vi "FIB MAIN (DESKTOP-J3Q0JMJ's conflicted copy 2019-02-19).vi"() -> ()   [LabVIEW 2018]
uses:
  <vilib>/userdefined/High Color/IMAQdx.ctl
  STAGE POSITION.ctl
  Original FIB Source/CENTER STIGMATOR.ctl
  FIB EVENTS.ctl
  FIB CAMERA EVENTS.ctl
  <vilib>/vision/driver/IMAQdx.llb/IMAQdx Buffer Number Mode.ctl
  <vilib>/vision/driver/IMAQdx.llb/IMAQdx Camera Control Mode.ctl
  <vilib>/Instr/_visa.llb/VISA Flush IO Buffer Mask.ctl
  <vilib>/Utility/error.llb/whitespace.ctl
  Mikrodaq/HYMOD MAIA/ddd.ctl
  FIB STAGE EVENTS.ctl
  <vilib>/Instr/_visa.llb/VISA Configure Serial Port (Instr).vi
  <vilib>/vision/driver/NI_Vision_Acquisition_Software.lvlib
  <resource>/objmgr/imaqdx.rc
  <vilib>/vision/NI_Vision_Development_Module.lvlib
  <vilib>/Utility/Variable/NI_VariableUtilities.lvlib
panel:
  out "size(s) 5":i32
  in  "ENABLE APERTURES":bool
  in  "ENABLE ORSAY":bool=TRUE
  in  "ENABLE CAMERA":bool
  out "size(s) 4":i32
  in  "Tab Control 4":enum32{"COMMANDS", "HV RAMPS"}(tab)
  in  "1V ENERGY RAMP":bool
  out "TEST OUTPUT":string
  in  "TEST COMMAND":bool
  in  "TEST COMMAND":string
  out "SERIAL \nRESPONSE":string[](array[string])
  out "WARNING":string
  out "PROCESS":string
  out "PROCESSES":string[](array[string])
  out "BEAM RAMP":dbl[unit][](graph)
  out "EXTRACTOR RAMP":dbl[unit][](graph)
  out "SUPPRESSOR RAMP":dbl[unit][](graph)
  in  "Tab Control 3":T1(tab)
  out "CURRENT":dbl[unit] format="%_4g"
  out "VOLTAGE":dbl[unit] format="%_4g"
  out "BEAM VOLTAGE":dbl[unit](graph)
  out "BEAM CURRENT":dbl[unit](graph)
  out "VOLTAGE":dbl[unit] format="%_4g"
  out "CURRENT":dbl[unit] format="%_4g"
  out "EXTRACTOR":dbl[unit](graph)
  out "EXTRACTOR  CURRENT":dbl[unit](graph)
  out "VOLTAGE":dbl[unit] format="%_4g"
  out "CURRENT":dbl[unit] format="%_4g"
  out "SUPPRESSOR VOLTAGE":dbl[unit](graph)
  out "SUPPRESSOR CURRENT":dbl[unit](graph)
  out "CONDENSOR VOLTAGE":dbl[unit](graph)
  out "CONDENSOR CURRENT":dbl[unit](graph)
  out "OBJECTIVE VOLTAGE":dbl[unit](graph)
  out "OBJECTIVE CURRENT":dbl[unit](graph)
  out "HV SUPPLY FEEDBACK 13":dbl[unit](graph)
  out "HV SUPPLY FEEDBACK 12":dbl[unit](graph)
  in  "IGAIN":dbl=0.00039 format="%_3p"
  in  "IOFFSET":dbl format="%_4g"
  in  "VOFFSET":dbl format="%_4g"
  out "HEATING CURRENT":dbl
  out "HEATING VOLTAGE":dbl
  in  "VGAIN":dbl=0.00071 format="%_3p"
  in  "OFFSET":dbl
  in  "RPONT":dbl[unit]
  in  "RMES":dbl[unit]
  out "TIMER":u32
  out "size(s)":i32
  out "SUPPRESSOR RAMP":dbl[unit][](array[numeric])
  out "EXTRACTOR RAMP":dbl[unit][](array[numeric])
  out "BEAM RAMP":dbl[unit][](array[numeric])
  in  "MEASURE HV":bool
  out "SERIAL \nRESPONSE 2":string[](array[string])
  out "VISA ERROR":errorcluster
  out "BEAM CURRENT (FC2)":dbl[unit] format="%_4g"
  out "BEAM CURRENT (FC1)":dbl[unit] format="%_4g"
  in  "APERTURE (MASS)":u16(ring)=3 items=["10 um", "20 um", "50 um", "50 um", "100 um", "200 um", "400 um"]
  in  "BRIGHT,CONT,GAMMA":cluster{"B":dbl, "C":dbl, "G":dbl}={"B"=250.0, "C"=67.0, "G"=1.6000000000000005} {"G" format="%_4g"; "C" format="%_4g"; "B" format="%_4g"}
  in  "REFLECTIVITY":bool
  in  "ROTATE VIEW":bool
  in  "ANGLE":sgl format="%.2f"
  in  "IMAGE SYMMETRY":u32(ring)=2 items=["Horizontal", "Vertical", "CENTRAL", "1st Diagonal", "2nd Diagonal"]
  in  "SYMMETRY":bool
  out "FIB CAMERA ERROR":errorcluster
  out "FIB SAMPLE CAMERA":T2="CSIRO-SAMPLE" caption="Session Out"
  out "IMAGE YCENTRE":dbl
  out "IMAGE XCENTRE":dbl
  out "ActualPeakBandwidth":dbl=1000.0
  out "IMAGE YPIXELS":u32=1024
  out "IMAGE XPIXELS":u32=1360
  in  "START SCANNING":bool
  in  "STOP":bool
  out "INTERLOCK STATE":bool
  in  "BEAM ON":bool=TRUE
  in  "BLANKING CONTROL":u16(ring) items=["LOCAL ", "SOURCE", "EXTERNAL"]
  in  "FIB SETUP FILE":path=path "C:/Users/jamie/Desktop/test.tdms"
  in  "SAVE SETUP":bool
  in  "READ & APPLY SETUP":bool
  in  "OBJECT APERTURE":u16(ring)=3 items=["10 um", "20 um", "50 um", "50 um", "100 um", "200 um", "400 um"]
  in  "USER":string="jslaird"
  in  "COMMENT":string
  in  "NAME":string
  out "gamme":bool
  out "Image":T3(plugin-control)
  in  "Tab Control":T4(tab)
  in  "RESET":bool
  in  "INTERLOCK HV":bool
  out "HIGH ENERGY":bool
  in  "SETTINGS DELAY":dbl[unit]=0.2
  in  "dV ENERGY":dbl[unit]=250.0
  in  "dV SUPPRESS":dbl[unit]=50.0
  in  "SHUTDOWN":bool
  in  "FILAMENT":bool
  out "HIGH VOLTAGE SUPPLIES":cluster{dbl[unit], dbl[unit], dbl[unit]}(knob)={0.0, 103.78830891166923, 181.50345045415557} scale format="%#_6p"
  in  "ION GUN":bool
  in  "FILAMENT HEATING":dbl[unit](slide) min=0.0 max=5.0 step=0.1 scale=0.0..5.000000000000001
  in  "ION GUN SETTINGS":T5 {"ION CURRENT" min=0 max=3e-05 step=1e-07; "SUPPRESSOR" min=0 max=30000 step=100; "EXTRACTOR" min=0 max=12000 step=100; "BEAM ENERGY" min=0 max=30000 step=1000}
  in  "dV EXTRACTOR":dbl[unit]=50.0
  in  "MOVE 2 POSITION":T6 {"Z" format="%_4g"; "Y" format="%_4g"; "X" format="%_4g"}
  out "POSITION":T6 {"Z" format="%_4g"; "Y" format="%_4g"; "X" format="%_4g"}
  in  "EXPOSURE":dbl(slide)=106.26827541712952 min=1.0 max=2500.0 step=10.0 scale=5.0..1000.0 scale format="%#_3f"
  out "FIB CAMERA":T3(plugin-control)
  out "IP ADDRESS":string="192.168.1.10"
  in  "CONFIGS":u16(ring) items=["MANUAL", "BEAM FOCUS", "SAMPLE VIEWING"]
  in  "GAIN METHOD":u16(ring)=2 items=["OFF", "ONCE", "CONTINOUS"]
  in  "GAIN":sgl=1.0 min=0 max=31 step=1
  out "CENTRE CAMERA FOV":T7={"Numeric Control"=677, "Numeric Control"=510}
  in  "Tab Control 2":T8(tab)
  out "Yo":dbl format="%_3g"
  out "Xo":dbl format="%_3g"
  in  "STORE OBJECT":bool
  in  "WOBBLER SETTINBGS FOR OBJECT ALIGNMENT":T9={"WOBBLER AMPLITUDE"={0.0, 33.333523, 47.735184}, "WOBBLE"=1} {"WOBBLE" items=["ENERGY", "CONDENSOR", "OBJECTIVE"]; "WOBBLER AMPLITUDE" scale=0.0..100.0}
  in  "OBJ APERTURE ALIGNMENT":T10={"DOWN"=FALSE, "UP"=FALSE, "STEP SIZE"=1, "LEFT"=FALSE, "RIGHT"=FALSE} {"STEP SIZE" items=["1 um", "5 um", "20 um", "50 um", "100 um", "500 um", "2000 um"]}
  in  "TURN ON WOBBLER":bool
  in  "OBJECT APERTURE POSITIONS":cluster{"NAME":string, "Xo":dbl, "Yo":dbl}[](array[cluster])=[{"NAME"="10um", "Xo"=0.0, "Yo"=0.0}, {"NAME"="20um", "Xo"=0.0, "Yo"=0.0}, {"NAME"="50um", "Xo"=0.0, "Yo"=0.0}, {"NAME"="50um", "Xo"=0.0, "Yo"=0.0}, {"NAME"="100um", "Xo"=0.0, "Yo"=0.0}, {"NAME"="200um", "Xo"=0.0, "Yo"=0.0}, {"NAME"="400um", "Xo"=0.0, "Yo"=0.0}] {"Yo" format="%_3g"; "Xo" format="%_3g"}
  in  "MASS APERTURE POSITIONS":cluster{"NAME":string, "Xa":dbl, "Ya":dbl}[](array[cluster])=[{"NAME"="10um", "Xa"=0.0, "Ya"=0.0}, {"NAME"="20um", "Xa"=0.0, "Ya"=0.0}, {"NAME"="50um", "Xa"=0.0, "Ya"=0.0}, {"NAME"="50um", "Xa"=0.0, "Ya"=0.0}, {"NAME"="100um", "Xa"=0.0, "Ya"=0.0}, {"NAME"="200um", "Xa"=0.0, "Ya"=0.0}, {"NAME"="400um", "Xa"=0.0, "Ya"=0.0}] {"Ya" format="%_3g"; "Xa" format="%_3g"}
  in  "MASS APERTURE ALIGNMENT":T10={"DOWN"=FALSE, "UP"=FALSE, "STEP SIZE"=1, "LEFT"=FALSE, "RIGHT"=FALSE} {"STEP SIZE" items=["1 um", "5 um", "20 um", "50 um", "100 um", "500 um", "2000 um"]}
  out "Xa":dbl format="%_3g"
  out "Ya":dbl format="%_3g"
  in  "STORE APERTURE":bool
  out "REFERENCED":bool[](array[boolean])
  out "ON TRARGET":bool[](array[boolean])
  in  "INIT PI":bool
  in  "STAGE AXES":string[](array[string])=["1", "2"]
  out "VELOCITIES":dbl[](array[numeric])
  out "POSITIONS":dbl[](array[numeric]) format="%_5g"
  out "STATUS":bool
  in  "HOME ALL AXES":bool
  in  "AXES MOTIION SETTINGS":dbl[][](array[numeric])=[[1.0, 140.0, 5.0, 350.0, 1200.0, 10000.0, 100.0, 30000.0, 200.0], [2.0, 140.0, 5.0, 350.0, 1200.0, 10000.0, 100.0, 30000.0, 200.0], [3.0, 140.0, 5.0, 0.0, 1200.0, 10000.0, 100.0, 30000.0, 200.0], [4.0, 140.0, 5.0, 0.0, 0.0, 10000.0, 100.0, 30000.0, 200.0]]
  out "NO CONTROLLER":bool
  in  "HOME ON LIMIT":u16(ring) items=["POSITIVE", "NEGATIVE"]
  out "RANGE":dbl[](array[numeric]) format="%_5g"
  in  "STIGMATOR":T11 {"STIG ALIGN"."-Y" min=-100 max=100 step=0.1 scale=-100.0..100.0; "STIG ALIGN"."+Y" min=-100 max=100 step=0.1 scale=-100.0..100.0; "STIG ALIGN"."-X" min=-100 max=100 step=0.1 scale=-100.0..100.0; "STIG ALIGN"."+X" min=-100 max=100 step=0.1 scale=-100.0..100.0; "THETA" format="%_3g"; "OFFY" format="%_3g"; "OFFX" format="%_3g"; "STIG Y" format="%_3g"; "STIG X" format="%_3g"}
  in  "STIGMATOR X & Y":cluster{"X":sgl, "Y":sgl} {"Y" min=0 max=20000 step=100 scale=0.0..1000.0; "X" min=0 max=20 step=0.1 scale=0.0..20.0}
  out "OBJECTIVE":sgl[unit] format="%_4g"
  out "CONDENSOR":sgl[unit] format="%_4g"
  in  "OBJECTIVE":cluster{"COARSE":sgl[unit], "FINE":sgl[unit]} {"FINE" min=0 max=20000 step=100 scale=0.0..1000.0; "COARSE" min=0 max=20000 step=100}
  in  "CONDENSOR":cluster{"COARSE":sgl[unit], "FINE":sgl[unit]} {"FINE" min=0 max=20000 step=100 scale=1.0..1000.0; "COARSE" min=0 max=20000 step=100}
  in  "SCAN CENTRE ON STAGE":T12 {"Zs" format="%_2g"; "Xs" format="%_2g"; "Ys" format="%_2g"}
  in  "STAGE POSITION":T12 {"Zs" format="%_2g"; "Xs" format="%_2g"; "Ys" format="%_2g"}
  in  "SCANNING CLUSTER":T13 {"MAGNIFICATION" scale=-180.0..180.0; "Y-OFFSET" min=0 max=3e-05 step=1e-07; "X-OFFSET" min=0 max=3e-05 step=1e-07; "SCANNING TYPE" items=["EXTERNAL", "ION MILLING"]}
  in  "EXTERNAL SCANNING ROI":T14={"X-AMPLITUDE"=1e-07, "dX"=0.0, "Y-AMPLITUDE"=1e-07, "dY"=0.0} {"Y-AMPLITUDE" min=1e-07 max=0.0005 step=9.999999999999999e-06; "X-AMPLITUDE" min=1e-07 max=0.0005 step=9.999999999999999e-06}
  out "CHAMBER VACUUM":cluster{dbl[unit], dbl[unit]}(knob)={2.179544466940017e-05, 0.00030039245125477424} scale format="%#_2e"
  in  "COLUMN THRESHOLD":dbl[unit]=6.666118421052631e-05
  out "VACUUM STATE":bool
  out "COLUMN VACUUM":dbl[unit](graph)
  out "COLUMN VACUUM":cluster{dbl[unit], dbl[unit]}(knob)={8.118323356328827e-09, 0.00010317996118558537} scale format="%#_1e"
  out "150V GOOD":bool
  in  "CHAMBER THRESHOLD":dbl[unit]
  in  "GATE VALVE":bool=TRUE
  in  "TERMINATION":bool=TRUE
  in  "TERMINATION CHAR":u16(ring)=1 items=["NONE", "CR", "LF", "CR+LF"]
  out "APPEND":string
  out "ORSAY CONNECTED":bool
  in  "STARTUP":T15[](array[typedef])=[enum."OPEN SERIAL CONN TO ORSAY", enum."INITIALISE ORSAY", enum."TURN OFF WOBBLER", enum."VACUUM ", enum."CHECK 150V", enum."BLANKING TOGGLE"]
  out "ORSAY":refnum<visa-resource-name>
  # "EXTRACTOR"
  # "CONDENSOR"
  # "OBJECT\nAPERTURES"
  # "OBJECTIVE"
  # "FILAMENT SHOULD BE ON PRIOR TO GUN !"
  # "E"
  # "C"
  # "O"
  # "AXIS               P                        I                      D                      L                  LOW-VEL    LOW-ACC      HI-VEL          HI-ACC"
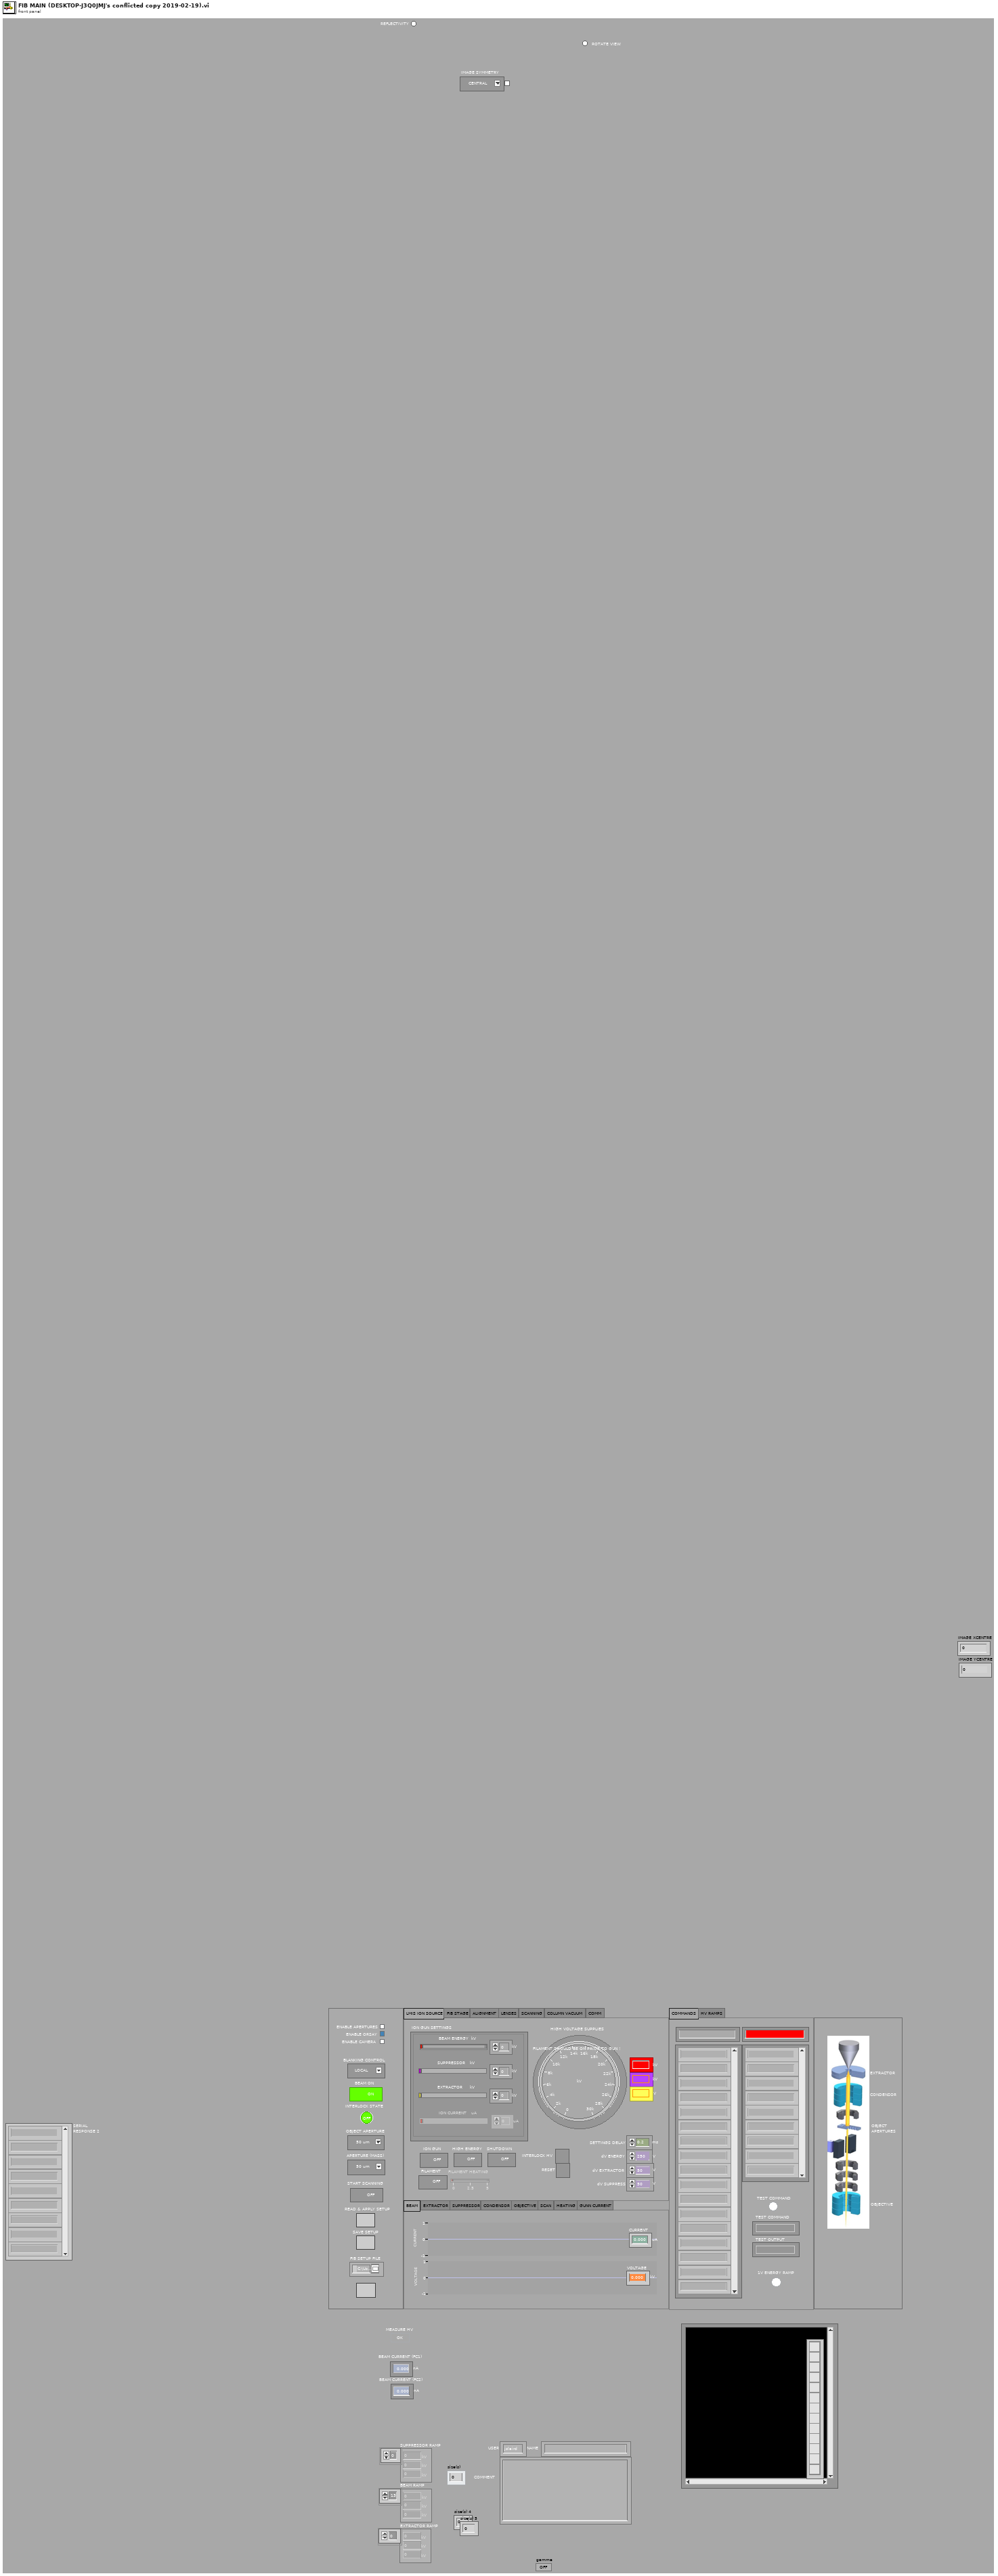
[diagram p1: front panel]
types:
  T1 = enum32{"BEAM", "EXTRACTOR", "SUPPRESSOR", "CONDENSOR", "OBJECTIVE", "SCAN", "HEATING", "GUNN CURRENT"}
  T2 = typedef "IMAQdx.ctl" = refnum<k21>
  T3 = typedef "IMAQ Image.ctl" = refnum<image>
  T4 = enum32{"LMIS ION SOURCE", "FIB STAGE", "ALIGNMENT", "LENSES", "SCANNING", "COLUMN VACUUM", "COMM"}
  T5 = cluster{"BEAM ENERGY":sgl[unit], "SUPPRESSOR":sgl[unit], "EXTRACTOR":sgl[unit], "ION CURRENT":sgl[unit]}
  T6 = typedef "STAGE POSITION.ctl" = cluster{"X":dbl[unit], "Y":dbl[unit], "Z":dbl[unit]}
  T7 = cluster{"Numeric Control":i32, "Numeric Control":i32}
  T8 = enum32{"OBJECTS", "MASS APERTURES", "MOTORS", "CENTRE STIGMATOR"}
  T9 = cluster{"WOBBLER AMPLITUDE":cluster{sgl, sgl, sgl}, "WOBBLE":u16}
  T10 = cluster{"DOWN":bool, "UP":bool, "STEP SIZE":u16, "LEFT":bool, "RIGHT":bool}
  T11 = typedef "CENTER STIGMATOR.ctl" = cluster{"STIG ALIGN":cluster{"+X":sgl, "-X":sgl, "+Y":sgl, "-Y":sgl}, "STIG X":dbl, "OFFX":dbl, "STIG Y":dbl, "OFFY":dbl, "THETA":dbl}
  T12 = cluster{"Xs":dbl[unit], "Ys":dbl[unit], "Zs":dbl[unit]}
  T13 = cluster{"SCANNING TYPE":u16, "X-OFFSET":sgl[unit], "Y-OFFSET":sgl[unit], "ROTATION":dbl[unit], "MAGNIFICATION":dbl}
  T14 = cluster{"X-AMPLITUDE":dbl[unit], "dX":dbl[unit], "Y-AMPLITUDE":dbl[unit], "dY":dbl[unit]}
  T15 = typedef "FIB EVENTS.ctl" = enum16{"LOOP", "OPEN SERIAL CONN TO ORSAY", "INITIALISE ORSAY", "READ SETTINGS", "SAVE SETTINGS", "OBJECTIVE LENS", "CONDENSOR LENS", "BLANKING TOGGLE", "TURN ON HEATER", "TURN OFF WOBBLER", "MEASURE HEATER OUTPUT", "TOGGLE GATE VALVE", "SCANNING CONTROLS", "TURN ON BEAM HV", "ENERGY RAMP CYCLE", "TURN ON SUPPRESSOR", "TURN ON EXTRACTOR", "SET ENERGY RANGE", "MEASURE HV SUPPLY VOLTAGES", "SHUTDOWN ION SOURCE", "RESET TYPE II", "PROBE CURRENT FC#1", "PROBE CURRENT FC#2", "VACUUM ", "CHECK 150V", "INITIALISE PI MOTORS", "SET STIGMATOR", "SET WOBBLER FOR OBJECT", "SET OBJ & AP STAGE VELOCITIES", "READ APERTURE POSITIONS", "HOME OBJ & AP STAGES", "DEFINE NEW OBJ", "MOVE OBJ STAGES", "DEFINE NEW APERTURE", "MOVE APERTURE STAGES", "STOP SYSTEM", "TEST COMMANDS"}
  T16 = typedef "FIB CAMERA EVENTS.ctl" = enum16{"INIT VIDEO", "CAMERA GAIN", "CAMERA EXPOSURE", "LOOP"}
  T17 = enum8{"Enabled", "Disabled", "Disabled and Grayed Out"}
  T18 = cluster{"BEAM ENERGY":sgl[unit], "EXTRACTOR":sgl[unit], "SUPPRESSOR":sgl[unit], "ION CURRENT":sgl[unit]}
  T19 = typedef "FIB STAGE EVENTS.ctl" = enum16{"LOOP", "INIT STAGE CONTROLLER", "SEND COMMAND TO CONTROLLER", "HOME X", "HOME Y", "HOME Z", "ABORT ALL AXES", "GOTO MARKER", "ZERO XYZ", "READ XYZ POSITIONS", "GOTO XYZ POSITION", "STOP", "JOG XYZ", "WAIT FOR MOVE COMPLETE"}
  T20 = cluster{"BEAM":dbl[unit], "SUPPRESSOR":dbl[unit], "EXTRACTOR":dbl[unit]}
  T21 = typedef "ddd.ctl" = string[]
  T22 = enum16{"open", "open or create", "create or replace", "create", "open (read-only)"}
  T23 = typedef "VISA Flush IO Buffer Mask.ctl" = u16
  T24 = cluster{dbl[unit], "CHAMBER THRESHOLD":dbl[unit]}
  T25 = typedef "whitespace.ctl" = u16
  T26 = typedef "NI_Vision_Acquisition_Software.lvlib/IMAQdx Buffer Number Mode.ctl" = enum32{"Next", "Last", "Buffer Number", "Every", "Last New"}
  T27 = typedef "NI_Vision_Acquisition_Software.lvlib/IMAQdx Camera Control Mode.ctl" = enum32{"Controller", "Listener"}
  T28 = typedef "Image Type" = u32
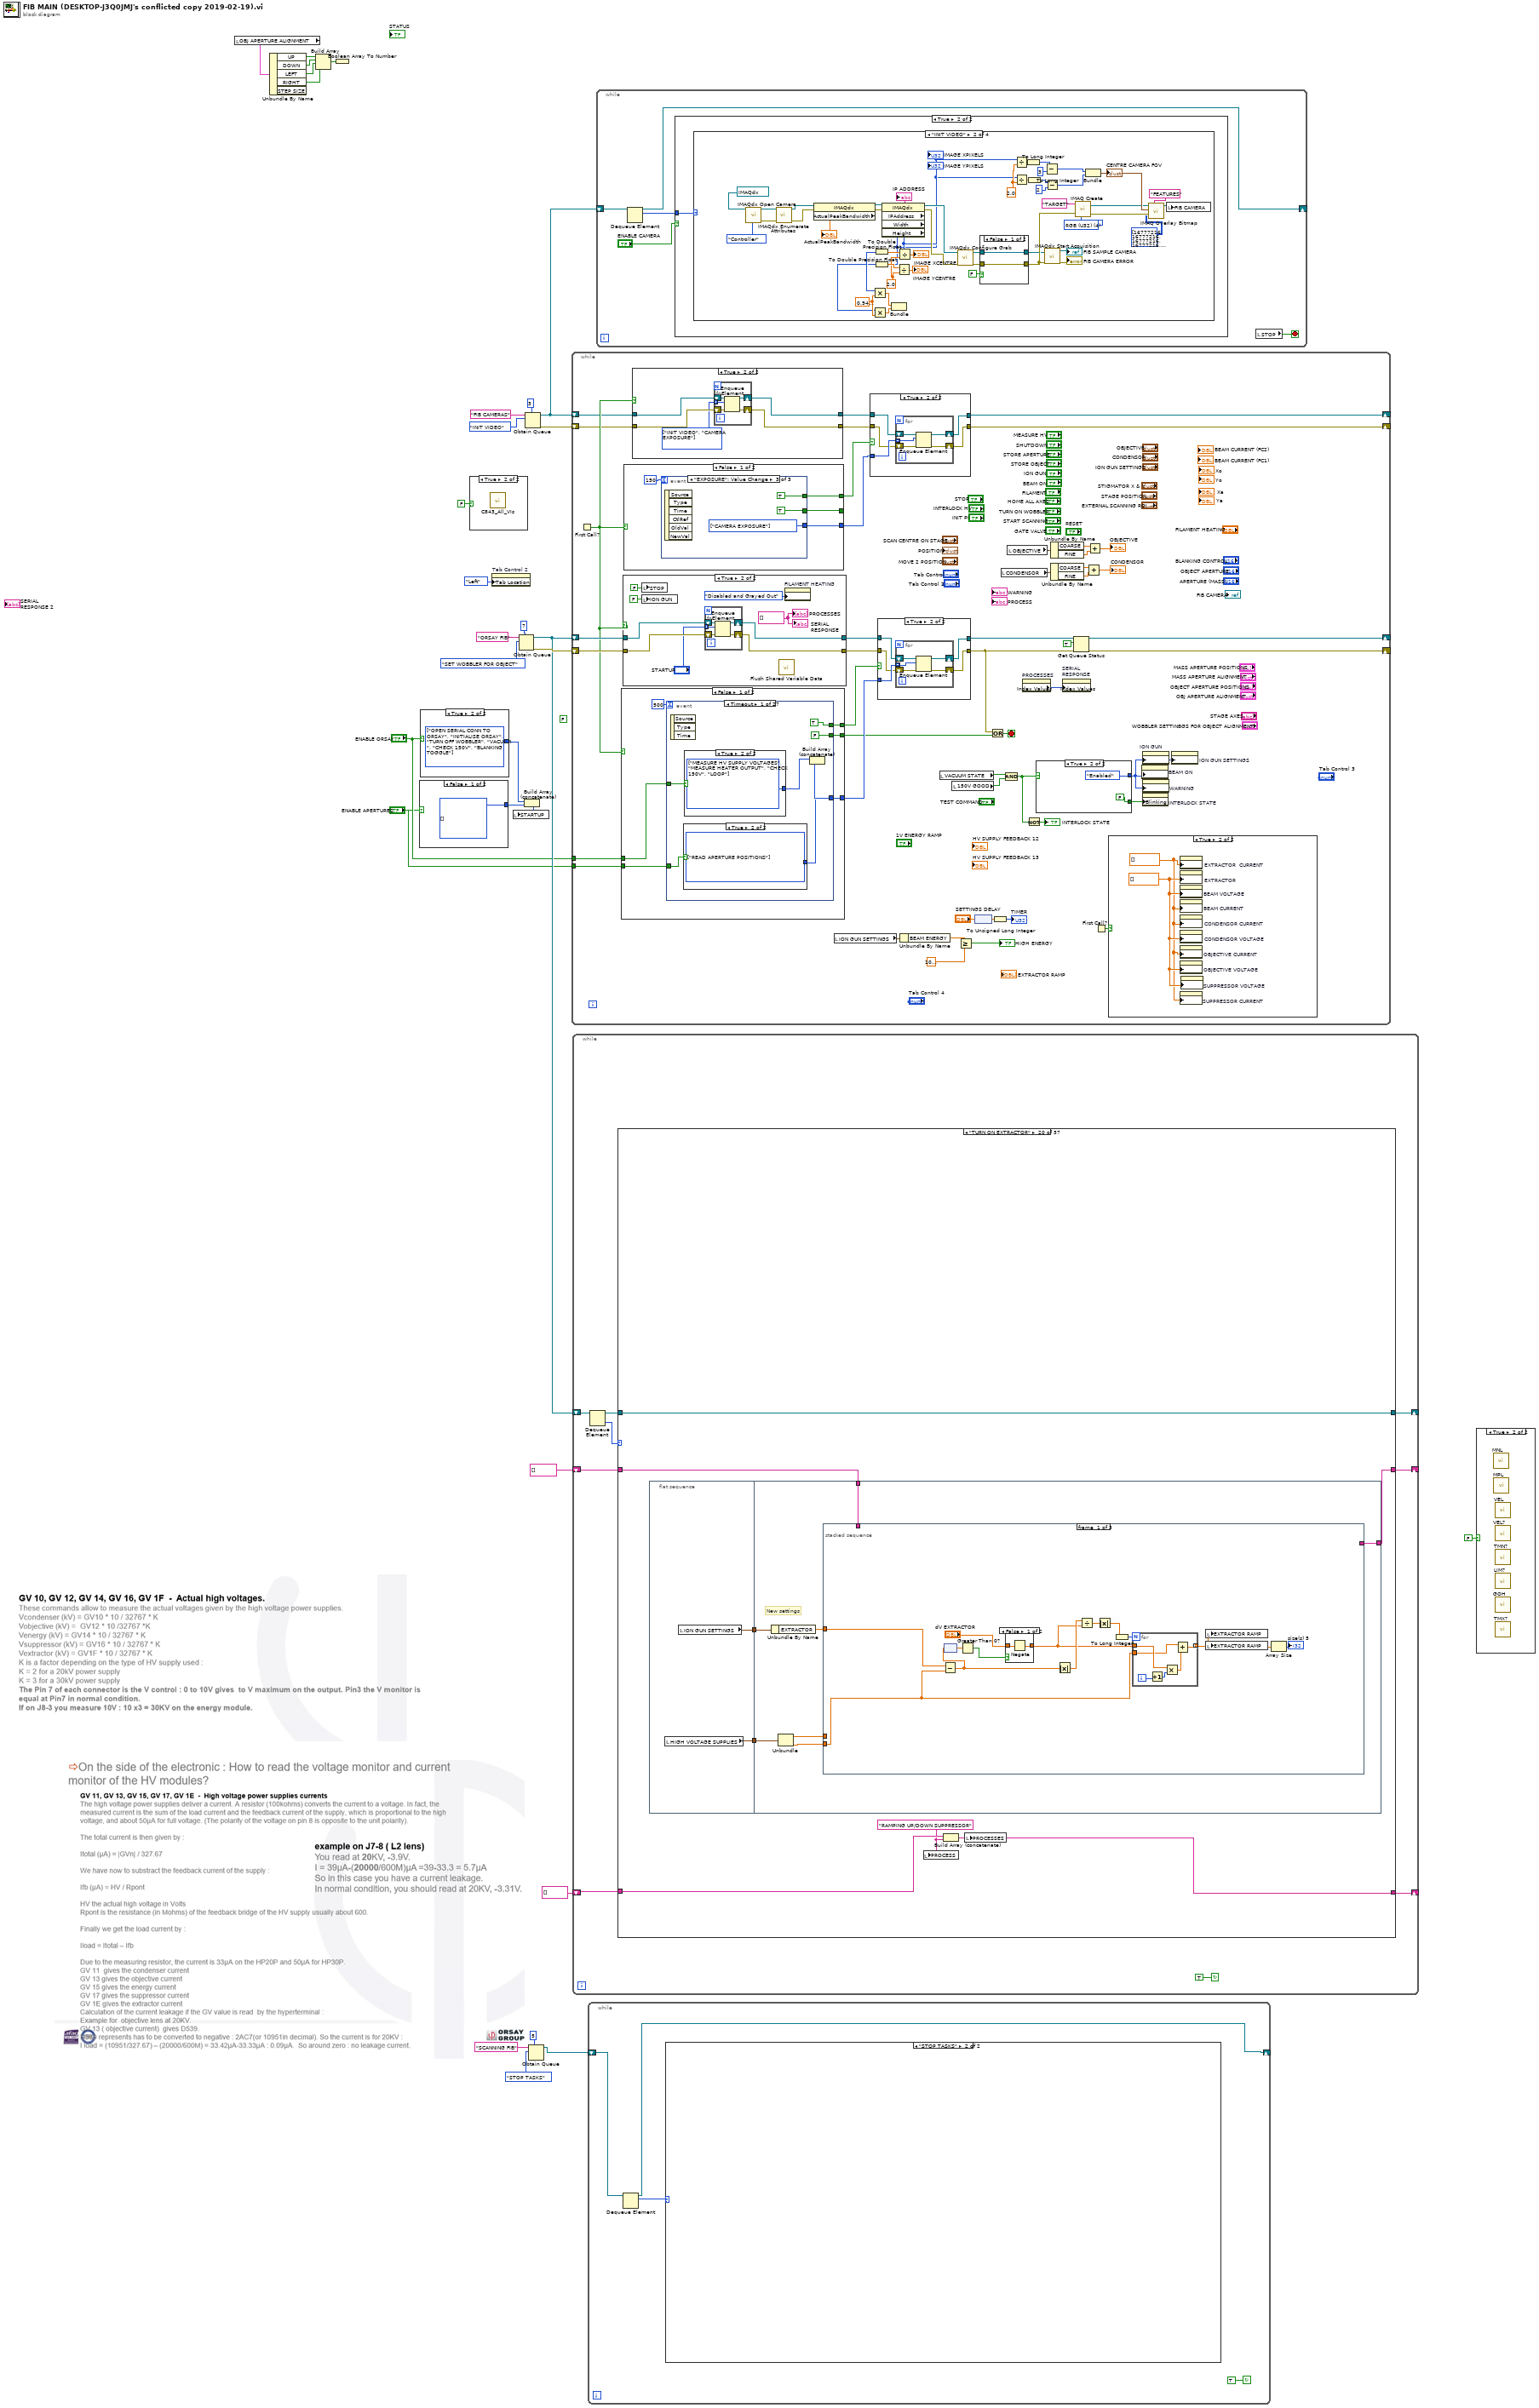
[diagram p0: block diagram]
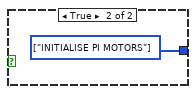
[diagram p2: hidden frame]
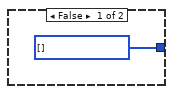
[diagram p3: hidden frame]
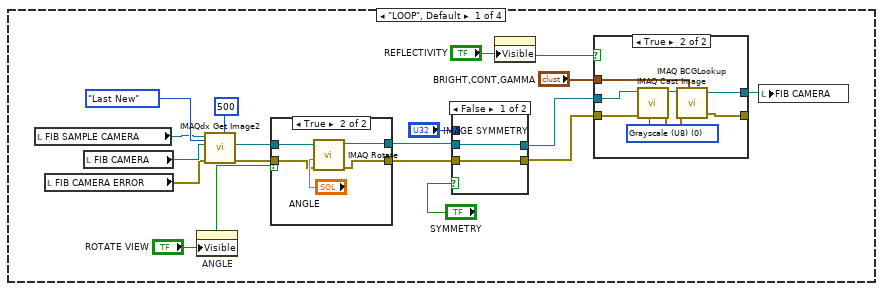
[diagram p8: hidden frame]
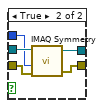
[diagram p11: hidden frame]
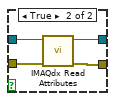
[diagram p12: hidden frame]
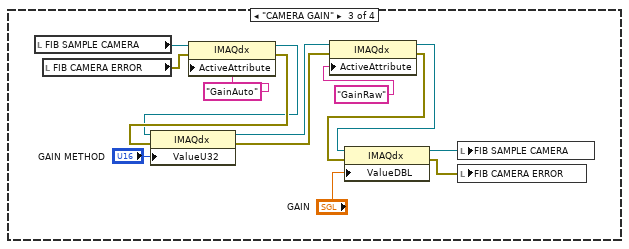
[diagram p13: hidden frame]
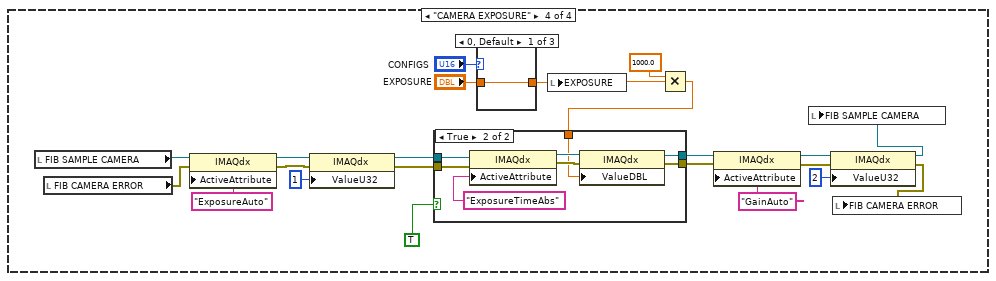
[diagram p14: hidden frame]
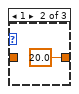
[diagram p16: hidden frame]
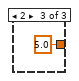
[diagram p17: hidden frame]
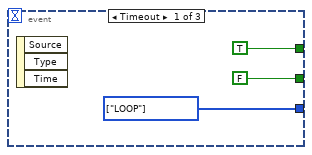
[diagram p20: hidden frame]
diagram:
  (unwired) FALSE ("ION GUN")
  n1 = local read "OBJ APERTURE ALIGNMENT"() -> (w17:T10)
  n2 = Unbundle By Name(w17) -> ("UP"=w18:bool, "DOWN"=w19:bool, "LEFT"=w20:bool, "RIGHT"=w21:bool)  [unwired: 1 out]
  n3 = Build Array(w18, w19, w20, w21) -> (w22:bool[])
  n4 = Boolean Array To Number(Boolean array=w22) -> ()  [unwired: 1 out]
  n5 = case shown="False" "ENABLE APERTURES" {
    tunnel: [w31 w32] -> w4
    frame False {
      w31 = T15[] [] items=["LOOP", "OPEN SERIAL CONN TO ORSAY", "INITIALISE ORSAY", "READ SETTINGS", "SAVE SETTINGS", "OBJECTIVE LENS", "CONDENSOR LENS", "BLANKING TOGGLE", "TURN ON HEATER", "TURN OFF WOBBLER", "MEASURE HEATER OUTPUT", "TOGGLE GATE VALVE", "SCANNING CONTROLS", "TURN ON BEAM HV", "ENERGY RAMP CYCLE", "TURN ON SUPPRESSOR", "TURN ON EXTRACTOR", "SET ENERGY RANGE", "MEASURE HV SUPPLY VOLTAGES", "SHUTDOWN ION SOURCE", "RESET TYPE II", "PROBE CURRENT FC#1", "PROBE CURRENT FC#2", "VACUUM ", "CHECK 150V", "INITIALISE PI MOTORS", "SET STIGMATOR", "SET WOBBLER FOR OBJECT", "SET OBJ & AP STAGE VELOCITIES", "READ APERTURE POSITIONS", "HOME OBJ & AP STAGES", "DEFINE NEW OBJ", "MOVE OBJ STAGES", "DEFINE NEW APERTURE", "MOVE APERTURE STAGES", "STOP SYSTEM", "TEST COMMANDS"] ("STARTUP")
    }
    frame True {
      w32 = T15[] [enum."INITIALISE PI MOTORS"] items=["LOOP", "OPEN SERIAL CONN TO ORSAY", "INITIALISE ORSAY", "READ SETTINGS", "SAVE SETTINGS", "OBJECTIVE LENS", "CONDENSOR LENS", "BLANKING TOGGLE", "TURN ON HEATER", "TURN OFF WOBBLER", "MEASURE HEATER OUTPUT", "TOGGLE GATE VALVE", "SCANNING CONTROLS", "TURN ON BEAM HV", "ENERGY RAMP CYCLE", "TURN ON SUPPRESSOR", "TURN ON EXTRACTOR", "SET ENERGY RANGE", "MEASURE HV SUPPLY VOLTAGES", "SHUTDOWN ION SOURCE", "RESET TYPE II", "PROBE CURRENT FC#1", "PROBE CURRENT FC#2", "VACUUM ", "CHECK 150V", "INITIALISE PI MOTORS", "SET STIGMATOR", "SET WOBBLER FOR OBJECT", "SET OBJ & AP STAGE VELOCITIES", "READ APERTURE POSITIONS", "HOME OBJ & AP STAGES", "DEFINE NEW OBJ", "MOVE OBJ STAGES", "DEFINE NEW APERTURE", "MOVE APERTURE STAGES", "STOP SYSTEM", "TEST COMMANDS"] ("STARTUP")
    }
  }
  n6 = case shown="True" "ENABLE ORSAY" {
    tunnel: [w33 w34] -> w5
    frame False {
      w33 = T15[] [] items=["LOOP", "OPEN SERIAL CONN TO ORSAY", "INITIALISE ORSAY", "READ SETTINGS", "SAVE SETTINGS", "OBJECTIVE LENS", "CONDENSOR LENS", "BLANKING TOGGLE", "TURN ON HEATER", "TURN OFF WOBBLER", "MEASURE HEATER OUTPUT", "TOGGLE GATE VALVE", "SCANNING CONTROLS", "TURN ON BEAM HV", "ENERGY RAMP CYCLE", "TURN ON SUPPRESSOR", "TURN ON EXTRACTOR", "SET ENERGY RANGE", "MEASURE HV SUPPLY VOLTAGES", "SHUTDOWN ION SOURCE", "RESET TYPE II", "PROBE CURRENT FC#1", "PROBE CURRENT FC#2", "VACUUM ", "CHECK 150V", "INITIALISE PI MOTORS", "SET STIGMATOR", "SET WOBBLER FOR OBJECT", "SET OBJ & AP STAGE VELOCITIES", "READ APERTURE POSITIONS", "HOME OBJ & AP STAGES", "DEFINE NEW OBJ", "MOVE OBJ STAGES", "DEFINE NEW APERTURE", "MOVE APERTURE STAGES", "STOP SYSTEM", "TEST COMMANDS"] ("STARTUP")
    }
    frame True {
      w34 = T15[] [enum."OPEN SERIAL CONN TO ORSAY", enum."INITIALISE ORSAY", enum."TURN OFF WOBBLER", enum."VACUUM ", enum."CHECK 150V", enum."BLANKING TOGGLE"] items=["LOOP", "OPEN SERIAL CONN TO ORSAY", "INITIALISE ORSAY", "READ SETTINGS", "SAVE SETTINGS", "OBJECTIVE LENS", "CONDENSOR LENS", "BLANKING TOGGLE", "TURN ON HEATER", "TURN OFF WOBBLER", "MEASURE HEATER OUTPUT", "TOGGLE GATE VALVE", "SCANNING CONTROLS", "TURN ON BEAM HV", "ENERGY RAMP CYCLE", "TURN ON SUPPRESSOR", "TURN ON EXTRACTOR", "SET ENERGY RANGE", "MEASURE HV SUPPLY VOLTAGES", "SHUTDOWN ION SOURCE", "RESET TYPE II", "PROBE CURRENT FC#1", "PROBE CURRENT FC#2", "VACUUM ", "CHECK 150V", "INITIALISE PI MOTORS", "SET STIGMATOR", "SET WOBBLER FOR OBJECT", "SET OBJ & AP STAGE VELOCITIES", "READ APERTURE POSITIONS", "HOME OBJ & AP STAGES", "DEFINE NEW OBJ", "MOVE OBJ STAGES", "DEFINE NEW APERTURE", "MOVE APERTURE STAGES", "STOP SYSTEM", "TEST COMMANDS"] ("STARTUP")
    }
  }
  n7 = case shown="True" FALSE {
    frame False {
    }
    frame True {
      n8 = call "C843_All_VIs.vi"() -> ()  [unwired: 1 in]
    }
  }
  n9 = property on="Tab Control 2" class="TabCtl (strict)"("Tab Location"=enum32{"Top", "Bottom", "Left", "Right"}."Left") -> ()  [unwired: 2 in, 2 out]
  n10 = Obtain Queue(max queue size (-1, unlimited)=7, name (unnamed)="ORSAY FIB", element data type=FIB_EVENTS."SET WOBBLER FOR OBJECT" ("Enum")) -> (queue out=w7:refnum<queue>, error out=w28:errorcluster)  [unwired: 2 in, 1 out]
  n11 = Build Array (concatenate)(w5, w4) -> (w3:T15[])
  n12 = local write "STARTUP"(w3) -> ()
  n13 = Obtain Queue(max queue size (-1, unlimited)=3, name (unnamed)="FIB CAMERAS", element data type=FIB_CAMERA_EVENTS."INIT VIDEO") -> (queue out=w23:refnum<queue>, error out=w24:errorcluster)  [unwired: 2 in, 1 out]
  n14 = Obtain Queue(max queue size (-1, unlimited)=5, name (unnamed)="SCANNING FIB", element data type=enum16{"INIT DAQ", "STOP TASKS"}."STOP TASKS") -> (queue out=w11:refnum<queue>)  [unwired: 2 in, 2 out]
  n15 = while {
    shift-right: [w73] -> _
    shift-left: w7 -> [w81]
    shift-right: [w70] -> _
    shift-left: w28 -> [w80]
    shift-right: [w59] -> _
    shift-left: w23 -> [w65]
    shift-right: [w58] -> _
    shift-left: w24 -> [w64]
    tunnel: "ENABLE ORSAY" -> [w36]
    tunnel: "ENABLE APERTURES" -> [w35]
    stop <- w42 stop-if-true
    n16 = First Call?() -> (First Call?: T/F=w66:bool)
    n17 = case shown="False" w66 {
      tunnel: [w132 FALSE] -> w78
      tunnel: [w131 w242] -> w77
      tunnel: [w130 FALSE] -> w74
      tunnel: w36 -> [w129 _]
      tunnel: w35 -> [w128 _]
      frame False {
        n18 = event shown="[0] Timeout" {
          selector: _ -> [_ _ _ _ _ _ _ _ _ _ _ _ _ _ _ _ _ _ _ _ _ _ _ _ _ _ _]
          dyn-events: _ -> [_ _ _ _ _ _ _ _ _ _ _ _ _ _ _ _ _ _ _ _ _ _ _ _ _ _ _]
          timeout: 500 -> [_ _ _ _ _ _ _ _ _ _ _ _ _ _ _ _ _ _ _ _ _ _ _ _ _ _ _]
          tunnel: [TRUE TRUE ("VACUUM STATE") TRUE ("VACUUM STATE") TRUE ("VACUUM STATE") w156 w158 w164 w168 w175 w182 TRUE ("VACUUM STATE") TRUE ("VACUUM STATE") TRUE ("VACUUM STATE") w196 TRUE ("VACUUM STATE") w201 _ TRUE ("VACUUM STATE") w209 w213 w217 w221 TRUE w227 TRUE ("VACUUM STATE") w234 TRUE ("VACUUM STATE")] -> w132
          tunnel: [FALSE FALSE FALSE FALSE FALSE FALSE FALSE FALSE FALSE FALSE FALSE FALSE FALSE FALSE FALSE FALSE _ FALSE FALSE FALSE FALSE FALSE FALSE FALSE FALSE FALSE FALSE] -> w130
          tunnel: [w137 w147 w148 w153 w154 w162 w165 w171 w178 w180 w185 w188 w191 w194 w200 w204 w205 w206 w212 w216 w220 w223 w226 w228 w230 w233 w236] -> w131
          tunnel: w129 -> [w135 _ _ _ _ _ _ _ _ _ _ _ _ _ _ _ _ _ _ _ _ _ _ _ _ _ _]
          tunnel: w128 -> [w134 _ _ _ _ _ _ _ _ _ _ _ _ _ _ _ _ _ _ _ _ _ _ _ _ _ _]
          event Timeout {
            n19 = event-data() -> ()  [unwired: 1 in, 3 out]
            n20 = case shown="True" w134 {
              tunnel: [w141 w142] -> w136
              frame False {
                w141 = T15[] [] items=["LOOP", "OPEN SERIAL CONN TO ORSAY", "INITIALISE ORSAY", "READ SETTINGS", "SAVE SETTINGS", "OBJECTIVE LENS", "CONDENSOR LENS", "BLANKING TOGGLE", "TURN ON HEATER", "TURN OFF WOBBLER", "MEASURE HEATER OUTPUT", "TOGGLE GATE VALVE", "SCANNING CONTROLS", "TURN ON BEAM HV", "ENERGY RAMP CYCLE", "TURN ON SUPPRESSOR", "TURN ON EXTRACTOR", "SET ENERGY RANGE", "MEASURE HV SUPPLY VOLTAGES", "SHUTDOWN ION SOURCE", "RESET TYPE II", "PROBE CURRENT FC#1", "PROBE CURRENT FC#2", "VACUUM ", "CHECK 150V", "INITIALISE PI MOTORS", "SET STIGMATOR", "SET WOBBLER FOR OBJECT", "SET OBJ & AP STAGE VELOCITIES", "READ APERTURE POSITIONS", "HOME OBJ & AP STAGES", "DEFINE NEW OBJ", "MOVE OBJ STAGES", "DEFINE NEW APERTURE", "MOVE APERTURE STAGES", "STOP SYSTEM", "TEST COMMANDS"]
              }
              frame True {
                w142 = T15[] [enum."READ APERTURE POSITIONS"] items=["LOOP", "OPEN SERIAL CONN TO ORSAY", "INITIALISE ORSAY", "READ SETTINGS", "SAVE SETTINGS", "OBJECTIVE LENS", "CONDENSOR LENS", "BLANKING TOGGLE", "TURN ON HEATER", "TURN OFF WOBBLER", "MEASURE HEATER OUTPUT", "TOGGLE GATE VALVE", "SCANNING CONTROLS", "TURN ON BEAM HV", "ENERGY RAMP CYCLE", "TURN ON SUPPRESSOR", "TURN ON EXTRACTOR", "SET ENERGY RANGE", "MEASURE HV SUPPLY VOLTAGES", "SHUTDOWN ION SOURCE", "RESET TYPE II", "PROBE CURRENT FC#1", "PROBE CURRENT FC#2", "VACUUM ", "CHECK 150V", "INITIALISE PI MOTORS", "SET STIGMATOR", "SET WOBBLER FOR OBJECT", "SET OBJ & AP STAGE VELOCITIES", "READ APERTURE POSITIONS", "HOME OBJ & AP STAGES", "DEFINE NEW OBJ", "MOVE OBJ STAGES", "DEFINE NEW APERTURE", "MOVE APERTURE STAGES", "STOP SYSTEM", "TEST COMMANDS"]
              }
            }
            n21 = case shown="True" w135 {
              tunnel: [w143 w144] -> w138
              frame False {
                w143 = T15[] [] items=["LOOP", "OPEN SERIAL CONN TO ORSAY", "INITIALISE ORSAY", "READ SETTINGS", "SAVE SETTINGS", "OBJECTIVE LENS", "CONDENSOR LENS", "BLANKING TOGGLE", "TURN ON HEATER", "TURN OFF WOBBLER", "MEASURE HEATER OUTPUT", "TOGGLE GATE VALVE", "SCANNING CONTROLS", "TURN ON BEAM HV", "ENERGY RAMP CYCLE", "TURN ON SUPPRESSOR", "TURN ON EXTRACTOR", "SET ENERGY RANGE", "MEASURE HV SUPPLY VOLTAGES", "SHUTDOWN ION SOURCE", "RESET TYPE II", "PROBE CURRENT FC#1", "PROBE CURRENT FC#2", "VACUUM ", "CHECK 150V", "INITIALISE PI MOTORS", "SET STIGMATOR", "SET WOBBLER FOR OBJECT", "SET OBJ & AP STAGE VELOCITIES", "READ APERTURE POSITIONS", "HOME OBJ & AP STAGES", "DEFINE NEW OBJ", "MOVE OBJ STAGES", "DEFINE NEW APERTURE", "MOVE APERTURE STAGES", "STOP SYSTEM", "TEST COMMANDS"]
              }
              frame True {
                w144 = T15[] [enum."MEASURE HV SUPPLY VOLTAGES", enum."MEASURE HEATER OUTPUT", enum."CHECK 150V", enum."LOOP"] items=["LOOP", "OPEN SERIAL CONN TO ORSAY", "INITIALISE ORSAY", "READ SETTINGS", "SAVE SETTINGS", "OBJECTIVE LENS", "CONDENSOR LENS", "BLANKING TOGGLE", "TURN ON HEATER", "TURN OFF WOBBLER", "MEASURE HEATER OUTPUT", "TOGGLE GATE VALVE", "SCANNING CONTROLS", "TURN ON BEAM HV", "ENERGY RAMP CYCLE", "TURN ON SUPPRESSOR", "TURN ON EXTRACTOR", "SET ENERGY RANGE", "MEASURE HV SUPPLY VOLTAGES", "SHUTDOWN ION SOURCE", "RESET TYPE II", "PROBE CURRENT FC#1", "PROBE CURRENT FC#2", "VACUUM ", "CHECK 150V", "INITIALISE PI MOTORS", "SET STIGMATOR", "SET WOBBLER FOR OBJECT", "SET OBJ & AP STAGE VELOCITIES", "READ APERTURE POSITIONS", "HOME OBJ & AP STAGES", "DEFINE NEW OBJ", "MOVE OBJ STAGES", "DEFINE NEW APERTURE", "MOVE APERTURE STAGES", "STOP SYSTEM", "TEST COMMANDS"]
              }
            }
            n22 = Build Array (concatenate)(w138, w136) -> (w137:T15[])
          }
          event "1V ENERGY RAMP": Mouse Down {
            w147 = T15[] [enum."ENERGY RAMP CYCLE"] items=["LOOP", "OPEN SERIAL CONN TO ORSAY", "INITIALISE ORSAY", "READ SETTINGS", "SAVE SETTINGS", "OBJECTIVE LENS", "CONDENSOR LENS", "BLANKING TOGGLE", "TURN ON HEATER", "TURN OFF WOBBLER", "MEASURE HEATER OUTPUT", "TOGGLE GATE VALVE", "SCANNING CONTROLS", "TURN ON BEAM HV", "ENERGY RAMP CYCLE", "TURN ON SUPPRESSOR", "TURN ON EXTRACTOR", "SET ENERGY RANGE", "MEASURE HV SUPPLY VOLTAGES", "SHUTDOWN ION SOURCE", "RESET TYPE II", "PROBE CURRENT FC#1", "PROBE CURRENT FC#2", "VACUUM ", "CHECK 150V", "INITIALISE PI MOTORS", "SET STIGMATOR", "SET WOBBLER FOR OBJECT", "SET OBJ & AP STAGE VELOCITIES", "READ APERTURE POSITIONS", "HOME OBJ & AP STAGES", "DEFINE NEW OBJ", "MOVE OBJ STAGES", "DEFINE NEW APERTURE", "MOVE APERTURE STAGES", "STOP SYSTEM", "TEST COMMANDS"]
            n23 = event-data() -> ()  [unwired: 1 in, 8 out]
          }
          event "RESET": Mouse Down {
            w148 = T15[] [enum."INITIALISE ORSAY"] items=["LOOP", "OPEN SERIAL CONN TO ORSAY", "INITIALISE ORSAY", "READ SETTINGS", "SAVE SETTINGS", "OBJECTIVE LENS", "CONDENSOR LENS", "BLANKING TOGGLE", "TURN ON HEATER", "TURN OFF WOBBLER", "MEASURE HEATER OUTPUT", "TOGGLE GATE VALVE", "SCANNING CONTROLS", "TURN ON BEAM HV", "ENERGY RAMP CYCLE", "TURN ON SUPPRESSOR", "TURN ON EXTRACTOR", "SET ENERGY RANGE", "MEASURE HV SUPPLY VOLTAGES", "SHUTDOWN ION SOURCE", "RESET TYPE II", "PROBE CURRENT FC#1", "PROBE CURRENT FC#2", "VACUUM ", "CHECK 150V", "INITIALISE PI MOTORS", "SET STIGMATOR", "SET WOBBLER FOR OBJECT", "SET OBJ & AP STAGE VELOCITIES", "READ APERTURE POSITIONS", "HOME OBJ & AP STAGES", "DEFINE NEW OBJ", "MOVE OBJ STAGES", "DEFINE NEW APERTURE", "MOVE APERTURE STAGES", "STOP SYSTEM", "TEST COMMANDS"]
            n24 = event-data() -> ()  [unwired: 1 in, 8 out]
          }
          event "MEASURE HV": Mouse Down {
            w153 = T15[] [enum."MEASURE HV SUPPLY VOLTAGES"] items=["LOOP", "OPEN SERIAL CONN TO ORSAY", "INITIALISE ORSAY", "READ SETTINGS", "SAVE SETTINGS", "OBJECTIVE LENS", "CONDENSOR LENS", "BLANKING TOGGLE", "TURN ON HEATER", "TURN OFF WOBBLER", "MEASURE HEATER OUTPUT", "TOGGLE GATE VALVE", "SCANNING CONTROLS", "TURN ON BEAM HV", "ENERGY RAMP CYCLE", "TURN ON SUPPRESSOR", "TURN ON EXTRACTOR", "SET ENERGY RANGE", "MEASURE HV SUPPLY VOLTAGES", "SHUTDOWN ION SOURCE", "RESET TYPE II", "PROBE CURRENT FC#1", "PROBE CURRENT FC#2", "VACUUM ", "CHECK 150V", "INITIALISE PI MOTORS", "SET STIGMATOR", "SET WOBBLER FOR OBJECT", "SET OBJ & AP STAGE VELOCITIES", "READ APERTURE POSITIONS", "HOME OBJ & AP STAGES", "DEFINE NEW OBJ", "MOVE OBJ STAGES", "DEFINE NEW APERTURE", "MOVE APERTURE STAGES", "STOP SYSTEM", "TEST COMMANDS"]
            n25 = event-data() -> ()  [unwired: 1 in, 8 out]
          }
          event "GATE VALVE": Mouse Down {
            w154 = T15[] [enum."TOGGLE GATE VALVE"] items=["LOOP", "OPEN SERIAL CONN TO ORSAY", "INITIALISE ORSAY", "READ SETTINGS", "SAVE SETTINGS", "OBJECTIVE LENS", "CONDENSOR LENS", "BLANKING TOGGLE", "TURN ON HEATER", "TURN OFF WOBBLER", "MEASURE HEATER OUTPUT", "TOGGLE GATE VALVE", "SCANNING CONTROLS", "TURN ON BEAM HV", "ENERGY RAMP CYCLE", "TURN ON SUPPRESSOR", "TURN ON EXTRACTOR", "SET ENERGY RANGE", "MEASURE HV SUPPLY VOLTAGES", "SHUTDOWN ION SOURCE", "RESET TYPE II", "PROBE CURRENT FC#1", "PROBE CURRENT FC#2", "VACUUM ", "CHECK 150V", "INITIALISE PI MOTORS", "SET STIGMATOR", "SET WOBBLER FOR OBJECT", "SET OBJ & AP STAGE VELOCITIES", "READ APERTURE POSITIONS", "HOME OBJ & AP STAGES", "DEFINE NEW OBJ", "MOVE OBJ STAGES", "DEFINE NEW APERTURE", "MOVE APERTURE STAGES", "STOP SYSTEM", "TEST COMMANDS"]
            n26 = event-data() -> ()  [unwired: 1 in, 8 out]
            n27 = local read "INTERLOCK STATE"() -> (w157:bool)
            n28 = Not(x=w157) -> (.not. x?=w156:bool)
          }
          event "ION GUN": Value Change {
            w162 = T15[] [enum."SET ENERGY RANGE", enum."TURN ON BEAM HV", enum."TURN ON SUPPRESSOR", enum."TURN ON EXTRACTOR"] items=["LOOP", "OPEN SERIAL CONN TO ORSAY", "INITIALISE ORSAY", "READ SETTINGS", "SAVE SETTINGS", "OBJECTIVE LENS", "CONDENSOR LENS", "BLANKING TOGGLE", "TURN ON HEATER", "TURN OFF WOBBLER", "MEASURE HEATER OUTPUT", "TOGGLE GATE VALVE", "SCANNING CONTROLS", "TURN ON BEAM HV", "ENERGY RAMP CYCLE", "TURN ON SUPPRESSOR", "TURN ON EXTRACTOR", "SET ENERGY RANGE", "MEASURE HV SUPPLY VOLTAGES", "SHUTDOWN ION SOURCE", "RESET TYPE II", "PROBE CURRENT FC#1", "PROBE CURRENT FC#2", "VACUUM ", "CHECK 150V", "INITIALISE PI MOTORS", "SET STIGMATOR", "SET WOBBLER FOR OBJECT", "SET OBJ & AP STAGE VELOCITIES", "READ APERTURE POSITIONS", "HOME OBJ & AP STAGES", "DEFINE NEW OBJ", "MOVE OBJ STAGES", "DEFINE NEW APERTURE", "MOVE APERTURE STAGES", "STOP SYSTEM", "TEST COMMANDS"]
            n29 = event-data() -> ()  [unwired: 1 in, 6 out]
            n30 = local read "INTERLOCK STATE"() -> (w161:bool)
            n31 = local read "ION GUN"() -> (w159:bool)
            n32 = Not(x=w161) -> (.not. x?=w160:bool)
            n33 = And(x=w160, y=w159) -> (x .and. y?=w158:bool)
          }
          event "INIT PI": Mouse Down {
            w165 = T15[] [enum."INITIALISE PI MOTORS"] items=["LOOP", "OPEN SERIAL CONN TO ORSAY", "INITIALISE ORSAY", "READ SETTINGS", "SAVE SETTINGS", "OBJECTIVE LENS", "CONDENSOR LENS", "BLANKING TOGGLE", "TURN ON HEATER", "TURN OFF WOBBLER", "MEASURE HEATER OUTPUT", "TOGGLE GATE VALVE", "SCANNING CONTROLS", "TURN ON BEAM HV", "ENERGY RAMP CYCLE", "TURN ON SUPPRESSOR", "TURN ON EXTRACTOR", "SET ENERGY RANGE", "MEASURE HV SUPPLY VOLTAGES", "SHUTDOWN ION SOURCE", "RESET TYPE II", "PROBE CURRENT FC#1", "PROBE CURRENT FC#2", "VACUUM ", "CHECK 150V", "INITIALISE PI MOTORS", "SET STIGMATOR", "SET WOBBLER FOR OBJECT", "SET OBJ & AP STAGE VELOCITIES", "READ APERTURE POSITIONS", "HOME OBJ & AP STAGES", "DEFINE NEW OBJ", "MOVE OBJ STAGES", "DEFINE NEW APERTURE", "MOVE APERTURE STAGES", "STOP SYSTEM", "TEST COMMANDS"]
            n34 = event-data() -> ()  [unwired: 1 in, 8 out]
            n35 = local read "INIT PI"() -> (w164:bool)
          }
          event "ION GUN SETTINGS.SUPPRESSOR": Value Change {
            w171 = T15[] [enum."TURN ON SUPPRESSOR"] items=["LOOP", "OPEN SERIAL CONN TO ORSAY", "INITIALISE ORSAY", "READ SETTINGS", "SAVE SETTINGS", "OBJECTIVE LENS", "CONDENSOR LENS", "BLANKING TOGGLE", "TURN ON HEATER", "TURN OFF WOBBLER", "MEASURE HEATER OUTPUT", "TOGGLE GATE VALVE", "SCANNING CONTROLS", "TURN ON BEAM HV", "ENERGY RAMP CYCLE", "TURN ON SUPPRESSOR", "TURN ON EXTRACTOR", "SET ENERGY RANGE", "MEASURE HV SUPPLY VOLTAGES", "SHUTDOWN ION SOURCE", "RESET TYPE II", "PROBE CURRENT FC#1", "PROBE CURRENT FC#2", "VACUUM ", "CHECK 150V", "INITIALISE PI MOTORS", "SET STIGMATOR", "SET WOBBLER FOR OBJECT", "SET OBJ & AP STAGE VELOCITIES", "READ APERTURE POSITIONS", "HOME OBJ & AP STAGES", "DEFINE NEW OBJ", "MOVE OBJ STAGES", "DEFINE NEW APERTURE", "MOVE APERTURE STAGES", "STOP SYSTEM", "TEST COMMANDS"]
            n36 = event-data() -> ()  [unwired: 1 in, 6 out]
            n37 = local read "INTERLOCK STATE"() -> (w170:bool)
            n38 = local read "ION GUN"() -> (w167:bool)
            n39 = Not(x=w170) -> (.not. x?=w169:bool)
            n40 = And(x=w169, y=w167) -> (x .and. y?=w168:bool)
          }
          event "ION GUN SETTINGS.EXTRACTOR": Value Change {
            w178 = T15[] [enum."TURN ON EXTRACTOR"] items=["LOOP", "OPEN SERIAL CONN TO ORSAY", "INITIALISE ORSAY", "READ SETTINGS", "SAVE SETTINGS", "OBJECTIVE LENS", "CONDENSOR LENS", "BLANKING TOGGLE", "TURN ON HEATER", "TURN OFF WOBBLER", "MEASURE HEATER OUTPUT", "TOGGLE GATE VALVE", "SCANNING CONTROLS", "TURN ON BEAM HV", "ENERGY RAMP CYCLE", "TURN ON SUPPRESSOR", "TURN ON EXTRACTOR", "SET ENERGY RANGE", "MEASURE HV SUPPLY VOLTAGES", "SHUTDOWN ION SOURCE", "RESET TYPE II", "PROBE CURRENT FC#1", "PROBE CURRENT FC#2", "VACUUM ", "CHECK 150V", "INITIALISE PI MOTORS", "SET STIGMATOR", "SET WOBBLER FOR OBJECT", "SET OBJ & AP STAGE VELOCITIES", "READ APERTURE POSITIONS", "HOME OBJ & AP STAGES", "DEFINE NEW OBJ", "MOVE OBJ STAGES", "DEFINE NEW APERTURE", "MOVE APERTURE STAGES", "STOP SYSTEM", "TEST COMMANDS"]
            n41 = event-data() -> ()  [unwired: 1 in, 6 out]
            n42 = local read "INTERLOCK STATE"() -> (w177:bool)
            n43 = local read "ION GUN"() -> (w173:bool)
            n44 = Not(x=w177) -> (.not. x?=w174:bool)
            n45 = And(x=w174, y=w173) -> (x .and. y?=w175:bool)
          }
          event "ION GUN SETTINGS.BEAM ENERGY": Value Change {
            w180 = T15[] [enum."TURN ON BEAM HV", enum."TURN ON SUPPRESSOR"] items=["LOOP", "OPEN SERIAL CONN TO ORSAY", "INITIALISE ORSAY", "READ SETTINGS", "SAVE SETTINGS", "OBJECTIVE LENS", "CONDENSOR LENS", "BLANKING TOGGLE", "TURN ON HEATER", "TURN OFF WOBBLER", "MEASURE HEATER OUTPUT", "TOGGLE GATE VALVE", "SCANNING CONTROLS", "TURN ON BEAM HV", "ENERGY RAMP CYCLE", "TURN ON SUPPRESSOR", "TURN ON EXTRACTOR", "SET ENERGY RANGE", "MEASURE HV SUPPLY VOLTAGES", "SHUTDOWN ION SOURCE", "RESET TYPE II", "PROBE CURRENT FC#1", "PROBE CURRENT FC#2", "VACUUM ", "CHECK 150V", "INITIALISE PI MOTORS", "SET STIGMATOR", "SET WOBBLER FOR OBJECT", "SET OBJ & AP STAGE VELOCITIES", "READ APERTURE POSITIONS", "HOME OBJ & AP STAGES", "DEFINE NEW OBJ", "MOVE OBJ STAGES", "DEFINE NEW APERTURE", "MOVE APERTURE STAGES", "STOP SYSTEM", "TEST COMMANDS"]
            n46 = event-data() -> ()  [unwired: 1 in, 6 out]
            n47 = local read "INTERLOCK STATE"() -> (w179:bool)
            n48 = local read "ION GUN"() -> (w184:bool)
            n49 = Not(x=w179) -> (.not. x?=w183:bool)
            n50 = And(x=w183, y=w184) -> (x .and. y?=w182:bool)
          }
          event "TEST COMMAND": Mouse Down {
            w185 = T15[] [enum."TEST COMMANDS"] items=["LOOP", "OPEN SERIAL CONN TO ORSAY", "INITIALISE ORSAY", "READ SETTINGS", "SAVE SETTINGS", "OBJECTIVE LENS", "CONDENSOR LENS", "BLANKING TOGGLE", "TURN ON HEATER", "TURN OFF WOBBLER", "MEASURE HEATER OUTPUT", "TOGGLE GATE VALVE", "SCANNING CONTROLS", "TURN ON BEAM HV", "ENERGY RAMP CYCLE", "TURN ON SUPPRESSOR", "TURN ON EXTRACTOR", "SET ENERGY RANGE", "MEASURE HV SUPPLY VOLTAGES", "SHUTDOWN ION SOURCE", "RESET TYPE II", "PROBE CURRENT FC#1", "PROBE CURRENT FC#2", "VACUUM ", "CHECK 150V", "INITIALISE PI MOTORS", "SET STIGMATOR", "SET WOBBLER FOR OBJECT", "SET OBJ & AP STAGE VELOCITIES", "READ APERTURE POSITIONS", "HOME OBJ & AP STAGES", "DEFINE NEW OBJ", "MOVE OBJ STAGES", "DEFINE NEW APERTURE", "MOVE APERTURE STAGES", "STOP SYSTEM", "TEST COMMANDS"]
            n51 = event-data() -> ()  [unwired: 1 in, 8 out]
          }
          event "INTERLOCK HV": Mouse Down {
            w188 = T15[] [enum."RESET TYPE II"] items=["LOOP", "OPEN SERIAL CONN TO ORSAY", "INITIALISE ORSAY", "READ SETTINGS", "SAVE SETTINGS", "OBJECTIVE LENS", "CONDENSOR LENS", "BLANKING TOGGLE", "TURN ON HEATER", "TURN OFF WOBBLER", "MEASURE HEATER OUTPUT", "TOGGLE GATE VALVE", "SCANNING CONTROLS", "TURN ON BEAM HV", "ENERGY RAMP CYCLE", "TURN ON SUPPRESSOR", "TURN ON EXTRACTOR", "SET ENERGY RANGE", "MEASURE HV SUPPLY VOLTAGES", "SHUTDOWN ION SOURCE", "RESET TYPE II", "PROBE CURRENT FC#1", "PROBE CURRENT FC#2", "VACUUM ", "CHECK 150V", "INITIALISE PI MOTORS", "SET STIGMATOR", "SET WOBBLER FOR OBJECT", "SET OBJ & AP STAGE VELOCITIES", "READ APERTURE POSITIONS", "HOME OBJ & AP STAGES", "DEFINE NEW OBJ", "MOVE OBJ STAGES", "DEFINE NEW APERTURE", "MOVE APERTURE STAGES", "STOP SYSTEM", "TEST COMMANDS"]
            n52 = event-data() -> ()  [unwired: 1 in, 8 out]
          }
          event "STOP": Mouse Down {
            w191 = T15[] [enum."SHUTDOWN ION SOURCE", enum."STOP SYSTEM"] items=["LOOP", "OPEN SERIAL CONN TO ORSAY", "INITIALISE ORSAY", "READ SETTINGS", "SAVE SETTINGS", "OBJECTIVE LENS", "CONDENSOR LENS", "BLANKING TOGGLE", "TURN ON HEATER", "TURN OFF WOBBLER", "MEASURE HEATER OUTPUT", "TOGGLE GATE VALVE", "SCANNING CONTROLS", "TURN ON BEAM HV", "ENERGY RAMP CYCLE", "TURN ON SUPPRESSOR", "TURN ON EXTRACTOR", "SET ENERGY RANGE", "MEASURE HV SUPPLY VOLTAGES", "SHUTDOWN ION SOURCE", "RESET TYPE II", "PROBE CURRENT FC#1", "PROBE CURRENT FC#2", "VACUUM ", "CHECK 150V", "INITIALISE PI MOTORS", "SET STIGMATOR", "SET WOBBLER FOR OBJECT", "SET OBJ & AP STAGE VELOCITIES", "READ APERTURE POSITIONS", "HOME OBJ & AP STAGES", "DEFINE NEW OBJ", "MOVE OBJ STAGES", "DEFINE NEW APERTURE", "MOVE APERTURE STAGES", "STOP SYSTEM", "TEST COMMANDS"]
            n53 = event-data() -> ()  [unwired: 1 in, 8 out]
          }
          event "HIGH ENERGY": Value Change {
            w194 = T15[] [enum."SET ENERGY RANGE"] items=["LOOP", "OPEN SERIAL CONN TO ORSAY", "INITIALISE ORSAY", "READ SETTINGS", "SAVE SETTINGS", "OBJECTIVE LENS", "CONDENSOR LENS", "BLANKING TOGGLE", "TURN ON HEATER", "TURN OFF WOBBLER", "MEASURE HEATER OUTPUT", "TOGGLE GATE VALVE", "SCANNING CONTROLS", "TURN ON BEAM HV", "ENERGY RAMP CYCLE", "TURN ON SUPPRESSOR", "TURN ON EXTRACTOR", "SET ENERGY RANGE", "MEASURE HV SUPPLY VOLTAGES", "SHUTDOWN ION SOURCE", "RESET TYPE II", "PROBE CURRENT FC#1", "PROBE CURRENT FC#2", "VACUUM ", "CHECK 150V", "INITIALISE PI MOTORS", "SET STIGMATOR", "SET WOBBLER FOR OBJECT", "SET OBJ & AP STAGE VELOCITIES", "READ APERTURE POSITIONS", "HOME OBJ & AP STAGES", "DEFINE NEW OBJ", "MOVE OBJ STAGES", "DEFINE NEW APERTURE", "MOVE APERTURE STAGES", "STOP SYSTEM", "TEST COMMANDS"]
            n54 = event-data() -> ()  [unwired: 1 in, 6 out]
            n55 = local read "INTERLOCK STATE"() -> (w197:bool)
            n56 = Not(x=w197) -> (.not. x?=w196:bool)
          }
          event "OBJECT APERTURE": Value Change {
            w200 = T15[] [enum."MOVE OBJ STAGES"] items=["LOOP", "OPEN SERIAL CONN TO ORSAY", "INITIALISE ORSAY", "READ SETTINGS", "SAVE SETTINGS", "OBJECTIVE LENS", "CONDENSOR LENS", "BLANKING TOGGLE", "TURN ON HEATER", "TURN OFF WOBBLER", "MEASURE HEATER OUTPUT", "TOGGLE GATE VALVE", "SCANNING CONTROLS", "TURN ON BEAM HV", "ENERGY RAMP CYCLE", "TURN ON SUPPRESSOR", "TURN ON EXTRACTOR", "SET ENERGY RANGE", "MEASURE HV SUPPLY VOLTAGES", "SHUTDOWN ION SOURCE", "RESET TYPE II", "PROBE CURRENT FC#1", "PROBE CURRENT FC#2", "VACUUM ", "CHECK 150V", "INITIALISE PI MOTORS", "SET STIGMATOR", "SET WOBBLER FOR OBJECT", "SET OBJ & AP STAGE VELOCITIES", "READ APERTURE POSITIONS", "HOME OBJ & AP STAGES", "DEFINE NEW OBJ", "MOVE OBJ STAGES", "DEFINE NEW APERTURE", "MOVE APERTURE STAGES", "STOP SYSTEM", "TEST COMMANDS"]
            n57 = event-data() -> ()  [unwired: 1 in, 6 out]
          }
          event "BEAM ON": Value Change {
            w204 = T15[] [enum."BLANKING TOGGLE"] items=["LOOP", "OPEN SERIAL CONN TO ORSAY", "INITIALISE ORSAY", "READ SETTINGS", "SAVE SETTINGS", "OBJECTIVE LENS", "CONDENSOR LENS", "BLANKING TOGGLE", "TURN ON HEATER", "TURN OFF WOBBLER", "MEASURE HEATER OUTPUT", "TOGGLE GATE VALVE", "SCANNING CONTROLS", "TURN ON BEAM HV", "ENERGY RAMP CYCLE", "TURN ON SUPPRESSOR", "TURN ON EXTRACTOR", "SET ENERGY RANGE", "MEASURE HV SUPPLY VOLTAGES", "SHUTDOWN ION SOURCE", "RESET TYPE II", "PROBE CURRENT FC#1", "PROBE CURRENT FC#2", "VACUUM ", "CHECK 150V", "INITIALISE PI MOTORS", "SET STIGMATOR", "SET WOBBLER FOR OBJECT", "SET OBJ & AP STAGE VELOCITIES", "READ APERTURE POSITIONS", "HOME OBJ & AP STAGES", "DEFINE NEW OBJ", "MOVE OBJ STAGES", "DEFINE NEW APERTURE", "MOVE APERTURE STAGES", "STOP SYSTEM", "TEST COMMANDS"]
            n58 = event-data() -> ()  [unwired: 1 in, 6 out]
            n59 = local read "INTERLOCK STATE"() -> (w202:bool)
            n60 = Not(x=w202) -> (.not. x?=w201:bool)
          }
          event "SHUTDOWN": Mouse Down {
            w205 = T15[] [enum."SHUTDOWN ION SOURCE"] items=["LOOP", "OPEN SERIAL CONN TO ORSAY", "INITIALISE ORSAY", "READ SETTINGS", "SAVE SETTINGS", "OBJECTIVE LENS", "CONDENSOR LENS", "BLANKING TOGGLE", "TURN ON HEATER", "TURN OFF WOBBLER", "MEASURE HEATER OUTPUT", "TOGGLE GATE VALVE", "SCANNING CONTROLS", "TURN ON BEAM HV", "ENERGY RAMP CYCLE", "TURN ON SUPPRESSOR", "TURN ON EXTRACTOR", "SET ENERGY RANGE", "MEASURE HV SUPPLY VOLTAGES", "SHUTDOWN ION SOURCE", "RESET TYPE II", "PROBE CURRENT FC#1", "PROBE CURRENT FC#2", "VACUUM ", "CHECK 150V", "INITIALISE PI MOTORS", "SET STIGMATOR", "SET WOBBLER FOR OBJECT", "SET OBJ & AP STAGE VELOCITIES", "READ APERTURE POSITIONS", "HOME OBJ & AP STAGES", "DEFINE NEW OBJ", "MOVE OBJ STAGES", "DEFINE NEW APERTURE", "MOVE APERTURE STAGES", "STOP SYSTEM", "TEST COMMANDS"]
            n61 = event-data() -> ()  [unwired: 1 in, 8 out]
          }
          event "FILAMENT HEATING", "FILAMENT": Value Change {
            w206 = T15[] [enum."TURN ON HEATER", enum."MEASURE HEATER OUTPUT"] items=["LOOP", "OPEN SERIAL CONN TO ORSAY", "INITIALISE ORSAY", "READ SETTINGS", "SAVE SETTINGS", "OBJECTIVE LENS", "CONDENSOR LENS", "BLANKING TOGGLE", "TURN ON HEATER", "TURN OFF WOBBLER", "MEASURE HEATER OUTPUT", "TOGGLE GATE VALVE", "SCANNING CONTROLS", "TURN ON BEAM HV", "ENERGY RAMP CYCLE", "TURN ON SUPPRESSOR", "TURN ON EXTRACTOR", "SET ENERGY RANGE", "MEASURE HV SUPPLY VOLTAGES", "SHUTDOWN ION SOURCE", "RESET TYPE II", "PROBE CURRENT FC#1", "PROBE CURRENT FC#2", "VACUUM ", "CHECK 150V", "INITIALISE PI MOTORS", "SET STIGMATOR", "SET WOBBLER FOR OBJECT", "SET OBJ & AP STAGE VELOCITIES", "READ APERTURE POSITIONS", "HOME OBJ & AP STAGES", "DEFINE NEW OBJ", "MOVE OBJ STAGES", "DEFINE NEW APERTURE", "MOVE APERTURE STAGES", "STOP SYSTEM", "TEST COMMANDS"]
            n62 = event-data() -> ()  [unwired: 1 in, 6 out]
          }
          event "OBJECTIVE": Value Change {
            w212 = T15[] [enum."OBJECTIVE LENS"] items=["LOOP", "OPEN SERIAL CONN TO ORSAY", "INITIALISE ORSAY", "READ SETTINGS", "SAVE SETTINGS", "OBJECTIVE LENS", "CONDENSOR LENS", "BLANKING TOGGLE", "TURN ON HEATER", "TURN OFF WOBBLER", "MEASURE HEATER OUTPUT", "TOGGLE GATE VALVE", "SCANNING CONTROLS", "TURN ON BEAM HV", "ENERGY RAMP CYCLE", "TURN ON SUPPRESSOR", "TURN ON EXTRACTOR", "SET ENERGY RANGE", "MEASURE HV SUPPLY VOLTAGES", "SHUTDOWN ION SOURCE", "RESET TYPE II", "PROBE CURRENT FC#1", "PROBE CURRENT FC#2", "VACUUM ", "CHECK 150V", "INITIALISE PI MOTORS", "SET STIGMATOR", "SET WOBBLER FOR OBJECT", "SET OBJ & AP STAGE VELOCITIES", "READ APERTURE POSITIONS", "HOME OBJ & AP STAGES", "DEFINE NEW OBJ", "MOVE OBJ STAGES", "DEFINE NEW APERTURE", "MOVE APERTURE STAGES", "STOP SYSTEM", "TEST COMMANDS"]
            n63 = event-data() -> ()  [unwired: 1 in, 6 out]
            n64 = local read "INTERLOCK STATE"() -> (w210:bool)
            n65 = Not(x=w210) -> (.not. x?=w209:bool)
          }
          event "CONDENSOR": Value Change {
            w216 = T15[] [enum."CONDENSOR LENS"] items=["LOOP", "OPEN SERIAL CONN TO ORSAY", "INITIALISE ORSAY", "READ SETTINGS", "SAVE SETTINGS", "OBJECTIVE LENS", "CONDENSOR LENS", "BLANKING TOGGLE", "TURN ON HEATER", "TURN OFF WOBBLER", "MEASURE HEATER OUTPUT", "TOGGLE GATE VALVE", "SCANNING CONTROLS", "TURN ON BEAM HV", "ENERGY RAMP CYCLE", "TURN ON SUPPRESSOR", "TURN ON EXTRACTOR", "SET ENERGY RANGE", "MEASURE HV SUPPLY VOLTAGES", "SHUTDOWN ION SOURCE", "RESET TYPE II", "PROBE CURRENT FC#1", "PROBE CURRENT FC#2", "VACUUM ", "CHECK 150V", "INITIALISE PI MOTORS", "SET STIGMATOR", "SET WOBBLER FOR OBJECT", "SET OBJ & AP STAGE VELOCITIES", "READ APERTURE POSITIONS", "HOME OBJ & AP STAGES", "DEFINE NEW OBJ", "MOVE OBJ STAGES", "DEFINE NEW APERTURE", "MOVE APERTURE STAGES", "STOP SYSTEM", "TEST COMMANDS"]
            n66 = event-data() -> ()  [unwired: 1 in, 6 out]
            n67 = local read "INTERLOCK STATE"() -> (w214:bool)
            n68 = Not(x=w214) -> (.not. x?=w213:bool)
          }
          event "READ & APPLY SETUP": Mouse Down {
            w220 = T15[] [enum."READ SETTINGS"] items=["LOOP", "OPEN SERIAL CONN TO ORSAY", "INITIALISE ORSAY", "READ SETTINGS", "SAVE SETTINGS", "OBJECTIVE LENS", "CONDENSOR LENS", "BLANKING TOGGLE", "TURN ON HEATER", "TURN OFF WOBBLER", "MEASURE HEATER OUTPUT", "TOGGLE GATE VALVE", "SCANNING CONTROLS", "TURN ON BEAM HV", "ENERGY RAMP CYCLE", "TURN ON SUPPRESSOR", "TURN ON EXTRACTOR", "SET ENERGY RANGE", "MEASURE HV SUPPLY VOLTAGES", "SHUTDOWN ION SOURCE", "RESET TYPE II", "PROBE CURRENT FC#1", "PROBE CURRENT FC#2", "VACUUM ", "CHECK 150V", "INITIALISE PI MOTORS", "SET STIGMATOR", "SET WOBBLER FOR OBJECT", "SET OBJ & AP STAGE VELOCITIES", "READ APERTURE POSITIONS", "HOME OBJ & AP STAGES", "DEFINE NEW OBJ", "MOVE OBJ STAGES", "DEFINE NEW APERTURE", "MOVE APERTURE STAGES", "STOP SYSTEM", "TEST COMMANDS"]
            n69 = event-data() -> ()  [unwired: 1 in, 8 out]
            n70 = local read "INTERLOCK STATE"() -> (w218:bool)
            n71 = Not(x=w218) -> (.not. x?=w217:bool)
          }
          event "SCANNING CLUSTER": Value Change {
            w223 = T15[] [enum."SCANNING CONTROLS"] items=["LOOP", "OPEN SERIAL CONN TO ORSAY", "INITIALISE ORSAY", "READ SETTINGS", "SAVE SETTINGS", "OBJECTIVE LENS", "CONDENSOR LENS", "BLANKING TOGGLE", "TURN ON HEATER", "TURN OFF WOBBLER", "MEASURE HEATER OUTPUT", "TOGGLE GATE VALVE", "SCANNING CONTROLS", "TURN ON BEAM HV", "ENERGY RAMP CYCLE", "TURN ON SUPPRESSOR", "TURN ON EXTRACTOR", "SET ENERGY RANGE", "MEASURE HV SUPPLY VOLTAGES", "SHUTDOWN ION SOURCE", "RESET TYPE II", "PROBE CURRENT FC#1", "PROBE CURRENT FC#2", "VACUUM ", "CHECK 150V", "INITIALISE PI MOTORS", "SET STIGMATOR", "SET WOBBLER FOR OBJECT", "SET OBJ & AP STAGE VELOCITIES", "READ APERTURE POSITIONS", "HOME OBJ & AP STAGES", "DEFINE NEW OBJ", "MOVE OBJ STAGES", "DEFINE NEW APERTURE", "MOVE APERTURE STAGES", "STOP SYSTEM", "TEST COMMANDS"]
            n72 = event-data() -> ()  [unwired: 1 in, 6 out]
            n73 = local read "INTERLOCK STATE"() -> (w221:bool)
          }
          event "SAVE SETUP": Mouse Down {
            w226 = T15[] [enum."SAVE SETTINGS"] items=["LOOP", "OPEN SERIAL CONN TO ORSAY", "INITIALISE ORSAY", "READ SETTINGS", "SAVE SETTINGS", "OBJECTIVE LENS", "CONDENSOR LENS", "BLANKING TOGGLE", "TURN ON HEATER", "TURN OFF WOBBLER", "MEASURE HEATER OUTPUT", "TOGGLE GATE VALVE", "SCANNING CONTROLS", "TURN ON BEAM HV", "ENERGY RAMP CYCLE", "TURN ON SUPPRESSOR", "TURN ON EXTRACTOR", "SET ENERGY RANGE", "MEASURE HV SUPPLY VOLTAGES", "SHUTDOWN ION SOURCE", "RESET TYPE II", "PROBE CURRENT FC#1", "PROBE CURRENT FC#2", "VACUUM ", "CHECK 150V", "INITIALISE PI MOTORS", "SET STIGMATOR", "SET WOBBLER FOR OBJECT", "SET OBJ & AP STAGE VELOCITIES", "READ APERTURE POSITIONS", "HOME OBJ & AP STAGES", "DEFINE NEW OBJ", "MOVE OBJ STAGES", "DEFINE NEW APERTURE", "MOVE APERTURE STAGES", "STOP SYSTEM", "TEST COMMANDS"]
            n74 = event-data() -> ()  [unwired: 1 in, 8 out]
          }
          event "WOBBLER SETTINBGS FOR OBJECT ALIGNMENT": Value Change {
            w228 = T15[] [enum."SET WOBBLER FOR OBJECT"] items=["LOOP", "OPEN SERIAL CONN TO ORSAY", "INITIALISE ORSAY", "READ SETTINGS", "SAVE SETTINGS", "OBJECTIVE LENS", "CONDENSOR LENS", "BLANKING TOGGLE", "TURN ON HEATER", "TURN OFF WOBBLER", "MEASURE HEATER OUTPUT", "TOGGLE GATE VALVE", "SCANNING CONTROLS", "TURN ON BEAM HV", "ENERGY RAMP CYCLE", "TURN ON SUPPRESSOR", "TURN ON EXTRACTOR", "SET ENERGY RANGE", "MEASURE HV SUPPLY VOLTAGES", "SHUTDOWN ION SOURCE", "RESET TYPE II", "PROBE CURRENT FC#1", "PROBE CURRENT FC#2", "VACUUM ", "CHECK 150V", "INITIALISE PI MOTORS", "SET STIGMATOR", "SET WOBBLER FOR OBJECT", "SET OBJ & AP STAGE VELOCITIES", "READ APERTURE POSITIONS", "HOME OBJ & AP STAGES", "DEFINE NEW OBJ", "MOVE OBJ STAGES", "DEFINE NEW APERTURE", "MOVE APERTURE STAGES", "STOP SYSTEM", "TEST COMMANDS"]
            n75 = event-data() -> ()  [unwired: 1 in, 6 out]
            n76 = local read "INTERLOCK STATE"() -> (w227:bool)
          }
          event "OBJ APERTURE ALIGNMENT": Value Change {
            w230 = T15[] [enum."MOVE OBJ STAGES"] items=["LOOP", "OPEN SERIAL CONN TO ORSAY", "INITIALISE ORSAY", "READ SETTINGS", "SAVE SETTINGS", "OBJECTIVE LENS", "CONDENSOR LENS", "BLANKING TOGGLE", "TURN ON HEATER", "TURN OFF WOBBLER", "MEASURE HEATER OUTPUT", "TOGGLE GATE VALVE", "SCANNING CONTROLS", "TURN ON BEAM HV", "ENERGY RAMP CYCLE", "TURN ON SUPPRESSOR", "TURN ON EXTRACTOR", "SET ENERGY RANGE", "MEASURE HV SUPPLY VOLTAGES", "SHUTDOWN ION SOURCE", "RESET TYPE II", "PROBE CURRENT FC#1", "PROBE CURRENT FC#2", "VACUUM ", "CHECK 150V", "INITIALISE PI MOTORS", "SET STIGMATOR", "SET WOBBLER FOR OBJECT", "SET OBJ & AP STAGE VELOCITIES", "READ APERTURE POSITIONS", "HOME OBJ & AP STAGES", "DEFINE NEW OBJ", "MOVE OBJ STAGES", "DEFINE NEW APERTURE", "MOVE APERTURE STAGES", "STOP SYSTEM", "TEST COMMANDS"]
            n77 = event-data() -> ()  [unwired: 1 in, 6 out]
          }
          event Value Change {
            w233 = T15[] [enum."SET STIGMATOR"] items=["LOOP", "OPEN SERIAL CONN TO ORSAY", "INITIALISE ORSAY", "READ SETTINGS", "SAVE SETTINGS", "OBJECTIVE LENS", "CONDENSOR LENS", "BLANKING TOGGLE", "TURN ON HEATER", "TURN OFF WOBBLER", "MEASURE HEATER OUTPUT", "TOGGLE GATE VALVE", "SCANNING CONTROLS", "TURN ON BEAM HV", "ENERGY RAMP CYCLE", "TURN ON SUPPRESSOR", "TURN ON EXTRACTOR", "SET ENERGY RANGE", "MEASURE HV SUPPLY VOLTAGES", "SHUTDOWN ION SOURCE", "RESET TYPE II", "PROBE CURRENT FC#1", "PROBE CURRENT FC#2", "VACUUM ", "CHECK 150V", "INITIALISE PI MOTORS", "SET STIGMATOR", "SET WOBBLER FOR OBJECT", "SET OBJ & AP STAGE VELOCITIES", "READ APERTURE POSITIONS", "HOME OBJ & AP STAGES", "DEFINE NEW OBJ", "MOVE OBJ STAGES", "DEFINE NEW APERTURE", "MOVE APERTURE STAGES", "STOP SYSTEM", "TEST COMMANDS"]
            n78 = event-data() -> ()  [unwired: 1 in, 6 out]
            n79 = local read "INTERLOCK STATE"() -> (w234:bool)
          }
          event "HOME ALL AXES": Mouse Down {
            w236 = T15[] [enum."HOME OBJ & AP STAGES"] items=["LOOP", "OPEN SERIAL CONN TO ORSAY", "INITIALISE ORSAY", "READ SETTINGS", "SAVE SETTINGS", "OBJECTIVE LENS", "CONDENSOR LENS", "BLANKING TOGGLE", "TURN ON HEATER", "TURN OFF WOBBLER", "MEASURE HEATER OUTPUT", "TOGGLE GATE VALVE", "SCANNING CONTROLS", "TURN ON BEAM HV", "ENERGY RAMP CYCLE", "TURN ON SUPPRESSOR", "TURN ON EXTRACTOR", "SET ENERGY RANGE", "MEASURE HV SUPPLY VOLTAGES", "SHUTDOWN ION SOURCE", "RESET TYPE II", "PROBE CURRENT FC#1", "PROBE CURRENT FC#2", "VACUUM ", "CHECK 150V", "INITIALISE PI MOTORS", "SET STIGMATOR", "SET WOBBLER FOR OBJECT", "SET OBJ & AP STAGE VELOCITIES", "READ APERTURE POSITIONS", "HOME OBJ & AP STAGES", "DEFINE NEW OBJ", "MOVE OBJ STAGES", "DEFINE NEW APERTURE", "MOVE APERTURE STAGES", "STOP SYSTEM", "TEST COMMANDS"]
            n80 = event-data() -> ()  [unwired: 1 in, 8 out]
          }
        }
      }
      frame True {
        w242 = T19[] [] items=["LOOP", "INIT STAGE CONTROLLER", "SEND COMMAND TO CONTROLLER", "HOME X", "HOME Y", "HOME Z", "ABORT ALL AXES", "GOTO MARKER", "ZERO XYZ", "READ XYZ POSITIONS", "GOTO XYZ POSITION", "STOP", "JOG XYZ", "WAIT FOR MOVE COMPLETE"]
        n81 = local write "ION GUN SETTINGS"(T18 {"BEAM ENERGY"=0.0, "EXTRACTOR"=0.0, "SUPPRESSOR"=0.0, "ION CURRENT"=0.0} ("ION GUN SETTINGS")) -> ()
      }
    }
    n82 = case shown="True" w66 {
      tunnel: w81 -> [w256 w265]
      tunnel: w80 -> [w255 w264]
      tunnel: [w256 w263] -> w79
      tunnel: [w255 w262] -> w76
      frame False {
      }
      frame True {
        w259 = string[] [] ("PROCESSES")
        n83 = local write "STOP"(FALSE ("STOP")) -> ()
        n84 = local write "ION GUN"(FALSE ("TURN ON GUN")) -> ()
        n85 = for {
          shift-right: [w268] -> w263
          shift-left: w265 -> [w270]
          shift-right: [w267] -> w262
          shift-left: w264 -> [w269]
          tunnel: "STARTUP" -> [w266] mode=indexing
          n86 = Enqueue Element(queue=w270, element=w266, error in (no error)=w269) -> (queue out=w268:refnum<queue>, error out=w267:errorcluster)  [unwired: 1 in, 1 out]
        }
        n87 = call <vilib>:"Flush Shared Variable Data.vi"() -> ()  [unwired: 11 in, 1 out]
        n88 = property on="FILAMENT HEATING" class="Slide (strict)"("DisabledEnum"=T17."Disabled and Grayed Out" ("Disabled")) -> ()  [unwired: 2 in, 2 out]
        "PROCESSES" <- w259
        "SERIAL \nRESPONSE" <- w259
      }
    }
    n89 = case shown="False" w66 {
      tunnel: [w98 FALSE] -> w61
      tunnel: [w97 w109] -> w60
      tunnel: [w96 FALSE] -> _
      frame False {
        n90 = event shown="[2] \"EXPOSURE\": Value Change" {
          selector: _ -> [_ _ _]
          dyn-events: _ -> [_ _ _]
          timeout: 150 -> [_ _ _]
          tunnel: [TRUE TRUE TRUE] -> w98
          tunnel: [FALSE TRUE TRUE] -> w96
          tunnel: [w100 w105 w108] -> w97
          event Timeout {
            w100 = T16[] [enum."LOOP"] items=["INIT VIDEO", "CAMERA GAIN", "CAMERA EXPOSURE", "LOOP"]
            n91 = event-data() -> ()  [unwired: 1 in, 3 out]
          }
          event "GAIN", "GAIN METHOD": Value Change {
            w105 = T16[] [enum."CAMERA GAIN"] items=["INIT VIDEO", "CAMERA GAIN", "CAMERA EXPOSURE", "LOOP"]
            n92 = event-data() -> ()  [unwired: 1 in, 6 out]
          }
          event "EXPOSURE": Value Change {
            w108 = T16[] [enum."CAMERA EXPOSURE"] items=["INIT VIDEO", "CAMERA GAIN", "CAMERA EXPOSURE", "LOOP"]
            n93 = event-data() -> ()  [unwired: 1 in, 6 out]
          }
        }
      }
      frame True {
        w109 = T16[] [] items=["INIT VIDEO", "CAMERA GAIN", "CAMERA EXPOSURE", "LOOP"]
      }
    }
    n94 = case shown="True" w66 {
      tunnel: w65 -> [w113 w118]
      tunnel: w64 -> [w112 w117]
      tunnel: [w113 w116] -> w63
      tunnel: [w112 w115] -> w62
      frame False {
      }
      frame True {
        w114 = T16[] [enum."INIT VIDEO", enum."CAMERA EXPOSURE"] items=["INIT VIDEO", "CAMERA GAIN", "CAMERA EXPOSURE", "LOOP"]
        n95 = for {
          shift-right: [w121] -> w116
          shift-left: w118 -> [w123]
          shift-right: [w120] -> w115
          shift-left: w117 -> [w122]
          tunnel: w114 -> [w119] mode=indexing
          n96 = Enqueue Element(queue=w123, element=w119, error in (no error)=w122) -> (queue out=w121:refnum<queue>, error out=w120:errorcluster)  [unwired: 1 in, 1 out]
        }
      }
    }
    n97 = local read "ION GUN SETTINGS"() -> (w45:T5)
    n98 = case shown="True" w61 {
      tunnel: w63 -> [w85 w90]
      tunnel: w60 -> [_ w89]
      tunnel: [w85 w88] -> w59
      tunnel: [w84 w87] -> w58
      tunnel: w62 -> [w84 w86]
      frame False {
      }
      frame True {
        n99 = for {
          shift-right: [w93] -> w88
          shift-left: w90 -> [w95]
          shift-right: [w92] -> w87
          shift-left: w86 -> [w94]
          tunnel: w89 -> [w91] mode=indexing
          n100 = Enqueue Element(queue=w95, element=w91, error in (no error)=w94) -> (queue out=w93:refnum<queue>, error out=w92:errorcluster)  [unwired: 1 in, 1 out]
        }
      }
    }
    n101 = case shown="True" w78 {
      tunnel: w79 -> [w244 w249]
      tunnel: w77 -> [_ w248]
      tunnel: [w244 w247] -> w75
      tunnel: [w243 w246] -> w72
      tunnel: w76 -> [w243 w245]
      frame False {
      }
      frame True {
        n102 = for {
          shift-right: [w252] -> w247
          shift-left: w249 -> [w254]
          shift-right: [w251] -> w246
          shift-left: w245 -> [w253]
          tunnel: w248 -> [w250] mode=indexing
          n103 = Enqueue Element(queue=w254, element=w250, error in (no error)=w253) -> (queue out=w252:refnum<queue>, error out=w251:errorcluster)  [unwired: 1 in, 1 out]
        }
      }
    }
    n104 = Unbundle By Name(w45) -> ("BEAM ENERGY"=w37:sgl[unit])
    n105 = local read "VACUUM STATE"() -> (w68:bool)
    n106 = local read "150V GOOD"() -> (w69:bool)
    n107 = Greater Or Equal?(x=w37, y=sgl[unit] 10000.0) -> (x >= y?=→"HIGH ENERGY":bool)
    n108 = node("SETTINGS DELAY") -> (w40:dbl)
    n109 = Or(x=w72, y=w74) -> (x .or. y?=w42:bool)
    n110 = To Unsigned Long Integer(number=w40) -> (unsigned 32bit integer=→"TIMER":u32)
    n111 = local read "CONDENSOR"() -> (w47:cluster{"COARSE":sgl[unit], "FINE":sgl[unit]})
    n112 = Compound Arithmetic op=AND(w68, w69) -> (w55:bool)
    n113 = local read "OBJECTIVE"() -> (w46:cluster{"COARSE":sgl[unit], "FINE":sgl[unit]})
    n114 = property on="PROCESSES" class="Arr (strict)"() -> ("Index Values"=w54:u32[])  [unwired: 2 in, 2 out]
    n115 = Not(x=w55) -> (.not. x?=→"INTERLOCK STATE":bool)
    n116 = case shown="True" w55 {
      tunnel: [T17."Disabled and Grayed Out" ("Disabled") T17."Enabled" ("Disabled")] -> w57
      tunnel: [TRUE FALSE] -> w67
      frame False {
      }
      frame True {
      }
    }
    n117 = Unbundle By Name(w46) -> ("COARSE"=w49:sgl[unit], "FINE"=w48:sgl[unit])
    n118 = Unbundle By Name(w47) -> ("COARSE"=w50:sgl[unit], "FINE"=w51:sgl[unit])
    n119 = property on="SERIAL \nRESPONSE" class="Arr (strict)"("Index Values"=w54) -> ()  [unwired: 2 in, 2 out]
    n120 = Get Queue Status(queue=w75, return elements? (F)=TRUE, error in (no error)=w72) -> (queue out=w73:refnum<queue>, error out=w70:errorcluster)  [unwired: 6 out]
    n121 = Add(x=w50, y=w51) -> (x+y=→"CONDENSOR":sgl[unit])
    n122 = Add(x=w49, y=w48) -> (x+y=→"OBJECTIVE":sgl[unit])
    n123 = First Call?() -> (First Call?: T/F=w41:bool)
    n124 = case shown="True" w41 {
      frame False {
      }
      frame True {
        w82 = dbl[unit][] [] ("History Data")
        w83 = dbl[unit][] [] ("History Data")
        n125 = property on="BEAM VOLTAGE" class="WFChart (strict)"("History Data"=w83) -> ()  [unwired: 2 in, 2 out]
        n126 = property on="BEAM CURRENT" class="WFChart (strict)"("History Data"=w82) -> ()  [unwired: 2 in, 2 out]
        n127 = property on="EXTRACTOR  CURRENT" class="WFChart (strict)"("History Data"=w82) -> ()  [unwired: 2 in, 2 out]
        n128 = property on="EXTRACTOR" class="WFChart (strict)"("History Data"=w83) -> ()  [unwired: 2 in, 2 out]
        n129 = property on="CONDENSOR CURRENT" class="WFChart (strict)"("History Data"=w82) -> ()  [unwired: 2 in, 2 out]
        n130 = property on="CONDENSOR VOLTAGE" class="WFChart (strict)"("History Data"=w83) -> ()  [unwired: 2 in, 2 out]
        n131 = property on="OBJECTIVE CURRENT" class="WFChart (strict)"("History Data"=w82) -> ()  [unwired: 2 in, 2 out]
        n132 = property on="OBJECTIVE VOLTAGE" class="WFChart (strict)"("History Data"=w83) -> ()  [unwired: 2 in, 2 out]
        n133 = property on="SUPPRESSOR CURRENT" class="WFChart (strict)"("History Data"=w82) -> ()  [unwired: 2 in, 2 out]
        n134 = property on="SUPPRESSOR VOLTAGE" class="WFChart (strict)"("History Data"=w83) -> ()  [unwired: 2 in, 2 out]
      }
    }
    n135 = property on="BEAM ON" class="Bool (strict)"("DisabledEnum"=w57) -> ()  [unwired: 2 in, 2 out]
    n136 = property on="ION GUN" class="Bool (strict)"("DisabledEnum"=w57) -> ()  [unwired: 2 in, 2 out]
    n137 = property on="WARNING" class="Str"("DisabledEnum"=w57) -> ()  [unwired: 2 in, 2 out]
    n138 = property on="INTERLOCK STATE" class="Bool (strict)"("Blinking"=w67) -> ()  [unwired: 2 in, 2 out]
    n139 = property on="ION GUN SETTINGS" class="Clust (strict)"("DisabledEnum"=w57) -> ()  [unwired: 2 in, 2 out]
  }
  n140 = while {
    shift-right: [w277] -> _
    shift-left: string[] [] -> [w278]
    shift-right: [w272] -> _
    shift-left: string[] [] -> [w276]
    shift-right: [w275] -> _
    shift-left: w7 -> [w273]
    stop <- TRUE continue-if-true
    n141 = Dequeue Element(queue=w273) -> (queue out=w274:refnum<queue>, element=w279:T15)  [unwired: 2 in, 2 out]
    n142 = case shown="\"TURN ON EXTRACTOR\"" w279 {
      tunnel: w278 -> [w287 w318 w375 w406 w433 w517 w536 w580 w635 w649 w654 w665 w712 w762 w793 w823 w848 w924 w955 w1035 w1112 w1131 w1168 w1175 w1220 w1365 w1425 w1472 w1488 w1492 w1504 w1517 w1547 w1554 w1557 w1570 w1592]
      tunnel: [w285 w316 w373 w406 w432 w515 w535 w581 w635 w650 w654 w662 w711 w761 w792 w823 w847 w924 w954 w1034 w1112 w1131 w1167 w1173 w1220 w1365 w1422 w1470 w1488 w1492 w1504 w1517 w1546 w1554 w1557 w1570 w1592] -> w277
      tunnel: w276 -> [w284 w314 w376 w405 w431 w513 w534 w582 w633 w637 w652 w664 w749 w760 w794 w835 w850 w925 w957 w1037 w1113 w1133 w1165 w1176 w1218 w1363 w1423 w1473 w1486 w1490 w1502 w1515 w1550 w1552 w1555 w1568 w1590]
      tunnel: [w281 w312 w371 w405 w426 w507 w531 w570 w633 w637 w652 w659 w749 w757 w787 w820 w849 w925 w956 w1036 w1113 w1133 w1165 w1170 w1218 w1363 w1420 w1468 w1486 w1490 w1502 w1515 w1549 w1552 w1555 w1568 w1590] -> w272
      tunnel: [w282 w313 w372 w404 w427 w527 w532 w572 w634 w647 w653 w660 w750 w758 w788 w822 w845 w926 w952 w1032 w1111 w1132 w1166 w1171 w1219 w1364 w1421 w1469 w1487 w1491 w1503 w1516 w1551 w1553 w1556 w1569 w1591] -> w275
      tunnel: w274 -> [w282 w313 w372 w404 w428 w527 w532 w572 w634 w647 w653 w660 w750 w758 w788 w822 w845 w926 w952 w1032 w1111 w1132 w1166 w1171 w1219 w1364 w1421 w1469 w1487 w1491 w1503 w1516 w1551 w1553 w1556 w1569 w1591]
      frame "LOOP", Default {
        w280 = dbl[unit][] [] ("EXTRACTOR RAMP")
        w286 = "LOOP" ("PROCESS")
        n143 = local read "WOBBLER SETTINBGS FOR OBJECT ALIGNMENT"() -> (w290:T9)
        n144 = case shown="False" FALSE {
          frame False {
          }
          frame True {
            w294 = T23 16 items=["Flush Receive Buffer"=16, "Write Transmit Buffer to Device"=32, "Flush Receive Buffer (No I/O)"=64, "Flush Transmit Buffer"=128] ("Mask")
            n145 = local read "NO CONTROLLER"() -> (w299:bool)
            n146 = case shown="False" w299 {
              frame False {
                # "Query position for selected\naxes, not for all axes"
                n147 = call "POS?.vi"("System no."=1, "All axes?"=TRUE) -> ("Position"=w300:dbl[])  [unwired: 3 in, 14 out]
                n148 = local write "POSITIONS"(w300) -> ()
              }
              frame True {
              }
            }
            n149 = local read "VISA ERROR"() -> (w297:errorcluster)
            n150 = local read "ORSAY"() -> (w296:refnum<visa-resource-name>)
            n151 = VISA Flush I/O Buffer(VISA resource name=w296, mask (16)=w294, error in (no error)=w297) -> (VISA resource name out=w295:refnum<visa-resource-name>, error out=w298:errorcluster)
            n152 = local write "ORSAY"(w295) -> ()
            n153 = local write "VISA ERROR"(w298) -> ()
          }
        }
        n154 = local write "BEAM RAMP"(w280) -> ()
        n155 = local write "SUPPRESSOR RAMP"(w280) -> ()
        n156 = local write "EXTRACTOR RAMP"(w280) -> ()
        n157 = Unbundle By Name(w290) -> ("WOBBLE"=w289:u16)
        n158 = local write "PROCESS"(w286) -> ()
        n159 = case shown="1" w289 {
          tunnel: [TRUE FALSE FALSE] -> w293
          tunnel: [FALSE TRUE FALSE] -> w292
          tunnel: [FALSE FALSE TRUE] -> w291
          frame 0, Default {
          }
          frame 1 {
          }
          frame 2 {
          }
        }
        n160 = Build Array (concatenate)(w287, w286) -> (w285:string[])
        n161 = property class="DigNum (strict)"("Blinking"=w293) -> ()  [unwired: 2 in, 2 out]
        n162 = property class="DigNum (strict)"("Blinking"=w292) -> ()  [unwired: 2 in, 2 out]
        n163 = property class="DigNum (strict)"("Blinking"=w291) -> ()  [unwired: 2 in, 2 out]
        n164 = local write "PROCESSES"(w285) -> ()
        n165 = Build Array (concatenate)(w284, "LOOP") -> (w281:string[])
        n166 = local write "SERIAL \nRESPONSE"(w281) -> ()
      }
      frame "OPEN SERIAL CONN TO ORSAY" {
        w317 = "OPENING SERIAL CONNECTION TO ORSAY MB" ("PROCESS")
        n167 = flat-sequence {
          tunnel: [w330] -> w315
          frame #0 {
            w322 = T23 128 items=["Flush Receive Buffer"=16, "Write Transmit Buffer to Device"=32, "Flush Receive Buffer (No I/O)"=64, "Flush Transmit Buffer"=128] ("Mask")
            w339 = T23 16 items=["Flush Receive Buffer"=16, "Write Transmit Buffer to Device"=32, "Flush Receive Buffer (No I/O)"=64, "Flush Transmit Buffer"=128] ("Mask")
            n168 = case shown="0, Default" "TERMINATION CHAR" {
              tunnel: [0 13 10] -> w328
              tunnel: [w351 w354 w359] -> w327
              tunnel: [w350 w353 w358] -> w326
              tunnel: ["" "\r" "\n"] -> w319
              frame 0, Default {
                w350 = u16 0 items=["None", "Last Bit", "TermChar"] ("Serial Settings:End Mode for Reads")
                w351 = u16 0 items=["None", "Last Bit", "TermChar"] ("Serial Settings:End Mode for Reads")
              }
              frame 1 {
                w353 = u16 0 items=["None", "Last Bit", "TermChar"] ("Serial Settings:End Mode for Reads")
                w354 = u16 2 items=["None", "Last Bit", "TermChar"] ("Serial Settings:End Mode for Reads")
              }
              frame 2 {
                w358 = u16 0 items=["None", "Last Bit", "TermChar"] ("Serial Settings:End Mode for Reads")
                w359 = u16 2 items=["None", "Last Bit", "TermChar"] ("Serial Settings:End Mode for Reads")
              }
            }
            "APPEND" <- w319
            n169 = call-poly "VISA Configure Serial Port"("VISA resource name"=refnum<visa-resource-name> "ORSAY-USB", "Enable Termination\nChar (T)"=FALSE ("Enable Termination\nChar (T)"), "baud rate (9600)"=9600) -> ("VISA resource name out"=w343:refnum<visa-resource-name>, "error out"=w342:errorcluster)  [unwired: 11 in]
            n170 = property class="Instr"(reference=w343, error in=w342, "Serial Settings:End Mode for Writes"=w327, "Message Based Settings:Send End Enable"="TERMINATION", "Message Based Settings:Termination Character"=w328, "ASRL End In"=w326) -> (reference out=w334:refnum<visa-resource-name>, error out=w332:errorcluster)
            n171 = flat-sequence {
              tunnel: [w362] -> w333
              tunnel: w334 -> [w362]
              tunnel: [w361] -> w331
              tunnel: w332 -> [w361]
              frame #0 {
                n172 = Wait (ms)(milliseconds to wait=u32 200) -> ()  [unwired: 1 out]
              }
            }
            n173 = property class="Instr"(reference=w333, error in=w331) -> (reference out=w338:refnum<visa-resource-name>, error out=w335:errorcluster, "Serial Settings:Number of Bytes at Serial Port"=w336:u32)
            n174 = VISA Read(VISA resource name=w338, byte count=w336, error in (no error)=w335) -> (VISA resource name out=w337:refnum<visa-resource-name>, read buffer=w330:string, error out=w324:errorcluster)  [unwired: 1 out]
            n175 = VISA Flush I/O Buffer(VISA resource name=w337, mask (16)=w322, error in (no error)=w324) -> (VISA resource name out=w325:refnum<visa-resource-name>, error out=w323:errorcluster)
            n176 = VISA Flush I/O Buffer(VISA resource name=w325, mask (16)=w339, error in (no error)=w323) -> (VISA resource name out=→"ORSAY":refnum<visa-resource-name>, error out=→"VISA ERROR":errorcluster)
            n177 = Unbundle By Name(w323) -> ("status"=w345:bool)
            n178 = Not(x=w345) -> (.not. x?=→"ORSAY CONNECTED":bool)
          }
          frame #1 {
            n179 = Wait (ms)(milliseconds to wait=u32 2000 ("millisecond timer value")) -> ()  [unwired: 1 out]
          }
        }
        n180 = local write "PROCESS"(w317) -> ()
        n181 = Build Array (concatenate)(w318, w317) -> (w316:string[])
        n182 = Build Array (concatenate)(w314, w315) -> (w312:string[])
        n183 = local write "SERIAL \nRESPONSE"(w312) -> ()
      }
      frame "INITIALISE ORSAY" {
        w366 = cluster{"COARSE":sgl[unit], "FINE":sgl[unit]} {"COARSE"=0.0, "FINE"=0.0} ("CONDENSOR")
        w370 = dbl[unit][] [] ("SUPPRESSOR RAMP")
        w374 = "RESET ORSAY" ("PROCESS")
        n184 = flat-sequence {
          tunnel: [w384] -> w377
          tunnel: "DS CF12,58A4,30EE,58A4,7630,24B2,7630,DB4E,0" -> [w381]
          frame #0 {
            n185 = local read "APPEND"() -> (w382:string)
            n186 = Concatenate Strings("RE 1" ("ORSAY COMMAND"), w382) -> (w379:string)
            n187 = Concatenate Strings(w381, w382) -> (w378:string)
            n188 = local read "ORSAY"() -> (w386:refnum<visa-resource-name>)
            n189 = Build Array(w379, w378) -> (w380:string[])
            n190 = for {
              tunnel: [w399] -> w387
              tunnel: [w396] -> w384
              tunnel: w380 -> [w388] mode=indexing
              shift-right: [w397] -> w385
              shift-left: w386 -> [w398]
              n191 = VISA Write(VISA resource name=w398, write buffer=w388) -> (VISA resource name out=w392:refnum<visa-resource-name>, error out=w391:errorcluster)  [unwired: 1 in, 1 out]
              n192 = flat-sequence {
                tunnel: w392 -> [w400]
                tunnel: [w402] -> w389
                tunnel: w391 -> [w402]
                tunnel: [w400] -> w390
                frame #0 {
                  n193 = Wait (ms)(milliseconds to wait=u32 1000) -> ()  [unwired: 1 out]
                }
              }
              n194 = property class="Instr"(reference=w390, error in=w389) -> (reference out=w393:refnum<visa-resource-name>, error out=w395:errorcluster, "Serial Settings:Number of Bytes at Serial Port"=w394:u32)
              n195 = VISA Read(VISA resource name=w393, byte count=w394, error in (no error)=w395) -> (VISA resource name out=w397:refnum<visa-resource-name>, read buffer=w396:string, error out=w399:errorcluster)  [unwired: 1 out]
            }
            n196 = local write "ORSAY"(w385) -> ()
            n197 = local write "VISA ERROR"(w387) -> ()
          }
          frame #1 {
            n198 = Wait (ms)(milliseconds to wait=u32 200) -> ()  [unwired: 1 out]
          }
        }
        n199 = Build Array (concatenate)(w375, w374) -> (w373:string[])
        n200 = local write "PROCESS"(w374) -> ()
        n201 = Build Array (concatenate)(w376, w377) -> (w371:string[])
        n202 = local write "SERIAL \nRESPONSE"(w371) -> ()
        n203 = local write "CONDENSOR"(w366) -> ()
        n204 = local write "OBJECTIVE"(w366) -> ()
        n205 = property on="SUPPRESSOR" class="Slide (strict)"("DisabledEnum"=T17."Disabled and Grayed Out" ("Disabled")) -> ()  [unwired: 2 in, 2 out]
        n206 = property on="ION CURRENT" class="Slide (strict)"("DisabledEnum"=T17."Disabled and Grayed Out" ("Disabled")) -> ()  [unwired: 2 in, 2 out]
        n207 = property on="EXTRACTOR" class="Slide (strict)"("DisabledEnum"=T17."Disabled and Grayed Out" ("Disabled")) -> ()  [unwired: 2 in, 2 out]
        n208 = property on="SUPPRESSOR" class="Slide (strict)" props=["DisabledEnum"]() -> ()  [unwired: 2 in, 3 out]
        n209 = local write "ION GUN SETTINGS"(T18 {"BEAM ENERGY"=0.0, "EXTRACTOR"=0.0, "SUPPRESSOR"=0.0, "ION CURRENT"=0.0} ("ION GUN SETTINGS")) -> ()
        n210 = local write "EXTRACTOR RAMP"(w370) -> ()
        n211 = local write "BEAM RAMP"(w370) -> ()
        n212 = local write "SUPPRESSOR RAMP"(w370) -> ()
        "SUPPRESSOR RAMP" <- w370
        "EXTRACTOR RAMP" <- w370
        "BEAM RAMP" <- w370
      }
      frame "TEST COMMANDS" {
        n213 = flat-sequence {
          frame #0 {
            n214 = local read "APPEND"() -> (w417:string)
            n215 = Concatenate Strings("TEST COMMAND", w417) -> (w408:string)
            n216 = local read "VISA ERROR"() -> (w418:errorcluster)
            n217 = local read "ORSAY"() -> (w419:refnum<visa-resource-name>)
            n218 = VISA Write(VISA resource name=w419, write buffer=w408, error in (no error)=w418) -> (VISA resource name out=w412:refnum<visa-resource-name>, error out=w411:errorcluster)  [unwired: 1 out]
            n219 = flat-sequence {
              tunnel: w412 -> [w422]
              tunnel: [w424] -> w409
              tunnel: w411 -> [w424]
              tunnel: [w422] -> w410
              frame #0 {
                n220 = Wait (ms)(milliseconds to wait=u32 1000) -> ()  [unwired: 1 out]
              }
            }
            n221 = property class="Instr"(reference=w410, error in=w409) -> (reference out=w413:refnum<visa-resource-name>, error out=w415:errorcluster, "Serial Settings:Number of Bytes at Serial Port"=w414:u32)
            n222 = VISA Read(VISA resource name=w413, byte count=w414, error in (no error)=w415) -> (VISA resource name out=w421:refnum<visa-resource-name>, read buffer=→"TEST OUTPUT":string, error out=w420:errorcluster)  [unwired: 1 out]
            n223 = local write "ORSAY"(w421) -> ()
            n224 = local write "VISA ERROR"(w420) -> ()
          }
          frame #1 {
            n225 = local write "TEST COMMAND"(FALSE ("TEST COMMAND")) -> ()
          }
        }
      }
      frame "VACUUM " {
        w434 = "VACUUM CHECK"
        w467 = i16 2
        w466 = i16 2
        # "Bypass"
        # "Where is the column vac ?\nMust be before manual GV"
        # "Need a measure of vac in the target chamber & valve ??"
        n226 = local read "VISA ERROR"() -> (w484:errorcluster)
        n227 = local read "APPEND"() -> (w430:string)
        n228 = local read "ORSAY"() -> (w485:refnum<visa-resource-name>)
        n229 = Concatenate Strings("GV F", w430) -> (w446:string)
        n230 = Concatenate Strings("GV D", w430) -> (w444:string)
        n231 = VISA Write(VISA resource name=w485, write buffer=w446, error in (no error)=w484) -> (VISA resource name out=w442:refnum<visa-resource-name>, error out=w440:errorcluster)  [unwired: 1 out]
        n232 = flat-sequence {
          tunnel: [w497] -> w436
          tunnel: w439 -> [w497]
          tunnel: [w496] -> w437
          tunnel: w438 -> [w496]
          frame #0 {
            n233 = Wait (ms)(milliseconds to wait=u32 200) -> ()  [unwired: 1 out]
          }
        }
        n234 = flat-sequence {
          tunnel: [w500] -> w443
          tunnel: w442 -> [w500]
          tunnel: [w499] -> w441
          tunnel: w440 -> [w499]
          frame #0 {
            n235 = Wait (ms)(milliseconds to wait=u32 200) -> ()  [unwired: 1 out]
          }
        }
        n236 = property class="Instr"(reference=w443, error in=w441) -> (reference out=w453:refnum<visa-resource-name>, error out=w452:errorcluster, "Serial Settings:Number of Bytes at Serial Port"=w451:u32)
        n237 = property class="Instr"(reference=w436, error in=w437) -> (reference out=w450:refnum<visa-resource-name>, error out=w448:errorcluster, "Serial Settings:Number of Bytes at Serial Port"=w449:u32)
        n238 = VISA Read(VISA resource name=w453, byte count=w451, error in (no error)=w452) -> (VISA resource name out=w465:refnum<visa-resource-name>, read buffer=w455:string)  [unwired: 2 out]
        n239 = VISA Write(VISA resource name=w465, write buffer=w444) -> (VISA resource name out=w439:refnum<visa-resource-name>, error out=w438:errorcluster)  [unwired: 1 in, 1 out]
        n240 = VISA Read(VISA resource name=w450, byte count=w449, error in (no error)=w448) -> (VISA resource name out=w464:refnum<visa-resource-name>, read buffer=w454:string, error out=w463:errorcluster)  [unwired: 1 out]
        n241 = local write "ORSAY"(w464) -> ()
        n242 = local write "VISA ERROR"(w463) -> ()
        n243 = Concatenate Strings(w455, w454) -> (w435:string)
        n244 = Match Pattern(string=w455, regular expression=",") -> (before substring=w473:string)  [unwired: 1 in, 3 out]
        n245 = Match Pattern(string=w454, regular expression=",") -> (before substring=w475:string)  [unwired: 1 in, 3 out]
        n246 = property on="COLUMN VACUUM" class="Knob (strict)"("Scale.RampVis"=TRUE ("Scale.Ramp Visible")) -> ()  [unwired: 2 in, 2 out]
        n247 = local write "PROCESS"(w434) -> ()
        n248 = Hexadecimal String To Number(string=w473, offset=w466, default (0uL)=w466) -> (number=w477:i16)  [unwired: 1 out]
        n249 = Hexadecimal String To Number(string=w475, offset=w467, default (0uL)=w467) -> (number=w474:i16)  [unwired: 1 out]
        n250 = Absolute Value(x=w474) -> (abs(x)=w479:i16)
        n251 = Less?(x=w477, y=320) -> (x < y?=w480:bool)
        n252 = Build Array (concatenate)(w433, w434) -> (w432:string[])
        n253 = Equal To 0?(x=w477) -> (x = 0?=w476:bool)
        n254 = Equal To 0?(x=w479) -> (x = 0?=w478:bool)
        n255 = Build Array (concatenate)(w431, w435) -> (w426:string[])
        n256 = local write "PROCESSES"(w432) -> ()
        n257 = Select(t=i16 1, s=w476, f=w477) -> (s? t:f=w481:i16)
        n258 = Select(t=i16 1, s=w478, f=w479) -> (s? t:f=w482:i16)
        n259 = case shown="True" w480 {
          tunnel: w481 -> [w502 _]
          tunnel: w482 -> [_ w505]
          tunnel: [w501 w506] -> w483
          frame False {
            n260 = To Single Precision Float(number=w502) -> (single precision float=w501:sgl)
          }
          frame True {
            n261 = To Single Precision Float(number=w505) -> (single precision float=w503:sgl)
            n262 = Divide(x=w503, y=sgl 20.0) -> (x/y=w506:sgl)
          }
        }
        n263 = formula code="k=log(lp/3276700)-2.7;\np=10** k;"("lp"=w483) -> ("p"=w461:dbl)  [unwired: 1 out]
        n264 = node(w461) -> (w456:dbl[unit])
        "COLUMN VACUUM" <- w456
        n265 = Bundle(w456, "COLUMN THRESHOLD"="COLUMN THRESHOLD") -> (→"COLUMN VACUUM":cluster{dbl[unit], "COLUMN THRESHOLD":dbl[unit]})  [unwired: 1 in]
        n266 = Bundle(w456, "CHAMBER THRESHOLD"="CHAMBER THRESHOLD") -> (→"CHAMBER VACUUM":T24)  [unwired: 1 in]
        n267 = Less?(x=w456, y="COLUMN THRESHOLD") -> (x < y?=w429:bool)
        "VACUUM STATE" <- w429
        n268 = case shown="False" w429 {
          tunnel: w428 -> [w490 w494]
          tunnel: [w489 w494] -> w427
          frame False {
            w488 = T15[] [enum."TOGGLE GATE VALVE", enum."RESET TYPE II"] items=["LOOP", "OPEN SERIAL CONN TO ORSAY", "INITIALISE ORSAY", "READ SETTINGS", "SAVE SETTINGS", "OBJECTIVE LENS", "CONDENSOR LENS", "BLANKING TOGGLE", "TURN ON HEATER", "TURN OFF WOBBLER", "MEASURE HEATER OUTPUT", "TOGGLE GATE VALVE", "SCANNING CONTROLS", "TURN ON BEAM HV", "ENERGY RAMP CYCLE", "TURN ON SUPPRESSOR", "TURN ON EXTRACTOR", "SET ENERGY RANGE", "MEASURE HV SUPPLY VOLTAGES", "SHUTDOWN ION SOURCE", "RESET TYPE II", "PROBE CURRENT FC#1", "PROBE CURRENT FC#2", "VACUUM ", "CHECK 150V", "INITIALISE PI MOTORS", "SET STIGMATOR", "SET WOBBLER FOR OBJECT", "SET OBJ & AP STAGE VELOCITIES", "READ APERTURE POSITIONS", "HOME OBJ & AP STAGES", "DEFINE NEW OBJ", "MOVE OBJ STAGES", "DEFINE NEW APERTURE", "MOVE APERTURE STAGES", "STOP SYSTEM", "TEST COMMANDS"]
            n269 = local write "GATE VALVE"(FALSE ("GATE VALVE")) -> ()
            n270 = for {
              shift-right: [w492] -> w489
              shift-left: w490 -> [w493]
              tunnel: w488 -> [w491] mode=indexing
              n271 = Enqueue Element(queue=w493, element=w491) -> (queue out=w492:refnum<queue>)  [unwired: 2 in, 2 out]
            }
            n272 = One Button Dialog(message="FIB Low Vacuum !") -> ()  [unwired: 1 in, 1 out]
          }
          frame True {
          }
        }
        n273 = local write "SERIAL \nRESPONSE"(w426) -> ()
      }
      frame "RESET TYPE II" {
        n274 = local read "APPEND"() -> (w508:string)
        n275 = local read "VISA ERROR"() -> (w511:errorcluster)
        n276 = local read "ORSAY"() -> (w512:refnum<visa-resource-name>)
        n277 = Concatenate Strings("RE 2", w508) -> (w518:string)
        n278 = VISA Write(VISA resource name=w512, write buffer=w518, error in (no error)=w511) -> (VISA resource name out=w522:refnum<visa-resource-name>, error out=w519:errorcluster)  [unwired: 1 out]
        n279 = flat-sequence {
          tunnel: [w530] -> w521
          tunnel: w522 -> [w530]
          tunnel: [w529] -> w520
          tunnel: w519 -> [w529]
          frame #0 {
            n280 = Wait (ms)(milliseconds to wait=u32 200) -> ()  [unwired: 1 out]
          }
        }
        n281 = Build Array (concatenate)(w517, "RESET TYPE II") -> (w515:string[])
        n282 = property class="Instr"(reference=w521, error in=w520) -> (reference out=w525:refnum<visa-resource-name>, error out=w524:errorcluster, "Serial Settings:Number of Bytes at Serial Port"=w523:u32)
        n283 = local write "PROCESSES"(w515) -> ()
        n284 = VISA Read(VISA resource name=w525, byte count=w523, error in (no error)=w524) -> (VISA resource name out=w510:refnum<visa-resource-name>, read buffer=w514:string, error out=w509:errorcluster)  [unwired: 1 out]
        n285 = Build Array (concatenate)(w513, w514) -> (w507:string[])
        n286 = local write "SERIAL \nRESPONSE"(w507) -> ()
        n287 = local write "ORSAY"(w510) -> ()
        n288 = local write "VISA ERROR"(w509) -> ()
      }
      frame "CHECK 150V" {
        # "Should be true for 150V OK"
        # "NOT COMPLETE!!"
        n289 = local read "APPEND"() -> (w533:string)
        n290 = local read "ORSAY"() -> (w557:refnum<visa-resource-name>)
        n291 = Concatenate Strings("GV 15", w533) -> (w546:string)
        n292 = local read "VISA ERROR"() -> (w556:errorcluster)
        n293 = VISA Write(VISA resource name=w557, write buffer=w546, error in (no error)=w556) -> (VISA resource name out=w544:refnum<visa-resource-name>, error out=w542:errorcluster)  [unwired: 1 out]
        n294 = flat-sequence {
          tunnel: [w567] -> w545
          tunnel: w544 -> [w567]
          tunnel: [w566] -> w543
          tunnel: w542 -> [w566]
          frame #0 {
            n295 = Wait (ms)(milliseconds to wait=u32 50) -> ()  [unwired: 1 out]
          }
        }
        n296 = property class="Instr"(reference=w545, error in=w543) -> (reference out=w552:refnum<visa-resource-name>, error out=w550:errorcluster, "Serial Settings:Number of Bytes at Serial Port"=w551:u32)
        n297 = Build Array (concatenate)(w536, "150V CHECK") -> (w535:string[])
        n298 = VISA Read(VISA resource name=w552, byte count=w551, error in (no error)=w550) -> (VISA resource name out=w555:refnum<visa-resource-name>, read buffer=w538:string, error out=w554:errorcluster)  [unwired: 1 out]
        n299 = local write "VISA ERROR"(w554) -> ()
        n300 = local write "PROCESSES"(w535) -> ()
        n301 = local write "ORSAY"(w555) -> ()
        n302 = call <vilib>:"Trim Whitespace.vi"("string"=w538) -> ("trimmed string"=w541:string)  [unwired: 1 in]
        n303 = Match Pattern(string=w541, regular expression=",") -> (after substring=w540:string)  [unwired: 1 in, 3 out]
        n304 = Build Array (concatenate)(w534, w538) -> (w531:string[])
        n305 = Hexadecimal String To Number(string=w540, default (0uL)=i16 0 ("constante")) -> (number=w549:i16)  [unwired: 1 in, 1 out]
        n306 = local write "SERIAL \nRESPONSE"(w531) -> ()
        n307 = Compound Arithmetic op=AND(w549, 64 ("constante")) -> (w562:i32)
        n308 = Compound Arithmetic op=AND(w549, 16 ("constante")) -> (w563:i32)
        n309 = Not Equal To 0?(x=w562) -> (x != 0?=w560:bool)
        n310 = Not Equal To 0?(x=w563) -> (x != 0?=w548:bool)
        n311 = Or(x=w560, y=w548) -> (x .or. y?=w539:bool)
        "150V GOOD" <- w539
        n312 = case shown="True" w539 {
          tunnel: ["150V INTERLOCKED!" ""] -> w553
          frame False {
          }
          frame True {
          }
        }
        n313 = local write "WARNING"(w553) -> ()
      }
      frame "PROBE CURRENT FC#1" {
        w579 = "MEASURE PROBE CURRENT #1"
        w612 = i16 2
        w606 = i16 2
        n314 = local read "VISA ERROR"() -> (w593:errorcluster)
        n315 = local read "ORSAY"() -> (w600:refnum<visa-resource-name>)
        n316 = local read "APPEND"() -> (w575:string)
        n317 = Concatenate Strings("GV 9", w575) -> (w578:string)
        n318 = VISA Write(VISA resource name=w600, write buffer=w578, error in (no error)=w593) -> (VISA resource name out=w591:refnum<visa-resource-name>, error out=w588:errorcluster)  [unwired: 1 out]
        n319 = flat-sequence {
          tunnel: [w630] -> w590
          tunnel: w591 -> [w630]
          tunnel: [w629] -> w589
          tunnel: w588 -> [w629]
          frame #0 {
            n320 = Wait (ms)(milliseconds to wait=u32 200) -> ()  [unwired: 1 out]
          }
        }
        n321 = property class="Instr"(reference=w590, error in=w589) -> (reference out=w605:refnum<visa-resource-name>, error out=w597:errorcluster, "Serial Settings:Number of Bytes at Serial Port"=w604:u32)
        n322 = local read "APPEND"() -> (w573:string)
        n323 = VISA Read(VISA resource name=w605, byte count=w604, error in (no error)=w597) -> (VISA resource name out=w599:refnum<visa-resource-name>, read buffer=w603:string, error out=w598:errorcluster)  [unwired: 1 out]
        n324 = Match Pattern(string=w603, regular expression=",") -> (before substring=w615:string)  [unwired: 1 in, 3 out]
        n325 = Concatenate Strings("GV 8", w573) -> (w576:string)
        n326 = Hexadecimal String To Number(string=w615, offset=w606, default (0uL)=w606) -> (number=w622:i16)  [unwired: 1 out]
        n327 = VISA Write(VISA resource name=w599, write buffer=w576, error in (no error)=w598) -> (VISA resource name out=w587:refnum<visa-resource-name>, error out=w585:errorcluster)  [unwired: 1 out]
        n328 = Divide(x=w622, y=i16 32767) -> (x/y=w616:dbl)
        n329 = Build Array (concatenate)(w580, w579) -> (w581:string[])
        n330 = Less?(x=w622, y=i16 1600) -> (x < y?=w620:bool)
        "gamme" <- w620
        n331 = Multiply(x=w616, y=sgl 21.28) -> (x*y=w617:dbl)
        n332 = local write "PROCESS"(w579) -> ()
        n333 = flat-sequence {
          tunnel: [w627] -> w586
          tunnel: w587 -> [w627]
          tunnel: [w626] -> w584
          tunnel: w585 -> [w626]
          frame #0 {
            n334 = Wait (ms)(milliseconds to wait=u32 100) -> ()  [unwired: 1 out]
          }
        }
        n335 = property class="Instr"(reference=w586, error in=w584) -> (reference out=w602:refnum<visa-resource-name>, error out=w596:errorcluster, "Serial Settings:Number of Bytes at Serial Port"=w601:u32)
        n336 = VISA Read(VISA resource name=w602, byte count=w601, error in (no error)=w596) -> (VISA resource name out=w595:refnum<visa-resource-name>, read buffer=w583:string, error out=w594:errorcluster)  [unwired: 1 out]
        n337 = Match Pattern(string=w583, regular expression=",") -> (before substring=w621:string)  [unwired: 1 in, 3 out]
        n338 = Hexadecimal String To Number(string=w621, offset=w612, default (0uL)=w612) -> (number=w624:i16)  [unwired: 1 out]
        n339 = Negate(x=w624) -> (-x=w623:i16)
        n340 = Divide(x=w623, y=i16 32767) -> (x/y=w618:dbl)
        n341 = Multiply(x=w618, y=sgl 1060.0) -> (x*y=w619:dbl)
        n342 = case shown="True" w620 {
          tunnel: w617 -> [w631 _]
          tunnel: w619 -> [_ w632]
          tunnel: [w631 w632] -> w592
          frame False {
            (unwired) "Probe current (nA)" ("Définir l'attribut")
          }
          frame True {
            (unwired) "Probe current (pA)" ("Définir l'attribut")
          }
        }
        n343 = node(w592) -> (w571:dbl[unit])
        n344 = Build Array (concatenate)(w582, w583) -> (w570:string[])
        n345 = local write "SERIAL \nRESPONSE"(w570) -> ()
        n346 = local write "BEAM CURRENT (FC1)"(w571) -> ()
        n347 = local write "ORSAY"(w595) -> ()
        n348 = local write "VISA ERROR"(w594) -> ()
      }
      frame "PROBE CURRENT FC#2" {
      }
      frame "CONDENSOR LENS" {
        w643 = u16 3 items=["BEAM ENERGY", "EXTRACTOR", "SUPPRESSOR", "CONDENSOR", "OBJECTIVE"] ("HV SUPPLY")
        w648 = "CONDENSOR LENS"
        n349 = local read "CONDENSOR"() -> (w651:cluster{"COARSE":sgl[unit], "FINE":sgl[unit]})
        n350 = Unbundle By Name(w651) -> ("COARSE"=w642:sgl[unit], "FINE"=w641:sgl[unit])
        n351 = local read "VISA ERROR"() -> (w645:errorcluster)
        n352 = local read "ORSAY"() -> (w646:refnum<visa-resource-name>)
        n353 = Add(x=w642, y=w641) -> (x+y=w636:sgl[unit])
        n354 = local read "TIMER"() -> (w638:u32)
        n355 = local write "PROCESS"(w648) -> ()
        n356 = local read "APPEND"() -> (w644:string)
        n357 = call "SET HV SUPPLY MEASURE IV.vi"("ORSAY"=w646, "SETTLE"=w638, "HV SUPPLY"=w643, "VOLTAGE"=w636, "ORSAY ERROR"=w645, "APPEND"=w644) -> ("ORSAY 2"=w640:refnum<visa-resource-name>, "ORSAY ERROR"=w639:errorcluster)  [unwired: 8 in]
        n358 = Build Array (concatenate)(w649, w648) -> (w650:string[])
        n359 = local write "ORSAY"(w640) -> ()
        n360 = local write "VISA ERROR"(w639) -> ()
      }
      frame "SHUTDOWN ION SOURCE" {
        w655 = FALSE ("TURN ON FILAMENT")
        n361 = local write "FILAMENT HEATING"(dbl[unit] 0.0 ("FILAMENT HEATING")) -> ()
        n362 = local write "ION GUN"(w655) -> ()
        n363 = local write "FILAMENT"(w655) -> ()
        n364 = local write "ION GUN SETTINGS"(T18 {"BEAM ENERGY"=0.0, "EXTRACTOR"=0.0, "SUPPRESSOR"=0.0, "ION CURRENT"=0.0} ("ION GUN SETTINGS")) -> ()
      }
      frame "TURN ON HEATER" {
        w663 = "TURN ON HEATER"
        n365 = local read "FILAMENT"() -> (w658:bool)
        n366 = case shown="True" w658 {
          tunnel: ["SH 0,0" w687] -> w661
          frame False {
          }
          frame True {
            n367 = local read "FILAMENT HEATING"() -> (w682:dbl[unit])
            n368 = node(w682) -> (w680:dbl)
            n369 = call "conversion data to bits.vi"("Data input"=w680, "15 /16b"=TRUE, "Max supply"=sgl 5.0) -> ("15 bits output"=w684:u16)  [unwired: 1 out]
            n370 = Number To Hexadecimal String(2:w684) -> (0:w685:string)  [unwired: 1 in]
            n371 = Concatenate Strings("SH ", w685, ",1" ("string")) -> (w687:string)
          }
        }
        n372 = local read "VISA ERROR"() -> (w668:errorcluster)
        n373 = local read "ORSAY"() -> (w669:refnum<visa-resource-name>)
        n374 = VISA Write(VISA resource name=w669, write buffer=w661, error in (no error)=w668) -> (VISA resource name out=w675:refnum<visa-resource-name>, error out=w672:errorcluster)  [unwired: 1 out]
        n375 = flat-sequence {
          tunnel: [w691] -> w674
          tunnel: w675 -> [w691]
          tunnel: [w690] -> w673
          tunnel: w672 -> [w690]
          frame #0 {
            n376 = Wait (ms)(milliseconds to wait=u32 200) -> ()  [unwired: 1 out]
          }
        }
        n377 = property class="Instr"(reference=w674, error in=w673) -> (reference out=w678:refnum<visa-resource-name>, error out=w677:errorcluster, "Serial Settings:Number of Bytes at Serial Port"=w676:u32)
        n378 = VISA Read(VISA resource name=w678, byte count=w676, error in (no error)=w677) -> (VISA resource name out=w671:refnum<visa-resource-name>, read buffer=w667:string, error out=w670:errorcluster)  [unwired: 1 out]
        n379 = local write "ORSAY"(w671) -> ()
        n380 = local write "VISA ERROR"(w670) -> ()
        n381 = local write "PROCESS"(w663) -> ()
        n382 = Build Array (concatenate)(w665, w663) -> (w662:string[])
        n383 = local write "PROCESSES"(w662) -> ()
        n384 = property on="FILAMENT HEATING" class="Slide (strict)"("DisabledEnum"=T17."Enabled" ("Disabled")) -> ()  [unwired: 2 in, 2 out]
        n385 = Build Array (concatenate)(w664, w667) -> (w659:string[])
        n386 = local write "SERIAL \nRESPONSE"(w659) -> ()
      }
      frame "MEASURE HEATER OUTPUT" {
        w700 = T25 0 items=["both", "start of string", "end of string"] ("location (both)")
        w709 = T25 0 items=["both", "start of string", "end of string"] ("location (both)")
        # "SH, 0, 3.8e-4,0,0,0.71e-3"
        n387 = local read "VISA ERROR"() -> (w725:errorcluster)
        n388 = local read "APPEND"() -> (w728:string)
        n389 = local read "ORSAY"() -> (w726:refnum<visa-resource-name>)
        n390 = Concatenate Strings("GV 18" ("string"), w728) -> (w741:string)
        n391 = VISA Write(VISA resource name=w726, write buffer=w741, error in (no error)=w725) -> (VISA resource name out=w745:refnum<visa-resource-name>, error out=w744:errorcluster)  [unwired: 1 out]
        n392 = flat-sequence {
          tunnel: [w756] -> w743
          tunnel: w745 -> [w756]
          tunnel: [w755] -> w742
          tunnel: w744 -> [w755]
          frame #0 {
            n393 = Wait (ms)(milliseconds to wait=u32 100) -> ()  [unwired: 1 out]
          }
        }
        n394 = property class="Instr"(reference=w743, error in=w742) -> (reference out=w748:refnum<visa-resource-name>, error out=w747:errorcluster, "Serial Settings:Number of Bytes at Serial Port"=w746:u32)
        n395 = VISA Read(VISA resource name=w748, byte count=w746, error in (no error)=w747) -> (VISA resource name out=w730:refnum<visa-resource-name>, read buffer=w702:string, error out=w729:errorcluster)  [unwired: 1 out]
        n396 = call <vilib>:"Trim Whitespace.vi"("string"=w702, "location (both)"=w709) -> ("trimmed string"=w708:string)
        n397 = Match Pattern(string=w708, regular expression="FIB>") -> (before substring=w706:string)  [unwired: 1 in, 3 out]
        n398 = Match Pattern(string=w706, regular expression=",") -> (before substring=w703:string)  [unwired: 1 in, 3 out]
        n399 = Hexadecimal String To Number(string=w703, default (0uL)=u16 0 ("default (0 U32)")) -> (number=w701:u16)  [unwired: 1 in, 1 out]
        n400 = To Double Precision Float(number=w701) -> (double precision float=w713:dbl)
        n401 = Multiply(x=w713, y="IGAIN") -> (x*y=w721:dbl)
        n402 = Add(x=w721, y="IOFFSET") -> (x+y=→"HEATING CURRENT":dbl)
        n403 = local read "APPEND"() -> (w727:string)
        n404 = Concatenate Strings("GV 19" ("string"), w727) -> (w733:string)
        n405 = VISA Write(VISA resource name=w730, write buffer=w733, error in (no error)=w729) -> (VISA resource name out=w737:refnum<visa-resource-name>, error out=w736:errorcluster)  [unwired: 1 out]
        n406 = flat-sequence {
          tunnel: [w753] -> w735
          tunnel: w737 -> [w753]
          tunnel: [w752] -> w734
          tunnel: w736 -> [w752]
          frame #0 {
            n407 = Wait (ms)(milliseconds to wait=u32 100) -> ()  [unwired: 1 out]
          }
        }
        n408 = Build Array (concatenate)(w712, "MEASURE HEATER OUTPUT") -> (w711:string[])
        n409 = property class="Instr"(reference=w735, error in=w734) -> (reference out=w740:refnum<visa-resource-name>, error out=w739:errorcluster, "Serial Settings:Number of Bytes at Serial Port"=w738:u32)
        n410 = VISA Read(VISA resource name=w740, byte count=w738, error in (no error)=w739) -> (VISA resource name out=w724:refnum<visa-resource-name>, read buffer=w695:string, error out=w723:errorcluster)  [unwired: 1 out]
        n411 = call <vilib>:"Trim Whitespace.vi"("string"=w695, "location (both)"=w700) -> ("trimmed string"=w699:string)
        n412 = Match Pattern(string=w699, regular expression="FIB>") -> (before substring=w697:string)  [unwired: 1 in, 3 out]
        n413 = local write "ORSAY"(w724) -> ()
        n414 = local write "VISA ERROR"(w723) -> ()
        n415 = Match Pattern(string=w697, regular expression=",") -> (before substring=w693:string)  [unwired: 1 in, 3 out]
        n416 = Hexadecimal String To Number(string=w693, default (0uL)=u16 0 ("default (0 U32)")) -> (number=w692:u16)  [unwired: 1 in, 1 out]
        n417 = To Double Precision Float(number=w692) -> (double precision float=w714:dbl)
        n418 = Multiply(x="VGAIN", y=w714) -> (x*y=w716:dbl)
        n419 = Add(x="VOFFSET", y=w716) -> (x+y=→"HEATING VOLTAGE":dbl)
      }
      frame "TOGGLE GATE VALVE" {
        n420 = local read "GATE VALVE"() -> (w765:bool)
        n421 = case shown="True" w765 {
          tunnel: ["1" "0"] -> w764
          tunnel: ["OPENING GATE VALVE" "CLOSING GATE VALVE"] -> w763
          frame False {
          }
          frame True {
          }
        }
        n422 = local read "VISA ERROR"() -> (w775:errorcluster)
        n423 = local read "ORSAY"() -> (w774:refnum<visa-resource-name>)
        n424 = local read "APPEND"() -> (w759:string)
        n425 = Concatenate Strings("VC ", w764, w759) -> (w776:string)
        n426 = VISA Write(VISA resource name=w774, write buffer=w776, error in (no error)=w775) -> (VISA resource name out=w770:refnum<visa-resource-name>, error out=w773:errorcluster)  [unwired: 1 out]
        n427 = flat-sequence {
          tunnel: [w786] -> w771
          tunnel: w770 -> [w786]
          tunnel: [w785] -> w772
          tunnel: w773 -> [w785]
          frame #0 {
            n428 = Wait (ms)(milliseconds to wait=u32 200) -> ()  [unwired: 1 out]
          }
        }
        n429 = Build Array (concatenate)(w762, w763) -> (w761:string[])
        n430 = local write "PROCESSES"(w761) -> ()
        n431 = property class="Instr"(reference=w771, error in=w772) -> (reference out=w767:refnum<visa-resource-name>, error out=w768:errorcluster, "Serial Settings:Number of Bytes at Serial Port"=w769:u32)
        n432 = VISA Read(VISA resource name=w767, byte count=w769, error in (no error)=w768) -> (VISA resource name out=w777:refnum<visa-resource-name>, read buffer=w779:string, error out=w778:errorcluster)  [unwired: 1 out]
        n433 = local write "ORSAY"(w777) -> ()
        n434 = local write "VISA ERROR"(w778) -> ()
        n435 = Build Array (concatenate)(w760, w779) -> (w757:string[])
        n436 = local write "SERIAL \nRESPONSE"(w757) -> ()
      }
      frame "OBJECTIVE LENS" {
        w791 = "OBJECTIVE LENS"
        n437 = local read "OBJECTIVE"() -> (w814:cluster{"COARSE":sgl[unit], "FINE":sgl[unit]})
        n438 = Unbundle By Name(w814) -> ("COARSE"=w809:sgl[unit], "FINE"=w808:sgl[unit])
        n439 = node(w809) -> (w806:sgl)
        n440 = node(w808) -> (w807:sgl)
        n441 = Add(x=w806, y=w807) -> (x+y=w805:sgl)
        n442 = local read "VISA ERROR"() -> (w801:errorcluster)
        n443 = call "conversion data to bits.vi"("Data input"=w805, "Max supply"=sgl 20000.0) -> ("15 bits output"=w811:u16)  [unwired: 1 in, 1 out]
        n444 = local write "PROCESS"(w791) -> ()
        n445 = local read "ORSAY"() -> (w816:refnum<visa-resource-name>)
        n446 = Number To Hexadecimal String(2:w811) -> (0:w810:string)  [unwired: 1 in]
        n447 = local read "APPEND"() -> (w789:string)
        n448 = Concatenate Strings("L2 ", w810, w789) -> (w790:string)
        n449 = Build Array (concatenate)(w793, w791) -> (w792:string[])
        n450 = VISA Write(VISA resource name=w816, write buffer=w790, error in (no error)=w801) -> (VISA resource name out=w800:refnum<visa-resource-name>, error out=w799:errorcluster)  [unwired: 1 out]
        n451 = flat-sequence {
          tunnel: [w819] -> w798
          tunnel: w800 -> [w819]
          tunnel: [w818] -> w797
          tunnel: w799 -> [w818]
          frame #0 {
            n452 = Wait (ms)(milliseconds to wait=u32 200) -> ()  [unwired: 1 out]
          }
        }
        n453 = local write "PROCESSES"(w792) -> ()
        n454 = property class="Instr"(reference=w798, error in=w797) -> (reference out=w804:refnum<visa-resource-name>, error out=w803:errorcluster, "Serial Settings:Number of Bytes at Serial Port"=w802:u32)
        n455 = VISA Read(VISA resource name=w804, byte count=w802, error in (no error)=w803) -> (VISA resource name out=w815:refnum<visa-resource-name>, read buffer=w795:string, error out=w796:errorcluster)  [unwired: 1 out]
        n456 = local write "ORSAY"(w815) -> ()
        n457 = local write "VISA ERROR"(w796) -> ()
        n458 = Build Array (concatenate)(w794, w795) -> (w787:string[])
        n459 = local write "SERIAL \nRESPONSE"(w787) -> ()
      }
      frame "SET ENERGY RANGE" {
        # "HIGH energy range (MAX 30kV)"
        # "LOW energy range (MAX 10kV)"
        n460 = local read "HIGH ENERGY"() -> (w821:bool)
        n461 = local read "VISA ERROR"() -> (w838:errorcluster)
        n462 = local read "ORSAY"() -> (w839:refnum<visa-resource-name>)
        n463 = Select(t="RE 3", s=w821, f="RE 4") -> (s? t:f=w832:string)
        n464 = VISA Write(VISA resource name=w839, write buffer=w832, error in (no error)=w838) -> (VISA resource name out=w828:refnum<visa-resource-name>, error out=w827:errorcluster)  [unwired: 1 out]
        n465 = flat-sequence {
          tunnel: [w842] -> w825
          tunnel: w828 -> [w842]
          tunnel: [w841] -> w826
          tunnel: w827 -> [w841]
          frame #0 {
            n466 = Wait (ms)(milliseconds to wait=u32 200) -> ()  [unwired: 1 out]
          }
        }
        n467 = property class="Instr"(reference=w825, error in=w826) -> (reference out=w831:refnum<visa-resource-name>, error out=w830:errorcluster, "Serial Settings:Number of Bytes at Serial Port"=w829:u32)
        n468 = VISA Read(VISA resource name=w831, byte count=w829, error in (no error)=w830) -> (VISA resource name out=w837:refnum<visa-resource-name>, read buffer=w824:string, error out=w836:errorcluster)  [unwired: 1 out]
        n469 = Build Array (concatenate)(w835, w824) -> (w820:string[])
        n470 = local write "SERIAL \nRESPONSE"(w820) -> ()
        n471 = local write "VISA ERROR"(w836) -> ()
        n472 = local write "ORSAY"(w837) -> ()
      }
      frame "TURN ON BEAM HV" {
        w843 = "RAMPING UP/DOWN ION GUN PARAMETERS" ("PROCESS")
        n473 = flat-sequence {
          tunnel: [w852] -> w846
          tunnel: [w851] -> w844
          tunnel: w850 -> [w858]
          tunnel: [w857] -> w849
          tunnel: w846 -> [w855]
          tunnel: w844 -> [w854]
          frame #0 {
            n474 = local read "HIGH VOLTAGE SUPPLIES"() -> (w851:cluster{dbl[unit], dbl[unit], dbl[unit]})
            n475 = local read "ION GUN SETTINGS"() -> (w852:T5)
          }
          frame #1 {
            # "New settings"
            n476 = Unbundle By Name(w855) -> ("BEAM ENERGY"=w856:sgl[unit])
            n477 = Unbundle(w854) -> (w853:dbl[unit])  [unwired: 2 out]
            n478 = stacked-sequence {
              tunnel: w856 -> [w869 _ _]
              tunnel: w858 -> [_ w889 _]
              tunnel: w853 -> [w859 _ _]
              tunnel: [_ w889 _] -> w857
              frame #0 {
                n479 = Subtract(x=w869, y=w859) -> (x-y=w866:dbl[unit])
                n480 = node(w866) -> (w865:dbl)
                n481 = Greater Than 0?(x=w865) -> (x > 0?=w867:bool)
                n482 = case shown="False" w867 {
                  tunnel: [w872 w874] -> w861
                  tunnel: "dV ENERGY" -> [w873 w874]
                  frame False {
                    n483 = Negate(x=w873) -> (-x=w872:dbl[unit])
                  }
                  frame True {
                  }
                }
                n484 = Absolute Value(x=w866) -> (abs(x)=w868:dbl[unit])
                n485 = Divide(x=w868, y=w861) -> (x/y=w871:dbl)
                n486 = Absolute Value(x=w871) -> (abs(x)=w860:dbl)
                n487 = To Long Integer(number=w860) -> (32bit integer=w870:i32)
                n488 = for {
                  N: w870 -> [_]
                  tunnel: w861 -> [w878]
                  tunnel: [w875] -> w862 mode=indexing
                  tunnel: w859 -> [w876]
                  i -> [w880]
                  n489 = Increment(x=w880) -> (x+1=w879:i32)
                  n490 = Multiply(x=w878, y=w879) -> (x*y=w877:dbl[unit])
                  n491 = Add(x=w876, y=w877) -> (x+y=w875:dbl[unit])
                }
                "BEAM RAMP" <- w862
                n492 = local write "BEAM RAMP"(w862) -> ()
                n493 = Array Size(array=w862) -> (size(s)=→"size(s)":i32)
              }
              frame #1 {
                n494 = local read "BEAM RAMP"() -> (w882:dbl[unit][])
                n495 = Array Size(array=w882) -> (size(s)=w881:i32)
                n496 = local read "VISA ERROR"() -> (w887:errorcluster)
                n497 = local read "ORSAY"() -> (w888:refnum<visa-resource-name>)
                n498 = local read "TIMER"() -> (w886:u32)
                n499 = Not Equal To 0?(x=w881) -> (x != 0?=w883:bool)
                n500 = case shown="True" w883 {
                  tunnel: w888 -> [w891 w897]
                  tunnel: w887 -> [w890 w896]
                  tunnel: w886 -> [_ w895]
                  tunnel: [w891 w894] -> w885
                  tunnel: w882 -> [_ w892]
                  tunnel: [w890 w893] -> w884
                  frame False {
                  }
                  frame True {
                    n501 = for {
                      shift-right: [w911] -> w894
                      shift-left: w897 -> [w921]
                      shift-right: [w908] -> w893
                      shift-left: w896 -> [w920]
                      tunnel: w895 -> [w919]
                      tunnel: w892 -> [w916] mode=indexing
                      w906 = u16 2 items=["BEAM ENERGY", "EXTRACTOR", "SUPPRESSOR", "CONDENSOR", "OBJECTIVE"] ("HV SUPPLY")
                      w907 = u16 1 items=["BEAM ENERGY", "EXTRACTOR", "SUPPRESSOR", "CONDENSOR", "OBJECTIVE"] ("HV SUPPLY")
                      w914 = u16 0 items=["BEAM ENERGY", "EXTRACTOR", "SUPPRESSOR", "CONDENSOR", "OBJECTIVE"] ("HV SUPPLY")
                      n502 = local read "APPEND"() -> (w903:string)
                      n503 = call "SET HV SUPPLY MEASURE IV.vi"("ORSAY"=w921, "SETTLE"=w919, "HV SUPPLY"=w914, "VOLTAGE"=w916, "ORSAY ERROR"=w920, "APPEND"=w903) -> ("ORSAY 2"=w918:refnum<visa-resource-name>, "ORSAY ERROR"=w917:errorcluster)  [unwired: 8 in]
                      n504 = call "READ HV SUPPLIES.vi"("ORSAY"=w918, "HV SUPPLY"=w914, "ORSAY ERROR"=w917, "APPEND"=w903) -> ("ORSAY 2"=w913:refnum<visa-resource-name>, "VOLTAGE"=w901:dbl[unit], "CURRENT"=w915:dbl[unit], "ORSAY ERROR"=w910:errorcluster)  [unwired: 8 in]
                      n505 = local write "BEAM VOLTAGE"(w901) -> ()
                      n506 = local write "BEAM CURRENT"(w915) -> ()
                      n507 = call "READ HV SUPPLIES.vi"("ORSAY"=w913, "HV SUPPLY"=w907, "ORSAY ERROR"=w910, "APPEND"=w903) -> ("ORSAY 2"=w912:refnum<visa-resource-name>, "VOLTAGE"=w899:dbl[unit], "CURRENT"=w905:dbl[unit], "ORSAY ERROR"=w909:errorcluster)  [unwired: 8 in]
                      n508 = call "READ HV SUPPLIES.vi"("ORSAY"=w912, "HV SUPPLY"=w906, "ORSAY ERROR"=w909, "APPEND"=w903) -> ("ORSAY 2"=w911:refnum<visa-resource-name>, "VOLTAGE"=w900:dbl[unit], "CURRENT"=w904:dbl[unit], "ORSAY ERROR"=w908:errorcluster)  [unwired: 8 in]
                      n509 = Bundle By Name(cluster=T20 {"BEAM"=0.0, "SUPPRESSOR"=0.0, "EXTRACTOR"=0.0} ("HIGH VOLTAGE SUPPLIES"), "BEAM"=w901, "SUPPRESSOR"=w900, "EXTRACTOR"=w899) -> (w902:T20)
                      n510 = local write "HIGH VOLTAGE SUPPLIES"(w902) -> ()
                      n511 = local write "EXTRACTOR  CURRENT"(w905) -> ()
                      n512 = local write "EXTRACTOR"(w899) -> ()
                      n513 = local write "SUPPRESSOR CURRENT"(w904) -> ()
                      n514 = local write "SUPPRESSOR VOLTAGE"(w900) -> ()
                    }
                  }
                }
                n515 = local write "VISA ERROR"(w884) -> ()
                n516 = local write "ORSAY"(w885) -> ()
              }
              frame #2 {
                n517 = property on="SUPPRESSOR" class="Slide (strict)"("DisabledEnum"=T17."Enabled" ("Disabled")) -> ()  [unwired: 2 in, 2 out]
              }
            }
          }
        }
        n518 = local write "PROCESS"(w843) -> ()
        n519 = Build Array (concatenate)(w848, w843) -> (w847:string[])
        n520 = local write "PROCESSES"(w847) -> ()
      }
      frame "ENERGY RAMP CYCLE" {
        n521 = while {
          tunnel: dbl[unit][] [500.0, 1000.0, 1500.0, 2000.0, 2500.0, 3000.0, 3500.0, 4000.0, 4500.0, 5000.0, 4500.0, 4000.0, 3500.0, 3000.0, 2500.0, 2000.0, 1500.0, 1000.0, 500.0, 0.0] -> [w929]
          stop <- w927 continue-if-true
          n522 = local read "VISA ERROR"() -> (w933:errorcluster)
          n523 = local read "TIMER"() -> (w930:u32)
          n524 = local read "ORSAY"() -> (w934:refnum<visa-resource-name>)
          n525 = Array Size(array=w929) -> (size(s)=w928:i32)
          n526 = for {
            N: w928 -> [_]
            shift-right: [w939] -> w932
            shift-left: w934 -> [w946]
            shift-right: [w937] -> w931
            shift-left: w933 -> [w945]
            tunnel: w930 -> [w944]
            tunnel: w929 -> [w935] mode=indexing
            w940 = u16 0 items=["BEAM ENERGY", "EXTRACTOR", "SUPPRESSOR", "CONDENSOR", "OBJECTIVE"] ("HV SUPPLY")
            n527 = local read "APPEND"() -> (w941:string)
            n528 = call "SET HV SUPPLY MEASURE IV.vi"("ORSAY"=w946, "SETTLE"=w944, "HV SUPPLY"=w940, "VOLTAGE"=w935, "ORSAY ERROR"=w945, "APPEND"=w941) -> ("ORSAY 2"=w943:refnum<visa-resource-name>, "ORSAY ERROR"=w942:errorcluster)  [unwired: 8 in]
            n529 = call "READ HV SUPPLIES.vi"("ORSAY"=w943, "HV SUPPLY"=w940, "ORSAY ERROR"=w942, "APPEND"=w941) -> ("ORSAY 2"=w938:refnum<visa-resource-name>, "ORSAY ERROR"=w936:errorcluster)  [unwired: 8 in, 2 out]
            n530 = flat-sequence {
              tunnel: [w948] -> w939
              tunnel: w938 -> [w948]
              tunnel: [w947] -> w937
              tunnel: w936 -> [w947]
              frame #0 {
                n531 = Wait (ms)(milliseconds to wait=u32 100) -> ()  [unwired: 1 out]
              }
            }
          }
          n532 = local read "1V ENERGY RAMP"() -> (w927:bool)
          n533 = local write "ORSAY"(w932) -> ()
          n534 = local write "VISA ERROR"(w931) -> ()
        }
      }
      frame "TURN ON SUPPRESSOR" {
        w951 = "RAMPING UP/DOWN SUPPRESSOR" ("PROCESS")
        n535 = flat-sequence {
          tunnel: [w959] -> w953
          tunnel: [w958] -> w950
          tunnel: w957 -> [w965]
          tunnel: [w964] -> w956
          tunnel: w953 -> [w962]
          tunnel: w950 -> [w961]
          frame #0 {
            n536 = local read "HIGH VOLTAGE SUPPLIES"() -> (w958:cluster{dbl[unit], dbl[unit], dbl[unit]})
            n537 = local read "ION GUN SETTINGS"() -> (w959:T5)
          }
          frame #1 {
            # "New settings"
            n538 = Unbundle(w961) -> (w960:dbl[unit])  [unwired: 2 out]
            n539 = Unbundle By Name(w962) -> ("SUPPRESSOR"=w963:sgl[unit])
            n540 = stacked-sequence {
              tunnel: w963 -> [w967 _ _]
              tunnel: w965 -> [_ w996 _]
              tunnel: w960 -> [w966 _ _]
              tunnel: [_ w996 _] -> w964
              frame #0 {
                # "S-E=Seffective"
                n541 = Subtract(x=w967, y=w966) -> (x-y=w968:dbl[unit])
                n542 = node(w968) -> (w975:dbl)
                n543 = Greater Than 0?(x=w975) -> (x > 0?=w974:bool)
                n544 = case shown="False" w974 {
                  tunnel: [w980 w981] -> w972
                  tunnel: "dV SUPPRESS" -> [w979 w981]
                  frame False {
                    n545 = Negate(x=w979) -> (-x=w980:dbl[unit])
                  }
                  frame True {
                  }
                }
                n546 = Absolute Value(x=w968) -> (abs(x)=w976:dbl[unit])
                n547 = Divide(x=w976, y=w972) -> (x/y=w978:dbl)
                n548 = Absolute Value(x=w978) -> (abs(x)=w971:dbl)
                n549 = To Long Integer(number=w971) -> (32bit integer=w977:i32)
                n550 = for {
                  N: w977 -> [_]
                  tunnel: w972 -> [w986]
                  tunnel: [w984] -> w969 mode=indexing
                  tunnel: w966 -> [w983]
                  i -> [w987]
                  n551 = Increment(x=w987) -> (x+1=w985:i32)
                  n552 = Multiply(x=w986, y=w985) -> (x*y=w982:dbl[unit])
                  n553 = Add(x=w983, y=w982) -> (x+y=w984:dbl[unit])
                }
                "SUPPRESSOR RAMP" <- w969
                n554 = local write "SUPPRESSOR RAMP"(w969) -> ()
                n555 = Array Size(array=w969) -> (size(s)=→"size(s) 4":i32)
              }
              frame #1 {
                n556 = local read "SUPPRESSOR RAMP"() -> (w989:dbl[unit][])
                n557 = Array Size(array=w989) -> (size(s)=w988:i32)
                n558 = local read "VISA ERROR"() -> (w994:errorcluster)
                n559 = local read "ORSAY"() -> (w995:refnum<visa-resource-name>)
                n560 = local read "TIMER"() -> (w993:u32)
                n561 = Not Equal To 0?(x=w988) -> (x != 0?=w990:bool)
                n562 = case shown="True" w990 {
                  tunnel: w995 -> [w998 w1004]
                  tunnel: w994 -> [w997 w1003]
                  tunnel: w993 -> [_ w1002]
                  tunnel: [w998 w1001] -> w992
                  tunnel: w989 -> [_ w999]
                  tunnel: [w997 w1000] -> w991
                  frame False {
                  }
                  frame True {
                    n563 = for {
                      shift-right: [w1013] -> w1001
                      shift-left: w1004 -> [w1028]
                      shift-right: [w1012] -> w1000
                      shift-left: w1003 -> [w1027]
                      tunnel: w1002 -> [w1026]
                      tunnel: w999 -> [w1023] mode=indexing
                      w1014 = u16 1 items=["BEAM ENERGY", "EXTRACTOR", "SUPPRESSOR", "CONDENSOR", "OBJECTIVE"] ("HV SUPPLY")
                      w1018 = u16 0 items=["BEAM ENERGY", "EXTRACTOR", "SUPPRESSOR", "CONDENSOR", "OBJECTIVE"] ("HV SUPPLY")
                      w1022 = u16 2 items=["BEAM ENERGY", "EXTRACTOR", "SUPPRESSOR", "CONDENSOR", "OBJECTIVE"] ("HV SUPPLY")
                      n564 = local read "APPEND"() -> (w1015:string)
                      n565 = call "SET HV SUPPLY MEASURE IV.vi"("ORSAY"=w1028, "SETTLE"=w1026, "HV SUPPLY"=w1022, "VOLTAGE"=w1023, "ORSAY ERROR"=w1027, "APPEND"=w1015) -> ("ORSAY 2"=w1025:refnum<visa-resource-name>, "ORSAY ERROR"=w1024:errorcluster)  [unwired: 8 in]
                      n566 = call "READ HV SUPPLIES.vi"("ORSAY"=w1025, "HV SUPPLY"=w1022, "ORSAY ERROR"=w1024, "APPEND"=w1015) -> ("ORSAY 2"=w1020:refnum<visa-resource-name>, "VOLTAGE"=w1007:dbl[unit], "CURRENT"=w1021:dbl[unit], "ORSAY ERROR"=w1019:errorcluster)  [unwired: 8 in]
                      n567 = local write "SUPPRESSOR CURRENT"(w1021) -> ()
                      n568 = local write "SUPPRESSOR VOLTAGE"(w1007) -> ()
                      n569 = call "READ HV SUPPLIES.vi"("ORSAY"=w1020, "HV SUPPLY"=w1018, "ORSAY ERROR"=w1019, "APPEND"=w1015) -> ("ORSAY 2"=w1017:refnum<visa-resource-name>, "VOLTAGE"=w1009:dbl[unit], "CURRENT"=w1011:dbl[unit], "ORSAY ERROR"=w1016:errorcluster)  [unwired: 8 in]
                      n570 = local write "BEAM CURRENT"(w1011) -> ()
                      n571 = local write "BEAM VOLTAGE"(w1009) -> ()
                      n572 = call "READ HV SUPPLIES.vi"("ORSAY"=w1017, "HV SUPPLY"=w1014, "ORSAY ERROR"=w1016, "APPEND"=w1015) -> ("ORSAY 2"=w1013:refnum<visa-resource-name>, "VOLTAGE"=w1006:dbl[unit], "CURRENT"=w1010:dbl[unit], "ORSAY ERROR"=w1012:errorcluster)  [unwired: 8 in]
                      n573 = local write "EXTRACTOR  CURRENT"(w1010) -> ()
                      n574 = local write "EXTRACTOR"(w1006) -> ()
                      n575 = Bundle By Name(cluster=T20 {"BEAM"=0.0, "SUPPRESSOR"=0.0, "EXTRACTOR"=0.0} ("HIGH VOLTAGE SUPPLIES"), "BEAM"=w1009, "SUPPRESSOR"=w1007, "EXTRACTOR"=w1006) -> (w1008:T20)
                      n576 = local write "HIGH VOLTAGE SUPPLIES"(w1008) -> ()
                    }
                  }
                }
                n577 = local write "VISA ERROR"(w991) -> ()
                n578 = local write "ORSAY"(w992) -> ()
              }
              frame #2 {
                n579 = property on="EXTRACTOR" class="Slide (strict)"("DisabledEnum"=T17."Enabled" ("Disabled")) -> ()  [unwired: 2 in, 2 out]
              }
            }
          }
        }
        n580 = local write "PROCESS"(w951) -> ()
        n581 = Build Array (concatenate)(w955, w951) -> (w954:string[])
        n582 = local write "PROCESSES"(w954) -> ()
      }
      frame "TURN ON EXTRACTOR" {
        w1031 = "RAMPING UP/DOWN SUPPRESSOR" ("PROCESS")
        n583 = flat-sequence {
          tunnel: [w1039] -> w1033
          tunnel: [w1038] -> w1030
          tunnel: w1037 -> [w1046]
          tunnel: [w1045] -> w1036
          tunnel: w1033 -> [w1043]
          tunnel: w1030 -> [w1042]
          frame #0 {
            n584 = local read "HIGH VOLTAGE SUPPLIES"() -> (w1038:cluster{dbl[unit], dbl[unit], dbl[unit]})
            n585 = local read "ION GUN SETTINGS"() -> (w1039:T5)
          }
          frame #1 {
            # "New settings"
            n586 = Unbundle By Name(w1043) -> ("EXTRACTOR"=w1044:sgl[unit])
            n587 = Unbundle(w1042) -> (w1041:dbl[unit], w1040:dbl[unit])  [unwired: 1 out]
            n588 = stacked-sequence {
              tunnel: w1044 -> [w1048 _ _]
              tunnel: w1046 -> [_ w1077 _]
              tunnel: w1040 -> [w1047 _ _]
              tunnel: [_ w1077 _] -> w1045
              tunnel: w1041 -> [_ _ _]
              frame #0 {
                n589 = Subtract(x=w1048, y=w1047) -> (x-y=w1054:dbl[unit])
                n590 = node(w1054) -> (w1056:dbl)
                n591 = Greater Than 0?(x=w1056) -> (x > 0?=w1055:bool)
                n592 = case shown="False" w1055 {
                  tunnel: [w1061 w1062] -> w1052
                  tunnel: "dV EXTRACTOR" -> [w1060 w1062]
                  frame False {
                    n593 = Negate(x=w1060) -> (-x=w1061:dbl[unit])
                  }
                  frame True {
                  }
                }
                n594 = Absolute Value(x=w1054) -> (abs(x)=w1057:dbl[unit])
                n595 = Divide(x=w1057, y=w1052) -> (x/y=w1059:dbl)
                n596 = Absolute Value(x=w1059) -> (abs(x)=w1051:dbl)
                n597 = To Long Integer(number=w1051) -> (32bit integer=w1058:i32)
                n598 = for {
                  N: w1058 -> [_]
                  tunnel: w1052 -> [w1067]
                  tunnel: [w1065] -> w1049 mode=indexing
                  tunnel: w1047 -> [w1064]
                  i -> [w1068]
                  n599 = Increment(x=w1068) -> (x+1=w1066:i32)
                  n600 = Multiply(x=w1067, y=w1066) -> (x*y=w1063:dbl[unit])
                  n601 = Add(x=w1064, y=w1063) -> (x+y=w1065:dbl[unit])
                }
                n602 = local write "EXTRACTOR RAMP"(w1049) -> ()
                n603 = local write "EXTRACTOR RAMP"(w1049) -> ()
                n604 = Array Size(array=w1049) -> (size(s)=→"size(s) 5":i32)
              }
              frame #1 {
                n605 = local read "EXTRACTOR RAMP"() -> (w1069:dbl[unit][])
                n606 = Array Size(array=w1069) -> (size(s)=w1070:i32)
                n607 = local read "VISA ERROR"() -> (w1075:errorcluster)
                n608 = local read "ORSAY"() -> (w1076:refnum<visa-resource-name>)
                n609 = local read "TIMER"() -> (w1074:u32)
                n610 = Not Equal To 0?(x=w1070) -> (x != 0?=w1071:bool)
                n611 = case shown="True" w1071 {
                  tunnel: w1076 -> [w1079 w1085]
                  tunnel: w1075 -> [w1078 w1084]
                  tunnel: w1074 -> [_ w1083]
                  tunnel: [w1079 w1082] -> w1073
                  tunnel: w1069 -> [_ w1080]
                  tunnel: [w1078 w1081] -> w1072
                  frame False {
                  }
                  frame True {
                    n612 = for {
                      shift-right: [w1098] -> w1082
                      shift-left: w1085 -> [w1109]
                      shift-right: [w1096] -> w1081
                      shift-left: w1084 -> [w1108]
                      tunnel: w1083 -> [w1107]
                      tunnel: w1080 -> [w1104] mode=indexing
                      w1093 = u16 0 items=["BEAM ENERGY", "EXTRACTOR", "SUPPRESSOR", "CONDENSOR", "OBJECTIVE"] ("HV SUPPLY")
                      w1094 = u16 2 items=["BEAM ENERGY", "EXTRACTOR", "SUPPRESSOR", "CONDENSOR", "OBJECTIVE"] ("HV SUPPLY")
                      w1103 = u16 1 items=["BEAM ENERGY", "EXTRACTOR", "SUPPRESSOR", "CONDENSOR", "OBJECTIVE"] ("HV SUPPLY")
                      n613 = local read "APPEND"() -> (w1095:string)
                      n614 = call "SET HV SUPPLY MEASURE IV.vi"("ORSAY"=w1109, "SETTLE"=w1107, "HV SUPPLY"=w1103, "VOLTAGE"=w1104, "ORSAY ERROR"=w1108, "APPEND"=w1095) -> ("ORSAY 2"=w1106:refnum<visa-resource-name>, "ORSAY ERROR"=w1105:errorcluster)  [unwired: 8 in]
                      n615 = call "READ HV SUPPLIES.vi"("ORSAY"=w1106, "HV SUPPLY"=w1103, "ORSAY ERROR"=w1105, "APPEND"=w1095) -> ("ORSAY 2"=w1101:refnum<visa-resource-name>, "VOLTAGE"=w1087:dbl[unit], "CURRENT"=w1102:dbl[unit], "ORSAY ERROR"=w1100:errorcluster)  [unwired: 8 in]
                      n616 = local write "EXTRACTOR"(w1087) -> ()
                      n617 = local write "EXTRACTOR  CURRENT"(w1102) -> ()
                      n618 = call "READ HV SUPPLIES.vi"("ORSAY"=w1101, "HV SUPPLY"=w1093, "ORSAY ERROR"=w1100, "APPEND"=w1095) -> ("ORSAY 2"=w1099:refnum<visa-resource-name>, "VOLTAGE"=w1090:dbl[unit], "CURRENT"=w1091:dbl[unit], "ORSAY ERROR"=w1097:errorcluster)  [unwired: 8 in]
                      n619 = local write "BEAM CURRENT"(w1091) -> ()
                      n620 = local write "BEAM VOLTAGE"(w1090) -> ()
                      n621 = call "READ HV SUPPLIES.vi"("ORSAY"=w1099, "HV SUPPLY"=w1094, "ORSAY ERROR"=w1097, "APPEND"=w1095) -> ("ORSAY 2"=w1098:refnum<visa-resource-name>, "VOLTAGE"=w1088:dbl[unit], "CURRENT"=w1092:dbl[unit], "ORSAY ERROR"=w1096:errorcluster)  [unwired: 8 in]
                      n622 = Bundle By Name(cluster=T20 {"BEAM"=0.0, "SUPPRESSOR"=0.0, "EXTRACTOR"=0.0} ("HIGH VOLTAGE SUPPLIES"), "BEAM"=w1090, "SUPPRESSOR"=w1088, "EXTRACTOR"=w1087) -> (w1089:T20)
                      n623 = local write "HIGH VOLTAGE SUPPLIES"(w1089) -> ()
                      n624 = local write "SUPPRESSOR CURRENT"(w1092) -> ()
                      n625 = local write "SUPPRESSOR VOLTAGE"(w1088) -> ()
                    }
                  }
                }
                n626 = local write "VISA ERROR"(w1072) -> ()
                n627 = local write "ORSAY"(w1073) -> ()
              }
              frame #2 {
                n628 = property on="EXTRACTOR" class="Slide (strict)"("DisabledEnum"=T17."Enabled" ("Disabled")) -> ()  [unwired: 2 in, 2 out]
              }
            }
          }
        }
        n629 = local write "PROCESS"(w1031) -> ()
        n630 = Build Array (concatenate)(w1035, w1031) -> (w1034:string[])
        n631 = local write "PROCESSES"(w1034) -> ()
      }
      frame "TURN OFF WOBBLER" {
        n632 = flat-sequence {
          frame #0 {
            n633 = local read "APPEND"() -> (w1123:string)
            n634 = Concatenate Strings("WB 0" ("string"), w1123) -> (w1115:string)
            n635 = local read "VISA ERROR"() -> (w1124:errorcluster)
            n636 = local read "ORSAY"() -> (w1125:refnum<visa-resource-name>)
            n637 = VISA Write(VISA resource name=w1125, write buffer=w1115, error in (no error)=w1124) -> (VISA resource name out=w1119:refnum<visa-resource-name>, error out=w1118:errorcluster)  [unwired: 1 out]
            n638 = flat-sequence {
              tunnel: w1119 -> [w1128]
              tunnel: [w1130] -> w1116
              tunnel: w1118 -> [w1130]
              tunnel: [w1128] -> w1117
              frame #0 {
                n639 = Wait (ms)(milliseconds to wait=u32 100) -> ()  [unwired: 1 out]
              }
            }
            n640 = property class="Instr"(reference=w1117, error in=w1116) -> (reference out=w1120:refnum<visa-resource-name>, error out=w1122:errorcluster, "Serial Settings:Number of Bytes at Serial Port"=w1121:u32)
            n641 = VISA Read(VISA resource name=w1120, byte count=w1121, error in (no error)=w1122) -> (VISA resource name out=w1127:refnum<visa-resource-name>, error out=w1126:errorcluster)  [unwired: 2 out]
            n642 = local write "ORSAY"(w1127) -> ()
            n643 = local write "VISA ERROR"(w1126) -> ()
          }
          frame #1 {
          }
        }
      }
      frame "STOP SYSTEM" {
        n644 = flat-sequence {
          frame #0 {
            n645 = local read "VISA ERROR"() -> (w1134:errorcluster)
            n646 = local read "ORSAY"() -> (w1135:refnum<visa-resource-name>)
            n647 = VISA Close(VISA resource name=w1135, error in (no error)=w1134) -> ()  [unwired: 1 out]
          }
          frame #1 {
            n648 = Stop(stop? (T)=TRUE) -> ()
          }
        }
      }
      frame "MEASURE HV SUPPLY VOLTAGES" {
        w1153 = u16 4 items=["BEAM ENERGY", "EXTRACTOR", "SUPPRESSOR", "CONDENSOR", "OBJECTIVE"] ("HV SUPPLY")
        w1154 = u16 3 items=["BEAM ENERGY", "EXTRACTOR", "SUPPRESSOR", "CONDENSOR", "OBJECTIVE"] ("HV SUPPLY")
        w1157 = u16 2 items=["BEAM ENERGY", "EXTRACTOR", "SUPPRESSOR", "CONDENSOR", "OBJECTIVE"] ("HV SUPPLY")
        w1158 = u16 1 items=["BEAM ENERGY", "EXTRACTOR", "SUPPRESSOR", "CONDENSOR", "OBJECTIVE"] ("HV SUPPLY")
        w1159 = u16 0 items=["BEAM ENERGY", "EXTRACTOR", "SUPPRESSOR", "CONDENSOR", "OBJECTIVE"] ("HV SUPPLY")
        w1169 = "MEASURING ION GUN HV" ("PROCESS")
        n649 = local read "ORSAY"() -> (w1164:refnum<visa-resource-name>)
        n650 = local read "APPEND"() -> (w1149:string)
        n651 = call "READ HV SUPPLIES.vi"("ORSAY"=w1164, "HV SUPPLY"=w1159, "APPEND"=w1149) -> ("ORSAY 2"=w1161:refnum<visa-resource-name>, "VOLTAGE"=w1146:dbl[unit], "CURRENT"=→"BEAM CURRENT" →"CURRENT":dbl[unit], "ORSAY ERROR"=w1163:errorcluster)  [unwired: 9 in]
        "BEAM VOLTAGE" <- w1146
        "VOLTAGE" <- w1146
        n652 = call "READ HV SUPPLIES.vi"("ORSAY"=w1161, "HV SUPPLY"=w1158, "ORSAY ERROR"=w1163, "APPEND"=w1149) -> ("ORSAY 2"=w1160:refnum<visa-resource-name>, "VOLTAGE"=w1138:dbl[unit], "CURRENT"=→"EXTRACTOR  CURRENT" →"CURRENT":dbl[unit], "ORSAY ERROR"=w1162:errorcluster)  [unwired: 8 in]
        "EXTRACTOR" <- w1138
        "VOLTAGE" <- w1138
        n653 = call "READ HV SUPPLIES.vi"("ORSAY"=w1160, "HV SUPPLY"=w1157, "ORSAY ERROR"=w1162, "APPEND"=w1149) -> ("ORSAY 2"=w1156:refnum<visa-resource-name>, "VOLTAGE"=w1137:dbl[unit], "CURRENT"=→"SUPPRESSOR CURRENT" →"CURRENT":dbl[unit], "ORSAY ERROR"=w1150:errorcluster)  [unwired: 8 in]
        "SUPPRESSOR VOLTAGE" <- w1137
        "VOLTAGE" <- w1137
        n654 = local write "PROCESS"(w1169) -> ()
        n655 = Build Array (concatenate)(w1168, w1169) -> (w1167:string[])
        n656 = call "READ HV SUPPLIES.vi"("ORSAY"=w1156, "HV SUPPLY"=w1154, "ORSAY ERROR"=w1150, "APPEND"=w1149) -> ("ORSAY 2"=w1155:refnum<visa-resource-name>, "VOLTAGE"=→"CONDENSOR VOLTAGE":dbl[unit], "CURRENT"=→"CONDENSOR CURRENT":dbl[unit], "ORSAY ERROR"=w1151:errorcluster)  [unwired: 8 in]
        n657 = Bundle By Name(cluster=T20 {"BEAM"=0.0, "SUPPRESSOR"=0.0, "EXTRACTOR"=0.0} ("HIGH VOLTAGE SUPPLIES"), "BEAM"=w1146, "SUPPRESSOR"=w1137, "EXTRACTOR"=w1138) -> (→"HIGH VOLTAGE SUPPLIES":T20)
        n658 = local write "PROCESSES"(w1167) -> ()
        n659 = call "READ HV SUPPLIES.vi"("ORSAY"=w1155, "HV SUPPLY"=w1153, "ORSAY ERROR"=w1151, "APPEND"=w1149) -> ("ORSAY 2"=w1152:refnum<visa-resource-name>, "VOLTAGE"=→"OBJECTIVE VOLTAGE":dbl[unit], "CURRENT"=→"OBJECTIVE CURRENT":dbl[unit])  [unwired: 8 in, 1 out]
        n660 = local write "ORSAY"(w1152) -> ()
      }
      frame "SCANNING CONTROLS" {
        w1174 = "SCANNING CONTROL" ("PROCESS")
        n661 = Unbundle By Name("SCANNING CLUSTER") -> ("X-OFFSET"=w1200:sgl[unit], "Y-OFFSET"=w1199:sgl[unit], "ROTATION"=w1198:dbl[unit])  [unwired: 1 out]
        n662 = node(w1200) -> (w1196:sgl)
        n663 = node(w1199) -> (w1193:sgl)
        n664 = node(w1198) -> (w1192:dbl)
        n665 = local read "ORSAY"() -> (w1178:refnum<visa-resource-name>)
        n666 = call "conversion data to bits.vi"("Data input"=w1196, "Max supply"=sgl 30000.0) -> ("15 bits output"=w1191:u16)  [unwired: 1 in, 1 out]
        n667 = call "conversion data to bits.vi"("Data input"=w1193, "Max supply"=sgl 12000.0) -> ("15 bits output"=w1190:u16)  [unwired: 1 in, 1 out]
        n668 = call "conversion data to bits.vi"("Data input"=w1192, "Max supply"=sgl 2000.0) -> ("15 bits output"=w1189:u16)  [unwired: 1 in, 1 out]
        n669 = Number To Hexadecimal String(2:w1191) -> (0:w1188:string)  [unwired: 1 in]
        n670 = Number To Hexadecimal String(2:w1190) -> (0:w1185:string)  [unwired: 1 in]
        n671 = Number To Hexadecimal String(2:w1189) -> (0:w1184:string)  [unwired: 1 in]
        n672 = local read "APPEND"() -> (w1172:string)
        n673 = Concatenate Strings("XX  ", w1188, w1172) -> (w1183:string)
        n674 = Concatenate Strings("XX  ", w1185, w1172) -> (w1182:string)
        n675 = local write "PROCESS"(w1174) -> ()
        n676 = Concatenate Strings("XX ", w1184, w1172) -> (w1181:string)
        n677 = Build Array (concatenate)(w1175, w1174) -> (w1173:string[])
        n678 = Build Array(w1183, w1182, w1181) -> (w1177:string[])
        n679 = for {
          tunnel: w1177 -> [w1213] mode=indexing
          shift-right: [w1212] -> w1179
          shift-left: w1178 -> [w1214]
          shift-right: [w1202] -> w1170
          shift-left: w1176 -> [w1203]
          n680 = VISA Write(VISA resource name=w1214, write buffer=w1213) -> (VISA resource name out=w1209:refnum<visa-resource-name>, error out=w1208:errorcluster)  [unwired: 1 in, 1 out]
          n681 = flat-sequence {
            tunnel: w1209 -> [w1215]
            tunnel: [w1217] -> w1206
            tunnel: w1208 -> [w1217]
            tunnel: [w1215] -> w1207
            frame #0 {
              n682 = Wait (ms)(milliseconds to wait=u32 100) -> ()  [unwired: 1 out]
            }
          }
          n683 = property class="Instr"(reference=w1207, error in=w1206) -> (reference out=w1211:refnum<visa-resource-name>, error out=w1205:errorcluster, "Serial Settings:Number of Bytes at Serial Port"=w1210:u32)
          n684 = VISA Read(VISA resource name=w1211, byte count=w1210, error in (no error)=w1205) -> (VISA resource name out=w1212:refnum<visa-resource-name>, read buffer=w1204:string)  [unwired: 2 out]
          n685 = Build Array (concatenate)(w1203, w1204) -> (w1202:string[])
          n686 = local write "SERIAL \nRESPONSE"(w1202) -> ()
        }
        n687 = local write "PROCESSES"(w1173) -> ()
        n688 = local write "ORSAY"(w1179) -> ()
      }
      frame "SAVE SETTINGS" {
        n689 = stacked-sequence {
          seq-local: [w1225 _] -> [_ w1330]
          seq-local: [w1224 _] -> [_ w1329]
          frame #0 {
            w1259 = "FIB SETTINGS" ("channel name")
            n690 = local read "STIGMATOR"() -> (w1223:T11)
            n691 = local read "ION GUN SETTINGS"() -> (w1302:T5)
            n692 = local read "STIGMATOR X & Y"() -> (w1285:cluster{"X":sgl, "Y":sgl})
            n693 = local read "CONDENSOR"() -> (w1286:cluster{"COARSE":sgl[unit], "FINE":sgl[unit]})
            n694 = local read "OBJECTIVE"() -> (w1287:cluster{"COARSE":sgl[unit], "FINE":sgl[unit]})
            n695 = Unbundle By Name(w1223) -> ("STIG ALIGN"=w1222:cluster{"+X":sgl, "-X":sgl, "+Y":sgl, "-Y":sgl})
            n696 = local read "COLUMN VACUUM"() -> (w1228:dbl[unit])
            n697 = Unbundle By Name(w1302) -> ("BEAM ENERGY"=w1280:sgl[unit], "EXTRACTOR"=w1256:sgl[unit], "SUPPRESSOR"=w1255:sgl[unit], "ION CURRENT"=w1254:sgl[unit])
            n698 = Unbundle By Name(w1287) -> ("COARSE"=w1279:sgl[unit], "FINE"=w1272:sgl[unit])
            n699 = local read "BEAM CURRENT (FC1)"() -> (w1229:dbl[unit])
            n700 = Unbundle By Name(w1286) -> ("COARSE"=w1271:sgl[unit], "FINE"=w1270:sgl[unit])
            n701 = Unbundle By Name(w1285) -> ("X"=w1269:sgl, "Y"=w1268:sgl)
            n702 = Unbundle By Name(w1222) -> ("+X"=w1238:sgl, "-X"=w1237:sgl, "+Y"=w1236:sgl, "-Y"=w1235:sgl)
            n703 = To Variant(anything=w1238) -> (Variant=w1234:variant)
            n704 = To Variant(anything=w1237) -> (Variant=w1233:variant)
            n705 = To Variant(anything=w1236) -> (Variant=w1232:variant)
            n706 = To Variant(anything=w1235) -> (Variant=w1231:variant)
            n707 = call "File Dialog"() -> ("selected path"=w1304:path, "error out"=w1283:errorcluster)  [unwired: 12 in, 2 out]
            n708 = node(w1271) -> (w1248:sgl)
            n709 = node(w1270) -> (w1247:sgl)
            n710 = node(w1280) -> (w1257:sgl)
            n711 = node(w1256) -> (w1251:sgl)
            n712 = node(w1255) -> (w1252:sgl)
            n713 = node(w1254) -> (w1253:sgl)
            n714 = node(w1279) -> (w1250:sgl)
            n715 = node(w1272) -> (w1249:sgl)
            n716 = TDMS Open(8:w1283, 10:T22."create or replace" ("operation (0:open)"), 11:w1304) -> (0:w1282:errorcluster, 3:w1284:refnum<k34>)  [unwired: 4 in]
            n717 = To Variant(anything=w1257) -> (Variant=w1278:variant)
            n718 = To Variant(anything=w1251) -> (Variant=w1277:variant)
            n719 = To Variant(anything=w1252) -> (Variant=w1276:variant)
            n720 = node(w1229) -> (w1221:dbl)
            n721 = To Variant(anything=w1253) -> (Variant=w1275:variant)
            n722 = To Variant(anything=w1250) -> (Variant=w1274:variant)
            n723 = To Variant(anything=w1249) -> (Variant=w1267:variant)
            n724 = To Variant(anything=w1248) -> (Variant=w1266:variant)
            n725 = To Variant(anything=w1247) -> (Variant=w1265:variant)
            n726 = To Variant(anything=w1269) -> (Variant=w1264:variant)
            n727 = To Variant(anything=w1268) -> (Variant=w1263:variant)
            n728 = node(w1228) -> (w1227:dbl)
            n729 = To Variant(anything=w1221) -> (Variant=w1230:variant)
            n730 = To Variant(anything=w1227) -> (Variant=w1226:variant)
            n731 = local read "SCANNING CLUSTER"() -> (w1246:T13)
            n732 = Build Array(w1278, w1277, w1276, w1275, w1274, w1267, w1266, w1265, w1264, w1263, w1234, w1233, w1232, w1231, w1230, w1226) -> (w1273:variant[])
            n733 = for {
              tunnel: T21 ["BEAM ENERGY", "EXTRACTOR", "SUPRESSOR", "ION CURRENT", "OBJ COARSE", "OBJ FINE", "COND COARSE", "COND FINE", "STIGX", "STIGY", "STIG+X", "STIG-X", "STIG+Y", "STIG-Y", "PROBE CURRENT", "COLUMN VACUUM"] -> [w1320] mode=indexing
              shift-right: [w1322] -> w1258
              shift-left: w1282 -> [w1318]
              tunnel: w1273 -> [w1316] mode=indexing
              tunnel: w1259 -> [w1315]
              tunnel: "ORSAY COLUMN" -> [w1314]
              shift-right: [w1321] -> w1261
              shift-left: w1284 -> [w1323]
              n734 = call <userlib>:"Set Data Name__ogtk.vi"("error in (no error)"=w1318, "Data Name"=w1320, "Data"=w1316) -> ("error out"=w1317:errorcluster, "Renamed Data"=w1319:variant)  [unwired: 7 in]
              n735 = TDMS Set Properties(5:w1319, 7:w1320, 8:w1317, 9:w1314, 10:w1315, 11:w1323) -> (0:w1322:errorcluster, 3:w1321:refnum<k34>)  [unwired: 2 out]
            }
            n736 = Get Date/Time String() -> (date string=w1290:string, time string=w1291:string)  [unwired: 3 in]
            n737 = Unbundle By Name(w1246) -> ("X-OFFSET"=w1242:sgl[unit], "Y-OFFSET"=w1241:sgl[unit], "ROTATION"=w1240:dbl[unit], "MAGNIFICATION"=w1239:dbl)  [unwired: 1 out]
            n738 = To Variant(anything=0) -> (Variant=w1292:variant)
            n739 = To Variant(anything="NAME") -> (Variant=w1295:variant)
            n740 = To Variant(anything="USER") -> (Variant=w1296:variant)
            n741 = To Variant(anything=w1290) -> (Variant=w1297:variant)
            n742 = To Variant(anything=w1291) -> (Variant=w1298:variant)
            n743 = To Variant(anything="COMMENT") -> (Variant=w1300:variant)
            n744 = Build Array(w1292, w1295, w1296, w1297, w1298, w1300) -> (w1301:variant[])
            n745 = for {
              shift-right: [w1312] -> w1224
              shift-left: w1258 -> [w1310]
              tunnel: string[] ["RUN ID", "USER ID", "DATE", "TIME", "COMMENTS"] ("property names") -> [w1307] mode=indexing
              tunnel: "RUN DETAILS" ("channel name") -> [w1308]
              tunnel: w1301 -> [w1306] mode=indexing
              tunnel: w1259 -> [w1305]
              shift-right: [w1311] -> w1225
              shift-left: w1261 -> [w1313]
              n746 = call <userlib>:"Set Data Name__ogtk.vi"("Data Name"=w1307, "Data"=w1306) -> ("Renamed Data"=w1309:variant)  [unwired: 8 in, 1 out]
              n747 = TDMS Set Properties(5:w1309, 7:w1307, 8:w1310, 9:w1308, 10:w1305, 11:w1313) -> (0:w1312:errorcluster, 3:w1311:refnum<k34>)  [unwired: 2 out]
            }
            n748 = node(w1242) -> (w1245:sgl)
            n749 = node(w1241) -> (w1243:sgl)
            n750 = node(w1240) -> (w1244:dbl)
            n751 = To Variant(anything=w1245) -> ()  [unwired: 1 out]
            n752 = To Variant(anything=w1243) -> ()  [unwired: 1 out]
            n753 = To Variant(anything=w1244) -> ()  [unwired: 1 out]
            n754 = To Variant(anything=w1239) -> ()  [unwired: 1 out]
          }
          frame #1 {
            n755 = local read "OBJECT APERTURE POSITIONS"() -> (w1324:cluster{"NAME":string, "Xo":dbl, "Yo":dbl}[])
            n756 = for {
              tunnel: "APERTURE SETTINGS" ("channel name") -> [w1353]
              tunnel: "FIB SETTINGS" ("channel name") -> [w1352]
              shift-right: [w1349] -> w1328
              shift-left: w1330 -> [w1351]
              shift-right: [w1348] -> w1327
              shift-left: w1329 -> [w1350]
              tunnel: w1324 -> [w1345] mode=indexing
              tunnel: "X" -> [w1343]
              tunnel: "Y" -> [w1341]
              i -> [w1347]
              n757 = Unbundle By Name(w1345) -> ("NAME"=w1344:string, "Xo"=w1337:dbl, "Yo"=w1336:dbl)
              n758 = Number To Decimal String(number=w1347, width (-)=i16 0) -> (decimal integer string=w1342:string)
              n759 = Concatenate Strings(w1344, w1342, w1343) -> (w1340:string)
              n760 = Concatenate Strings(w1344, w1342, w1341) -> (w1339:string)
              n761 = To Variant(anything=w1337) -> (Variant=w1335:variant)
              n762 = To Variant(anything=w1336) -> (Variant=w1334:variant)
              n763 = Build Array(w1340, w1339) -> (w1338:string[])
              n764 = Build Array(w1335, w1334) -> (w1333:variant[])
              n765 = for {
                shift-right: [w1361] -> w1348
                shift-left: w1350 -> [w1359]
                tunnel: w1338 -> [w1356] mode=indexing
                tunnel: w1353 -> [w1357]
                tunnel: w1352 -> [w1355]
                shift-right: [w1360] -> w1349
                shift-left: w1351 -> [w1362]
                tunnel: w1333 -> [w1354] mode=indexing
                n766 = call <userlib>:"Set Data Name__ogtk.vi"("Data Name"=w1356, "Data"=w1354) -> ("Renamed Data"=w1358:variant)  [unwired: 8 in, 1 out]
                n767 = TDMS Set Properties(5:w1358, 7:w1356, 8:w1359, 9:w1357, 10:w1355, 11:w1362) -> (0:w1361:errorcluster, 3:w1360:refnum<k34>)  [unwired: 2 out]
              }
            }
            n768 = TDMS Close(8:w1327, 11:w1328) -> ()  [unwired: 2 out]
          }
        }
      }
      frame "READ SETTINGS" {
        (unwired) 2 ("index")
        (unwired) 1 ("index")
        w1410 = "FIB SETTINGS" ("group name")
        (unwired) string[] ["BEAM ENERGY", "EXTRACTOR", "SUPRESSOR", "ION CURRENT", "OBJ COARSE", "OBJ FINE", "COND COARSE", "COND FINE", "STIGX", "STIGY", "SCAN TYPE", "X-OFFSET", "Y-OFFSET", "ROTATION", "MAGNIFICATION", "STIG+X", "STIG-X", "STIG+Y", "STIG-Y", "PROBE CURRENT", "COLUMN VACUUM"]
        n769 = TDMS Open(11:"FIB SETUP FILE") -> (0:w1415:errorcluster, 3:w1414:refnum<k34>)  [unwired: 6 in]
        n770 = TDMS List Contents(4:w1415, 6:w1410, 7:w1414) -> (1:w1409:string[], 3:w1413:refnum<k34>)  [unwired: 2 out]
        n771 = Index Array(array=w1409, index=0) -> (element=w1407:string)
        n772 = TDMS Get Properties(9:w1407, 10:w1410, 11:w1413) -> (0:w1411:errorcluster, 3:w1412:refnum<k34>, 4:w1369:variant[])  [unwired: 3 in, 3 out]
        n773 = Delete From Array(array=w1369, length=1, index=0) -> (array with subset deleted=w1366:variant[])  [unwired: 1 out]
        n774 = for {
          tunnel: w1366 -> [w1419] mode=indexing
          tunnel: [w1418] -> w1404 mode=indexing
          n775 = Variant To Data(type=sgl 0.0, Variant=w1419) -> (data=w1418:sgl)  [unwired: 1 in, 1 out]
        }
        n776 = TDMS Close(8:w1411, 11:w1412) -> ()  [unwired: 2 out]
        n777 = Index Array(array=w1404, index #1=0 ("index"), index #2=1 ("index"), index #3=2 ("index"), index #4=3 ("index"), index #5=4 ("index"), index #6=5 ("index"), index #7=6 ("index"), index #8=7 ("index"), index #9=8 ("index"), index #10=9 ("index")) -> (element #1=w1403:sgl, element #2=w1402:sgl, element #3=w1401:sgl, element #4=w1400:sgl, element #5=w1387:sgl, element #6=w1386:sgl, element #7=w1385:sgl, element #8=w1384:sgl, element #9=w1371:sgl, element #10=w1370:sgl)  [unwired: 4 in, 4 out]
        n778 = node(w1403) -> (w1399:sgl[unit])
        n779 = node(w1402) -> (w1398:sgl[unit])
        n780 = node(w1401) -> (w1397:sgl[unit])
        n781 = node(w1400) -> (w1396:sgl[unit])
        n782 = node(w1387) -> (w1395:sgl[unit])
        n783 = node(w1386) -> (w1394:sgl[unit])
        n784 = node(w1385) -> (w1393:sgl[unit])
        n785 = node(w1384) -> (w1392:sgl[unit])
        n786 = local read "STIGMATOR X & Y"() -> (w1373:cluster{"X":sgl, "Y":sgl})
        n787 = local read "ION GUN SETTINGS"() -> (w1406:T5)
        n788 = Bundle By Name(cluster=w1406, "BEAM ENERGY"=w1399, "EXTRACTOR"=w1398, "SUPPRESSOR"=w1397, "ION CURRENT"=w1396) -> (w1405:T5)
        n789 = local read "CONDENSOR"() -> (w1390:cluster{"COARSE":sgl[unit], "FINE":sgl[unit]})
        n790 = Bundle By Name(cluster=w1390, "COARSE"=w1393, "FINE"=w1392) -> (w1389:cluster{"COARSE":sgl[unit], "FINE":sgl[unit]})
        n791 = local read "OBJECTIVE"() -> (w1391:cluster{"COARSE":sgl[unit], "FINE":sgl[unit]})
        n792 = Bundle By Name(cluster=w1391, "COARSE"=w1395, "FINE"=w1394) -> (w1388:cluster{"COARSE":sgl[unit], "FINE":sgl[unit]})
        n793 = Bundle By Name(cluster=w1373, "X"=w1371, "Y"=w1370) -> (w1372:cluster{"X":sgl, "Y":sgl})
        n794 = local write "STIGMATOR X & Y"(w1372) -> ()
        n795 = local write "OBJECTIVE"(w1388) -> ()
        n796 = local write "CONDENSOR"(w1389) -> ()
        n797 = local write "ION GUN SETTINGS"(w1405) -> ()
      }
      frame "BLANKING TOGGLE" {
        w1426 = "BLANKING MODE" ("PROCESS")
        n798 = local read "BEAM ON"() -> (w1427:bool)
        n799 = case shown="False" w1427 {
          tunnel: [w1429 w1449] -> w1424
          frame False {
            n800 = local read "APPEND"() -> (w1428:string)
            n801 = local read "VISA ERROR"() -> (w1440:errorcluster)
            n802 = Concatenate Strings("BL 0,1", "," ("string"), "0" ("string"), w1428) -> (w1430:string)
            n803 = local read "ORSAY"() -> (w1441:refnum<visa-resource-name>)
            n804 = VISA Write(VISA resource name=w1441, write buffer=w1430, error in (no error)=w1440) -> (VISA resource name out=w1437:refnum<visa-resource-name>, error out=w1435:errorcluster)  [unwired: 1 out]
            n805 = flat-sequence {
              tunnel: [w1447] -> w1436
              tunnel: w1437 -> [w1447]
              tunnel: [w1446] -> w1434
              tunnel: w1435 -> [w1446]
              frame #0 {
                n806 = Wait (ms)(milliseconds to wait=u32 200) -> ()  [unwired: 1 out]
              }
            }
            n807 = property class="Instr"(reference=w1436, error in=w1434) -> (reference out=w1444:refnum<visa-resource-name>, error out=w1442:errorcluster, "Serial Settings:Number of Bytes at Serial Port"=w1443:u32)
            n808 = VISA Read(VISA resource name=w1444, byte count=w1443, error in (no error)=w1442) -> (VISA resource name out=w1439:refnum<visa-resource-name>, read buffer=w1429:string, error out=w1438:errorcluster)  [unwired: 1 out]
            n809 = local write "VISA ERROR"(w1438) -> ()
            n810 = local write "ORSAY"(w1439) -> ()
          }
          frame True {
            n811 = local read "BLANKING CONTROL"() -> (w1452:u16)
            n812 = local read "APPEND"() -> (w1448:string)
            n813 = Concatenate Strings("BL 0,0\nBL 1,1\nBL 2,0", w1448) -> (w1451:string)
            n814 = local read "VISA ERROR"() -> (w1460:errorcluster)
            n815 = Pick Line(multi-line string=w1451, line index=w1452) -> (output string=w1457:string)  [unwired: 1 in]
            n816 = local read "ORSAY"() -> (w1461:refnum<visa-resource-name>)
            n817 = VISA Write(VISA resource name=w1461, write buffer=w1457, error in (no error)=w1460) -> (VISA resource name out=w1456:refnum<visa-resource-name>, error out=w1454:errorcluster)  [unwired: 1 out]
            n818 = flat-sequence {
              tunnel: [w1467] -> w1455
              tunnel: w1456 -> [w1467]
              tunnel: [w1466] -> w1453
              tunnel: w1454 -> [w1466]
              frame #0 {
                n819 = Wait (ms)(milliseconds to wait=u32 100) -> ()  [unwired: 1 out]
              }
            }
            n820 = property class="Instr"(reference=w1455, error in=w1453) -> (reference out=w1464:refnum<visa-resource-name>, error out=w1462:errorcluster, "Serial Settings:Number of Bytes at Serial Port"=w1463:u32)
            n821 = VISA Read(VISA resource name=w1464, byte count=w1463, error in (no error)=w1462) -> (VISA resource name out=w1459:refnum<visa-resource-name>, read buffer=w1449:string, error out=w1458:errorcluster)  [unwired: 1 out]
            n822 = local write "ORSAY"(w1459) -> ()
            n823 = local write "VISA ERROR"(w1458) -> ()
          }
        }
        n824 = Build Array (concatenate)(w1425, w1426) -> (w1422:string[])
        n825 = local write "PROCESS"(w1426) -> ()
        n826 = Build Array (concatenate)(w1423, w1424) -> (w1420:string[])
        n827 = local write "SERIAL \nRESPONSE"(w1420) -> ()
        n828 = local write "PROCESSES"(w1422) -> ()
      }
      frame "SET STIGMATOR" {
        w1471 = "ADJUSTING STIGMATOR" ("PROCESS")
        n829 = local read "VISA ERROR"() -> (w1477:errorcluster)
        n830 = local read "ORSAY"() -> (w1484:refnum<visa-resource-name>)
        n831 = call "CENTER STIGMATOR.vi"("STIGMATOR"="STIGMATOR") -> ("STIGMATOR COMMAND"=w1478:string)  [unwired: 5 in]
        n832 = VISA Write(VISA resource name=w1484, write buffer=w1478, error in (no error)=w1477) -> (VISA resource name out=w1479:refnum<visa-resource-name>, error out=w1481:errorcluster)  [unwired: 1 out]
        n833 = property class="Instr"(reference=w1479, error in=w1481) -> (reference out=w1480:refnum<visa-resource-name>, error out=w1482:errorcluster, "Serial Settings:Number of Bytes at Serial Port"=w1483:u32)
        n834 = local write "PROCESS"(w1471) -> ()
        n835 = Build Array (concatenate)(w1472, w1471) -> (w1470:string[])
        n836 = VISA Read(VISA resource name=w1480, byte count=w1483, error in (no error)=w1482) -> (VISA resource name out=w1476:refnum<visa-resource-name>, read buffer=w1474:string, error out=w1475:errorcluster)  [unwired: 1 out]
        n837 = local write "PROCESSES"(w1470) -> ()
        n838 = local write "ORSAY"(w1476) -> ()
        n839 = local write "VISA ERROR"(w1475) -> ()
        n840 = Build Array (concatenate)(w1473, w1474) -> (w1468:string[])
        n841 = local write "SERIAL \nRESPONSE"(w1468) -> ()
      }
      frame "SET WOBBLER FOR OBJECT" {
        n842 = local read "WOBBLER SETTINBGS FOR OBJECT ALIGNMENT"() -> (w1489:T9)
        n843 = Unbundle By Name(w1489) -> ()  [unwired: 2 out]
      }
      frame "DEFINE NEW OBJ" {
        n844 = local read "OBJECT APERTURE POSITIONS"() -> (w1500:cluster{"NAME":string, "Xo":dbl, "Yo":dbl}[])
        n845 = property on="OBJECT APERTURE" class="Ring (strict)"() -> ("RingText.Text"=w1498:string)  [unwired: 2 in, 2 out]
        n846 = local read "Xo"() -> (w1497:dbl)
        n847 = local read "Yo"() -> (w1496:dbl)
        n848 = Index Array(array=w1500, index=0) -> (element=w1499:cluster{"NAME":string, "Xo":dbl, "Yo":dbl})
        n849 = Bundle By Name(cluster=w1499, "NAME"=w1498, "Xo"=w1497, "Yo"=w1496) -> (w1495:cluster{"NAME":string, "Xo":dbl, "Yo":dbl})
        n850 = local read "OBJECT APERTURE"() -> (w1501:u16)
        n851 = Replace Array Subset(array=w1500, new element=w1495, index=w1501) -> (w1494:cluster{"NAME":string, "Xo":dbl, "Yo":dbl}[])
        n852 = local write "OBJECT APERTURE POSITIONS"(w1494) -> ()
      }
      frame "DEFINE NEW APERTURE" {
        n853 = local read "MASS APERTURE POSITIONS"() -> (w1512:cluster{"NAME":string, "Xa":dbl, "Ya":dbl}[])
        n854 = property on="APERTURE (MASS)" class="Ring (strict)"() -> ("RingText.Text"=w1505:string)  [unwired: 2 in, 2 out]
        n855 = local read "Xa"() -> (w1510:dbl)
        n856 = local read "Ya"() -> (w1509:dbl)
        n857 = Index Array(array=w1512, index=0) -> (element=w1511:cluster{"NAME":string, "Xa":dbl, "Ya":dbl})
        n858 = Bundle By Name(cluster=w1511, "NAME"=w1505, "Xa"=w1510, "Ya"=w1509) -> (w1508:cluster{"NAME":string, "Xa":dbl, "Ya":dbl})
        n859 = local read "APERTURE (MASS)"() -> (w1513:u16)
        n860 = Replace Array Subset(array=w1512, new element=w1508, index=w1513) -> (w1507:cluster{"NAME":string, "Xa":dbl, "Ya":dbl}[])
        n861 = local write "MASS APERTURE POSITIONS"(w1507) -> ()
      }
      frame "INITIALISE PI MOTORS" {
        n862 = local read "ENABLE APERTURES"() -> (w1514:bool)
        n863 = case shown="True" w1514 {
          frame False {
          }
          frame True {
            # "Stage names input"
            # "TRUE: All axes can be moved"
            n864 = local read "STAGE AXES"() -> (w1523:string[])
            n865 = local write "INIT PI"(FALSE ("INIT PI")) -> ()
            n866 = call "C843_Configuration_Setup.vi"("System no."=1, "C-843 Board No."=1, "Axes to move"=w1523, "All axes?"=TRUE, "C-843 version"=TRUE, "Use dialog to define\nconnected stages?"=FALSE ("Use dialog to define\nconnected stages?"), "Stage names input"=string[] ["FIBSTAGE", "FIBSTAGE", "FIBSTAGE", "FIBSTAGE"], "Limit switch selection"="HOME ON LIMIT", "RON Affected axes"=w1523, "Reference mode"=bool[] [TRUE, TRUE, TRUE, TRUE]) -> ("Identification"=w1529:string, "Position"=→"POSITIONS":dbl[], "+/- movement\nrange"=→"RANGE":dbl[], "error out"=w1527:errorcluster)  [unwired: 5 in, 1 out]
            n867 = Select(t="NONE", s=w1527, f=w1529) -> (s? t:f=w1528:string)
            n868 = Unbundle By Name(w1527) -> ("status"=→"NO CONTROLLER":bool)
            n869 = Concatenate Strings("DETECTED CONTROLLER:", w1528) -> (w1531:string)
            n870 = local write "PROCESS"(w1531) -> ()
          }
        }
      }
      frame "READ APERTURE POSITIONS" {
        w1540 = FALSE ("All axes?")
        w1539 = 1 ("System no.")
        n871 = local read "STAGE AXES"() -> (w1541:string[])
        n872 = call "FRF?.vi"("System no."=w1539, "Axes to query"=w1541, "All axes?"=w1540) -> ("Referenced?"=w1537:bool[], "error out"=w1544:errorcluster)  [unwired: 2 in, 13 out]
        n873 = call "POS?.vi"("System no."=w1539, "Axes to query"=w1541, "All axes?"=w1540, "error in"=w1544) -> ("Position"=w1542:dbl[], "error out"=w1543:errorcluster)  [unwired: 1 in, 13 out]
        n874 = Build Array (concatenate)(w1547, "READING APERTURES") -> (w1546:string[])
        n875 = local write "REFERENCED"(w1537) -> ()
        n876 = local write "POSITIONS"(w1542) -> ()
        n877 = Build Array (concatenate)(w1550, "") -> (w1549:string[])
        n878 = call "RON?.vi"("System no."=w1539, "Axes to query"=w1541, "All axes?"=w1540, "error in"=w1543) -> ("Reference on?"=w1538:bool[])  [unwired: 1 in, 14 out]
        n879 = local write "ON TRARGET"(w1538) -> ()
      }
      frame "HOME OBJ & AP STAGES" {
      }
      frame "SET OBJ & AP STAGE VELOCITIES" {
        w1560 = string[] ["Xo", "Yo", "Xa", "Ya"] ("Axes to move")
        # "um/s"
        n880 = call "VEL.vi"("System no."=1, "Axes to set"=w1560, "Velocity values"=dbl[] [1000.0, 1000.0, 1000.0, 1000.0], "No.of digits"=i16 4, "Without axis ID?"=FALSE) -> ("error out"=w1562:errorcluster)  [unwired: 1 in, 13 out]
        n881 = call "VEL?.vi"("System no."=1, "Axes to query"=w1560, "All axes?"=TRUE, "error in"=w1562) -> ("Velocity"=→"VELOCITIES":dbl[])  [unwired: 1 in, 14 out]
        n882 = local write "PROCESS"("SETTING OBJ & APERTURE VELOCITIES" ("channel name")) -> ()
      }
      frame "MOVE OBJ STAGES" {
        w1573 = string[] ["Xo", "Yo"] ("Axes to move")
        n883 = local read "OBJECT APERTURE POSITIONS"() -> (w1585:cluster{"NAME":string, "Xo":dbl, "Yo":dbl}[])
        n884 = local read "OBJECT APERTURE"() -> (w1584:u16)
        n885 = Index Array(array=w1585, index=w1584) -> (element=w1583:cluster{"NAME":string, "Xo":dbl, "Yo":dbl})
        n886 = Unbundle By Name(w1583) -> ("Xo"=w1582:dbl, "Yo"=w1581:dbl)
        n887 = Build Array(w1582, w1581) -> (w1580:dbl[])
        n888 = call "MOV.vi"("System no."=1, "Axes to move"=w1573, "Position values"=w1580) -> ("error out"=w1586:errorcluster)  [unwired: 2 in, 14 out]
        n889 = call "MOV?.vi"("System no."=1, "Axes to query"=w1573, "All axes?"=TRUE, "error in"=w1586) -> ("Target position"=w1579:dbl[])  [unwired: 1 in, 14 out]
        n890 = Index Array(array=w1579, index #1=0 ("index"), index #2=1 ("index")) -> (element #1=w1578:dbl, element #2=w1577:dbl)
        n891 = local write "Xo"(w1578) -> ()
        n892 = local write "Yo"(w1577) -> ()
      }
      frame "MOVE APERTURE STAGES" {
        w1588 = string[] ["1", "2"] ("Axes to move")
        w1587 = 1 ("System no.")
        n893 = local read "MASS APERTURE POSITIONS"() -> (w1596:cluster{"NAME":string, "Xa":dbl, "Ya":dbl}[])
        n894 = local read "APERTURE (MASS)"() -> (w1595:u16)
        n895 = Index Array(array=w1596, index=w1595) -> (element=w1604:cluster{"NAME":string, "Xa":dbl, "Ya":dbl})
        n896 = Unbundle By Name(w1604) -> ("Xa"=w1603:dbl, "Ya"=w1602:dbl)
        n897 = Build Array(w1603, w1602) -> (w1601:dbl[])
        n898 = call "MOV.vi"("System no."=w1587, "Axes to move"=w1588, "Position values"=w1601) -> ("error out"=w1605:errorcluster)  [unwired: 2 in, 14 out]
        n899 = call "MOV?.vi"("System no."=w1587, "Axes to query"=w1588, "All axes?"=TRUE, "error in"=w1605) -> ("Target position"=w1600:dbl[], "error out"=w1589:errorcluster)  [unwired: 1 in, 13 out]
        n900 = while {
          tunnel: w1588 -> [w1607]
          tunnel: w1587 -> [w1610]
          shift-right: [w1606] -> _
          shift-left: w1589 -> [w1611]
          stop <- w1614 stop-if-true
          w1608 = FALSE ("All axes?")
          n901 = call "POS?.vi"("System no."=w1610, "Axes to query"=w1607, "All axes?"=w1608, "error in"=w1611) -> ("error out"=w1609:errorcluster)  [unwired: 1 in, 14 out]
          n902 = call "ONT?.vi"("System no."=w1610, "Axes to query"=w1607, "All axes?"=w1608, "error in"=w1609) -> ("Axis on target?"=w1613:bool[], "error out"=w1606:errorcluster)  [unwired: 1 in, 13 out]
          "ON TRARGET" <- w1613
          n903 = Index Array(array=w1613, index #1=0 ("index"), index #2=1 ("index")) -> (element #1=w1615:bool, element #2=w1616:bool)
          n904 = Wait (ms)(milliseconds to wait=u32 100) -> ()  [unwired: 1 out]
          n905 = And(x=w1615, y=w1616) -> (x .and. y?=w1614:bool)
        }
        n906 = Index Array(array=w1600, index #1=0 ("index"), index #2=1 ("index")) -> (element #1=w1594:dbl, element #2=w1593:dbl)
        n907 = local write "Xa"(w1594) -> ()
        n908 = local write "Ya"(w1593) -> ()
      }
    }
  }
  n909 = while {
    shift-right: [w1620] -> _
    shift-left: w11 -> [w1622]
    stop <- TRUE continue-if-true
    n910 = Dequeue Element(queue=w1622) -> (queue out=w1620:refnum<queue>, element=w1621:enum16{"INIT DAQ", "STOP TASKS"})  [unwired: 2 in, 2 out]
    n911 = case shown="\"STOP TASKS\"" w1621 {
      frame "INIT DAQ", Default {
      }
      frame "STOP TASKS" {
      }
    }
  }
  n912 = while {
    shift-right: [w1624] -> _
    shift-left: w23 -> [w1627]
    stop <- w1625 stop-if-true
    n913 = Dequeue Element(queue=w1627) -> (queue out=w1624:refnum<queue>, element=w1626:T16)  [unwired: 2 in, 2 out]
    n914 = case shown="True" "ENABLE CAMERA" {
      tunnel: w1626 -> [_ w1628]
      frame False {
      }
      frame True {
        n915 = case shown="\"INIT VIDEO\"" w1628 {
          frame "LOOP", Default {
            n916 = local read "FIB SAMPLE CAMERA"() -> (w1630:T2)
            n917 = local read "FIB CAMERA ERROR"() -> (w1631:errorcluster)
            n918 = local read "FIB CAMERA"() -> (w1632:T3)
            n919 = property on="ANGLE" class="DigNum (strict)"("Visible"="ROTATE VIEW") -> ()  [unwired: 2 in, 2 out]
            n920 = call <vilib>:"IMAQdx Get Image2.vi"("Timeout (ms)"=500, "Buffer Number Mode (Next)"=IMAQdx_Buffer_Number_Mode."Last New", "error in"=w1631, "Image In"=w1632, "Session In"=w1630) -> ("error out"=w1642:errorcluster, "Image Out"=w1643:T3)  [unwired: 3 in, 2 out]
            n921 = case shown="True" "ROTATE VIEW" {
              tunnel: w1643 -> [w1657 w1661]
              tunnel: w1642 -> [w1656 w1660]
              tunnel: [w1656 w1659] -> w1637
              tunnel: [w1657 w1658] -> w1638
              frame False {
              }
              frame True {
                n922 = call "IMAQ Rotate"("error in (no error)"=w1660, "Angle (degrees)"="ANGLE", "Image Src"=w1661) -> ("error out"=w1659:errorcluster, "Image Dst Out"=w1658:T3)  [unwired: 7 in]
              }
            }
            n923 = case shown="False" "SYMMETRY" {
              tunnel: w1638 -> [w1664 w1669]
              tunnel: w1637 -> [w1663 w1668]
              tunnel: "IMAGE SYMMETRY" -> [_ w1667]
              tunnel: [w1664 w1666] -> w1644
              tunnel: [w1663 w1665] -> w1645
              frame False {
              }
              frame True {
                n924 = call "IMAQ Symmetry"("error in (no error)"=w1668, "Type of Symmetry"=w1667, "Image Src"=w1669) -> ("error out"=w1665:errorcluster, "Image Dst Out"=w1666:T3)  [unwired: 2 in]
              }
            }
            n925 = property on="BRIGHT,CONT,GAMMA" class="Clust (strict)"("Visible"="REFLECTIVITY") -> ()  [unwired: 2 in, 2 out]
            n926 = case shown="True" "REFLECTIVITY" {
              tunnel: w1644 -> [w1647 w1651]
              tunnel: [w1647 w1653] -> w1629
              tunnel: "BRIGHT,CONT,GAMMA" -> [_ w1652]
              tunnel: w1645 -> [w1646 w1650]
              tunnel: [w1646 w1648] -> _
              frame False {
              }
              frame True {
                w1655 = T28 0 items=["Grayscale (U8)", "Grayscale (I16)", "Grayscale (SGL)", "Complex (CSG)", "RGB (U32)", "HSL (U32)", "RGB (U64)", "Grayscale (U16)"] ("Image Type")
                n927 = call "IMAQ Cast Image"("Image Type"=w1655, "error in (no error)"=w1650, "Image Src"=w1651) -> ("error out"=w1649:errorcluster, "Image Dst Out"=w1654:T3)  [unwired: 7 in]
                n928 = call "IMAQ BCGLookup"("Image Src"=w1654, "BCG Values"=w1652, "error in (no error)"=w1649) -> ("Image Dst Out"=w1653:T3, "error out"=w1648:errorcluster)  [unwired: 4 in]
              }
            }
            n929 = local write "FIB CAMERA"(w1629) -> ()
          }
          frame "INIT VIDEO" {
            w1676 = T28 4 items=["Grayscale (U8)", "Grayscale (I16)", "Grayscale (SGL)", "Complex (CSG)", "RGB (U32)", "HSL (U32)", "RGB (U64)", "Grayscale (U16)"] ("Image Type")
            w1679 = 2.0
            w1707 = 2.0
            w1706 = sgl 0.95 ("x")
            n930 = call <vilib>:"IMAQdx Open Camera.vi"("Camera Control Mode"=IMAQdx_Camera_Control_Mode."Controller", "Session In"=T2 "MAKO") -> ("error out"=w1704:errorcluster, "Session Out"=w1705:T2)  [unwired: 8 in]
            n931 = call <vilib>:"IMAQdx Enumerate Attributes.vi"("error in"=w1704, "Session In"=w1705) -> ("error out"=w1700:errorcluster, "Session Out"=w1701:T2)  [unwired: 7 in, 1 out]
            n932 = property class="IMAQdx"(reference=w1701, error in=w1700) -> (reference out=w1699:T2, error out=w1698:errorcluster, "ActualPeakBandwidth"=→"ActualPeakBandwidth":dbl)
            n933 = property class="IMAQdx"(reference=w1699, error in=w1698) -> (reference out=w1673:T2, error out=w1672:errorcluster, "IPAddress"=→"IP ADDRESS":string, "Width"=w1671:u32, "Height"=w1670:u32)
            "IMAGE XPIXELS" <- w1671
            "IMAGE YPIXELS" <- w1670
            n934 = Multiply(x=w1671, y=w1706) -> (x*y=w1710:sgl)
            n935 = Multiply(x=w1670, y=w1706) -> (x*y=w1709:sgl)
            n936 = To Double Precision Float(number=w1671) -> (double precision float=w1712:dbl)
            n937 = To Double Precision Float(number=w1670) -> (double precision float=w1713:dbl)
            n938 = Bundle(w1710, w1709) -> ()  [unwired: 1 in, 1 out]
            n939 = Divide(x=w1713, y=w1707) -> (x/y=→"IMAGE YCENTRE":dbl)
            n940 = Divide(x=w1712, y=w1707) -> (x/y=→"IMAGE XCENTRE":dbl)
            n941 = call <vilib>:"IMAQdx Configure Grab.vi"("error in"=w1672, "Session In"=w1673) -> ("error out"=w1686:errorcluster, "Session Out"=w1687:T2)  [unwired: 8 in]
            n942 = case shown="False" FALSE {
              tunnel: w1687 -> [w1717 w1721]
              tunnel: [w1717 w1720] -> w1696
              tunnel: w1686 -> [w1716 w1719]
              tunnel: [w1716 w1718] -> w1697
              frame False {
              }
              frame True {
                n943 = call <vilib>:"IMAQdx Read Attributes.vi"("error in"=w1719, "Session In"=w1721) -> ("error out"=w1718:errorcluster, "Session Out"=w1720:T2)  [unwired: 8 in]
              }
            }
            n944 = Divide(x=w1671, y=w1679) -> (x/y=w1688:dbl)
            n945 = Divide(x=w1670, y=w1679) -> (x/y=w1689:dbl)
            n946 = To Long Integer(number=w1688) -> (32bit integer=w1690:i32)
            n947 = To Long Integer(number=w1689) -> (32bit integer=w1691:i32)
            n948 = Subtract(x=w1690, y=3) -> (x-y=w1693:i32)
            n949 = call <vilib>:"IMAQdx Start Acquisition.vi"("error in"=w1697, "Session In"=w1696) -> ("error out"=→"FIB CAMERA ERROR":errorcluster, "Session Out"=→"FIB SAMPLE CAMERA":T2)  [unwired: 8 in]
            n950 = Subtract(x=w1691, y=2) -> (x-y=w1692:i32)
            n951 = call "IMAQ Create"("Image Name"="TARGET", "Image Type"=w1676, "error in (no error)"=w1697) -> ("New Image"=w1684:T3, "error out"=w1695:errorcluster)  [unwired: 2 in]
            n952 = Bundle(w1693, w1692) -> (w1694:cluster{i32, i32})  [unwired: 1 in]
            "CENTRE CAMERA FOV" <- w1694
            n953 = call "IMAQ Overlay Bitmap"("Group"="FEATURES", "error in (no error)"=w1695, "Bitmap"=u32[][] [[16777216, 16777216, 16777216, 16777216, 16777216, 16777216, 16777216, 16777216, 16777216, 16777216, 16777216, 12189440, 16777216, 16777216, 16777216, 16777216, 16777216, 16777216, 16777216, 16777216, 16777216, 16777216, 16777216], [16777216, 16777216, 16777216, 16777216, 16777216, 16777216, 16777216, 16777216, 16777216, 16777216, 16777216, 12189440, 16777216, 16777216, 16777216, 16777216, 16777216, 16777216, 16777216, 16777216, 16777216, 16777216, 16777216], [16777216, 16777216, 16777216, 16777216, 16777216, 16777216, 16777216, 16777216, 16777216, 16777216, 15859456, 12189440, 15859456, 16777216, 16777216, 16777216, 16777216, 16777216, 16777216, 16777216, 16777216, 16777216, 16777216], [16777216, 16777216, 16777216, 16777216, 16777216, 16777216, 16777216, 16777216, 16777216, 16777216, 15859456, 12189440, 15859456, 16777216, 16777216, 16777216, 16777216, 16777216, 16777216, 16777216, 16777216, 16777216, 16777216], [16777216, 16777216, 16777216, 16777216, 16777216, 16777216, 16777216, 16777216, 16777216, 16777216, 15859456, 12189440, 15859456, 16777216, 16777216, 16777216, 16777216, 16777216, 16777216, 16777216, 16777216, 16777216, 16777216], [16777216, 16777216, 16777216, 16777216, 16777216, 16777216, 16777216, 16777216, 16777216, 16777216, 15859456, 12189440, 15859456, 16777216, 16777216, 16777216, 16777216, 16777216, 16777216, 16777216, 16777216, 16777216, 16777216], [16777216, 16777216, 16777216, 16777216, 16777216, 16777216, 16777216, 16777216, 16777216, 16777216, 15859456, 12189440, 15859456, 16777216, 16777216, 16777216, 16777216, 16777216, 16777216, 16777216, 16777216, 16777216, 16777216], [16777216, 16777216, 16777216, 16777216, 16777216, 16777216, 16777216, 16777216, 16777216, 16777216, 16777216, 12189440, 16777216, 16777216, 16777216, 16777216, 16777216, 16777216, 16777216, 16777216, 16777216, 16777216, 16777216], [16777216, 16777216, 16777216, 16777216, 16777216, 16777216, 16777216, 16777216, 12189440, 16777216, 16777216, 12189440, 16777216, 16777216, 12189440, 16777216, 16777216, 16777216, 16777216, 16777216, 16777216, 16777216, 16777216], [16777216, 16777216, 16777216, 16777216, 16777216, 16777216, 16777216, 16777216, 16777216, 12189440, 16777216, 12189440, 16777216, 12189440, 16777216, 16777216, 16777216, 16777216, 16777216, 16777216, 16777216, 16777216, 16777216], [16777216, 16777216, 15859456, 15859456, 15859456, 15859456, 15859456, 16777216, 16777216, 16777216, 16777216, 12189440, 16777216, 16777216, 16777216, 16777216, 15859456, 15859456, 15859456, 15859456, 15859456, 16777216, 16777216], [12189440, 12189440, 12189440, 12189440, 12189440, 12189440, 12189440, 12189440, 12189440, 12189440, 12189440, 12189440, 12189440, 12189440, 12189440, 12189440, 12189440, 12189440, 12189440, 12189440, 12189440, 12189440, 12189440], [16777216, 16777216, 15859456, 15859456, 15859456, 15859456, 15859456, 16777216, 16777216, 16777216, 16777216, 12189440, 16777216, 16777216, 16777216, 16777216, 15859456, 15859456, 15859456, 15859456, 15859456, 16777216, 16777216], [16777216, 16777216, 16777216, 16777216, 16777216, 16777216, 16777216, 16777216, 16777216, 12189440, 16777216, 12189440, 16777216, 12189440, 16777216, 16777216, 16777216, 16777216, 16777216, 16777216, 16777216, 16777216, 16777216], [16777216, 16777216, 16777216, 16777216, 16777216, 16777216, 16777216, 16777216, 12189440, 16777216, 16777216, 12189440, 16777216, 16777216, 12189440, 16777216, 16777216, 16777216, 16777216, 16777216, 16777216, 16777216, 16777216], [16777216, 16777216, 16777216, 16777216, 16777216, 16777216, 16777216, 16777216, 16777216, 16777216, 16777216, 12189440, 16777216, 16777216, 16777216, 16777216, 16777216, 16777216, 16777216, 16777216, 16777216, 16777216, 16777216], [16777216, 16777216, 16777216, 16777216, 16777216, 16777216, 16777216, 16777216, 16777216, 16777216, 15859456, 12189440, 15859456, 16777216, 16777216, 16777216, 16777216, 16777216, 16777216, 16777216, 16777216, 16777216, 16777216], [16777216, 16777216, 16777216, 16777216, 16777216, 16777216, 16777216, 16777216, 16777216, 16777216, 15859456, 12189440, 15859456, 16777216, 16777216, 16777216, 16777216, 16777216, 16777216, 16777216, 16777216, 16777216, 16777216], [16777216, 16777216, 16777216, 16777216, 16777216, 16777216, 16777216, 16777216, 16777216, 16777216, 15859456, 12189440, 15859456, 16777216, 16777216, 16777216, 16777216, 16777216, 16777216, 16777216, 16777216, 16777216, 16777216], [16777216, 16777216, 16777216, 16777216, 16777216, 16777216, 16777216, 16777216, 16777216, 16777216, 15859456, 12189440, 15859456, 16777216, 16777216, 16777216, 16777216, 16777216, 16777216, 16777216, 16777216, 16777216, 16777216], [16777216, 16777216, 16777216, 16777216, 16777216, 16777216, 16777216, 16777216, 16777216, 16777216, 15859456, 12189440, 15859456, 16777216, 16777216, 16777216, 16777216, 16777216, 16777216, 16777216, 16777216, 16777216, 16777216], [16777216, 16777216, 16777216, 16777216, 16777216, 16777216, 16777216, 16777216, 16777216, 16777216, 16777216, 12189440, 16777216, 16777216, 16777216, 16777216, 16777216, 16777216, 16777216, 16777216, 16777216, 16777216, 16777216], [16777216, 16777216, 16777216, 16777216, 16777216, 16777216, 16777216, 16777216, 16777216, 16777216, 16777216, 12189440, 16777216, 16777216, 16777216, 16777216, 16777216, 16777216, 16777216, 16777216, 16777216, 16777216, 16777216]], "Top Left Point"=w1694, "Image"=w1684) -> ("Image Out"=w1685:T3)  [unwired: 5 in, 1 out]
            n954 = local write "FIB CAMERA"(w1685) -> ()
          }
          frame "CAMERA GAIN" {
            n955 = local read "FIB SAMPLE CAMERA"() -> (w1724:T2)
            n956 = local read "FIB CAMERA ERROR"() -> (w1723:errorcluster)
            n957 = property class="IMAQdx"(reference=w1724, error in=w1723, "ActiveAttribute"="GainAuto") -> (reference out=w1731:T2, error out=w1732:errorcluster)
            n958 = property class="IMAQdx"(reference=w1731, error in=w1732, "ValueU32"="GAIN METHOD") -> (reference out=w1733:T2, error out=w1734:errorcluster)
            n959 = property class="IMAQdx"(reference=w1733, error in=w1734, "ActiveAttribute"="GainRaw") -> (reference out=w1728:T2, error out=w1729:errorcluster)
            n960 = property class="IMAQdx"(reference=w1728, error in=w1729, "ValueDBL"="GAIN") -> (reference out=w1725:T2, error out=w1722:errorcluster)
            n961 = local write "FIB SAMPLE CAMERA"(w1725) -> ()
            n962 = local write "FIB CAMERA ERROR"(w1722) -> ()
          }
          frame "CAMERA EXPOSURE" {
            n963 = local read "FIB SAMPLE CAMERA"() -> (w1739:T2)
            n964 = local read "FIB CAMERA ERROR"() -> (w1738:errorcluster)
            n965 = property class="IMAQdx"(reference=w1739, error in=w1738, "ActiveAttribute"="ExposureAuto") -> (reference out=w1743:T2, error out=w1742:errorcluster)
            n966 = property class="IMAQdx"(reference=w1743, error in=w1742, "ValueU32"=u32 1) -> (reference out=w1752:T2, error out=w1753:errorcluster)
            n967 = case shown="0, Default" "CONFIGS" {
              tunnel: [w1768 20.0 ("EXPOSURE TIME") 5.0 ("EXPOSURE TIME")] -> w1751
              tunnel: "EXPOSURE" -> [w1768 _ _]
              frame 0, Default {
              }
              frame 1 {
              }
              frame 2 {
              }
            }
            n968 = local write "EXPOSURE"(w1751) -> ()
            n969 = Multiply(x=1000.0, y=w1751) -> (x*y=w1754:dbl)
            n970 = case shown="True" TRUE {
              tunnel: w1752 -> [w1759 w1766]
              tunnel: w1753 -> [w1758 w1765]
              tunnel: w1754 -> [_ w1762]
              tunnel: [w1759 w1761] -> w1741
              tunnel: [w1758 w1760] -> w1740
              frame False {
              }
              frame True {
                n971 = property class="IMAQdx"(reference=w1766, error in=w1765, "ActiveAttribute"="ExposureTimeAbs") -> (reference out=w1764:T2, error out=w1763:errorcluster)
                n972 = property class="IMAQdx"(reference=w1764, error in=w1763, "ValueDBL"=w1762) -> (reference out=w1761:T2, error out=w1760:errorcluster)
              }
            }
            n973 = property class="IMAQdx"(reference=w1741, error in=w1740, "ActiveAttribute"="GainAuto") -> (reference out=w1755:T2, error out=w1756:errorcluster)
            n974 = property class="IMAQdx"(reference=w1755, error in=w1756, "ValueU32"=u32 2) -> (reference out=w1737:T2, error out=w1736:errorcluster)
            n975 = local write "FIB SAMPLE CAMERA"(w1737) -> ()
            n976 = local write "FIB CAMERA ERROR"(w1736) -> ()
          }
        }
      }
    }
    n977 = local read "STOP"() -> (w1625:bool)
  }
  n978 = case shown="True" FALSE {
    frame False {
    }
    frame True {
      n979 = call "MNL.vi"() -> ()  [unwired: 5 in, 15 out]
      n980 = call "MPL.vi"() -> ()  [unwired: 5 in, 15 out]
      n981 = call "VEL.vi"() -> ()  [unwired: 6 in, 14 out]
      n982 = call "VEL?.vi"() -> ()  [unwired: 5 in, 15 out]
      n983 = call "TMN?.vi"() -> ()  [unwired: 5 in, 15 out]
      n984 = call "LIM?.vi"() -> ()  [unwired: 5 in, 15 out]
      n985 = call "GOH.vi"() -> ()  [unwired: 5 in, 15 out]
      n986 = call "TMX?.vi"() -> ()  [unwired: 5 in, 15 out]
    }
  }
